vi "BIMS_Collector (2010_08).vi"() -> ()   [LabVIEW 2015]
doc: "This program is currently beta software. It is designed to address the data requirements defined primarily by the DHB Ballistic Test Report.\n\nThe general operation of this program is based on the Ballistics Version 2005 application developed internally by DuPont as a research tool for the Spruance Plant Ballistics Lab in Richmond, VA.\n\nPlease note that the original trigger control logic was modified and no longer depends on a safety interlock system to enable operation of a ballistic test.\n\nDuPont makes no warranties and assumes no liabilities in connection with any use of this program."
uses:
  <vilib>/addons/database/NI_Database_API.lvlib
  <vilib>/addons/database/Connection.llb/Conn Execute.vi
  <vilib>/addons/database/Recordset.llb/Rec Destroy - Connection.vi
  <vilib>/Utility/config.llb/NI_LVConfig.lvlib
  <vilib>/Utility/config.llb/Write Key (I32).vi
  Shot Record.ctl
  BIMS_Collector Globals.vi
  Collector State.ctl
  DataSource.ctl
  <vilib>/registry/registry.llb/Registry RtKey.ctl
  <vilib>/Utility/config.llb/Write Key (String).vi
  <vilib>/addons/database/Connection.llb/DB Tools Open Connec (Path).vi
panel:
  out "Loading":u16(ring)
  in  "runtimeMenusVisible":bool=TRUE
  in  "diagPageVisible":bool
  in  "RESET All":bool
  out "ConfigName":string
  out "TimeNow":string
  in  "EXIT":bool
  in  "mainTabCntrl":enum32{"Setup", "Measure", "History", "System"}(tab)=enum."System"
  in  "SampleEntryTabCntrl":enum32{"Environment", "Sample"}(tab)
  in  "ThreatDetails":u16(ring) caption="Detail"
  in  "ThreatGroups":u16(ring) caption="Group" items=["", "RCC"]
  in  "PowderTypes":u16(ring) caption="Type"
  in  "Ballisticians":u16(ring) caption="Ballistician"
  in  "Recorders":u16(ring) caption="Recorder"
  in  "Shooters":u16(ring) caption="Shooter"
  in  "Methods":u16(ring) caption="Method"
  in  "RoomT":sgl caption="Temperature (° F)" format="%.1f"
  in  "RoomHum":sgl caption="Humidity (%)" min=0 max=100 format="%.1f"
  in  "SampleBackings":u16(ring)=3 caption="Type"
  in  "clayCalArray":i16[](array[numeric])=[0, 0, 0, 0, 0] caption="Calibration (mm)" min=0 max=99 format="%02.0f"
  out "clayAverage":sgl caption="Clay Average (mm)" format="%#.1f"
  in  "clayTemp":sgl caption="Clay Temp (° F)" format="%.1f"
  out "threatDetails":T1 caption="Description"
  in  "SampleClamping":u16(ring) caption="Clamping"
  in  "Sample SubTabCntrl":T2(tab)
  in  "SampleID":string caption="Sample ID"
  in  "SampleDimensions":u16(ring) caption="Dimensions"
  in  "ModelMfrs":u16(ring) caption="Manufacturer" items=["DuPont Experimental"]
  in  "SampleTypes":u16(ring) caption="Sample Type"
  in  "Submitters":u16(ring) caption="Submitter"
  in  "ProjectID":string caption="Project ID"
  in  "BackLayers":i32 caption="# of Layers" min=0 max=99 step=5
  in  "FrontLayers":i32 caption="# of Layers" min=0 max=99 step=5
  in  "BackLayer":u16(ring) caption="Back Layer"
  in  "FrontLayer":u16(ring) caption="Front Layer"
  out "totalNumLayers":i32 caption="Total # of Layers" min=0 max=100 step=5
  out "totalBAW":sgl caption="Total BAW (psf)" format="%.2f"
  in  "LayerTabControl":enum32{"1", "2", "3", "4", "5", "6"}(tab) caption="Inner Layers"
  out "fab1_totalWt":sgl caption="Fab1 Wt" min=0 max=99 step=5 format="%.2f"
  out "SampleAttribs_1":T3 caption="fabricAttribs_1"
  in  "Layer_1":T4 caption="Fabric #1" {"plyNum" min=0 max=99 step=5}
  in  "SampleStyle_1":u16(ring) items=["", "S-706G"]
  in  "Mfr_1":u16(ring) caption="vendor" items=["", "DuPont"]
  in  "layerStitch_1":u16(ring) caption="Stitch" items=["", "1-inch quilt", "2-inch quilt", "Corner Bartack", "Corners", "Custom (Panel)", "Custom (Vest)", "Diamond", "Edge", "n/a", "Normal"]
  out "fab2_totalWt":sgl caption="Fab2 Wt" min=0 max=99 step=5 format="%.2f"
  out "SampleAttribs_2":T3 caption="fabricAttribs_2"
  in  "Layer_2":T4 caption="Fabric #2" {"plyNum" min=0 max=99 step=5}
  in  "SampleStyle_2":u16(ring)
  in  "Mfr_2":u16(ring) caption="vendor" items=["", "DuPont"]
  in  "layerStitch_2":u16(ring) caption="Stitch" items=["", "1-inch quilt", "2-inch quilt", "Corner Bartack", "Corners", "Custom (Panel)", "Custom (Vest)", "Diamond", "Edge", "n/a", "Normal"]
  out "fab3_totalWt":sgl caption="Fab3 Wt" min=0 max=99 step=5 format="%.2f"
  out "SampleAttribs_3":T3 caption="fabricAttribs_3"
  in  "Layer_3":T4 caption="Fabric #3" {"plyNum" min=0 max=99 step=5}
  in  "SampleStyle_3":u16(ring)
  in  "Mfr_3":u16(ring) caption="vendor" items=["", "DuPont"]
  in  "layerStitch_3":u16(ring) caption="Stitch" items=["", "1-inch quilt", "2-inch quilt", "Corner Bartack", "Corners", "Custom (Panel)", "Custom (Vest)", "Diamond", "Edge", "n/a", "Normal"]
  out "fab4_totalWt":sgl caption="Fab4 Wt" min=0 max=99 step=5 format="%.2f"
  out "SampleAttribs_4":T3 caption="fabricAttribs_4"
  in  "Layer_4":T4 caption="Fabric #4" {"plyNum" min=0 max=99 step=5}
  in  "SampleStyle_4":u16(ring)
  in  "Mfr_4":u16(ring) caption="vendor" items=["", "DuPont"]
  in  "layerStitch_4":u16(ring) caption="Stitch" items=["", "1-inch quilt", "2-inch quilt", "Corner Bartack", "Corners", "Custom (Panel)", "Custom (Vest)", "Diamond", "Edge", "n/a", "Normal"]
  out "fab5_totalWt":sgl caption="Fab5 Wt" min=0 max=99 step=5 format="%.2f"
  out "SampleAttribs_5":T3 caption="fabricAttribs_5"
  in  "Layer_5":T4 caption="Fabric #5" {"plyNum" min=0 max=99 step=5}
  in  "SampleStyle_5":u16(ring)
  in  "Mfr_5":u16(ring) caption="vendor" items=["", "DuPont"]
  in  "layerStitch_5":u16(ring) caption="Stitch" items=["", "1-inch quilt", "2-inch quilt", "Corner Bartack", "Corners", "Custom (Panel)", "Custom (Vest)", "Diamond", "Edge", "n/a", "Normal"]
  out "fab6_totalWt":sgl caption="Fab6 Wt" min=0 max=99 step=5 format="%.2f"
  out "SampleAttribs_6":T3 caption="fabricAttribs_6"
  in  "Layer_6":T4 caption="Fabric #6" {"plyNum" min=0 max=99 step=5}
  in  "SampleStyle_6":u16(ring)
  in  "Mfr_6":u16(ring) caption="vendor" items=["", "DuPont"]
  in  "layerStitch_6":u16(ring) caption="Stitch" items=["", "1-inch quilt", "2-inch quilt", "Corner Bartack", "Corners", "Custom (Panel)", "Custom (Vest)", "Diamond", "Edge", "n/a", "Normal"]
  in  "SampleCoverings":u16(ring) caption="Sample Covering" items=["None", "RipStop", "Plastic bag", "Other"]
  in  "Assemblers":u16(ring) caption="Technician"
  in  "Thickness":dbl caption="Thickness (in)" format="%.3f"
  in  "totalSampleWt":sgl caption="Total Weight (lbs)" format="%.3f"
  in  "Comments":string caption="Remarks (optional):"
  in  "TestConditions":u16(ring) caption="Sample Condition"
  in  "shotsTabCntrl":T5(tab)
  in  "Frag Rod":sgl format="%.1f"
  in  "MeasSrc":T6=enum."Screens" caption="Source"
  in  "Drag Corrected":bool=TRUE
  in  "ARM":bool
  in  "readyClock":bool caption="Clock"
  out "Impact/speed":sgl caption="Chronograph 1" min=0 max=10000 step=0.1 format="%.1f"
  out "SHOT STATUS":u16(ring) caption="Penetration" items=["Partial", "Complete"]
  out "residual/speed":sgl caption="Residual" min=0 max=10000 step=0.1 format="%.1f"
  out "SUBMIT DATE/TIME":string
  out "BACKFACE DEPTH":sgl caption="Backface\nDepth" min=0 max=200 step=5
  in  "MeasVelScrnSet1":sgl caption="Set #1" min=0 max=10000 step=0.1 format="%.1f"
  in  "Current/sthotstatus":u16(ring) caption="Penetration" items=["Partial", "Complete"]
  in  "Current/residual/speed":sgl caption="Residual Set" min=0 max=10000 step=0.1 format="%.1f"
  in  "currentDateTime":string caption="Date/Time"
  in  "MeasVelScrnSet2":sgl caption="Set #2" min=0 max=1000000 step=0.1 format="%.1f"
  out "%_Difference":sgl caption="% Vel Diff" format="%.3f"
  in  "backdepth":sgl caption="BF Depth"
  out "Redundant/speed":sgl caption="Chronograph 2" min=0 max=10000 step=0.1 format="%.1f"
  out "Current/avg/speed":sgl caption="Average" min=0 max=1000000 step=0.1 format="%.1f"
  out "Avg/speed":sgl caption="Average" min=0 max=10000 step=0.1 format="%.1f"
  out "SafetyInterlock":cluster{"ARMED":bool}
  out "DC_ factor":sgl=1.0 caption="DC Factor" format="%.4f"
  in  "Barrel Temp":sgl format="%.1f"
  in  "Shot Description":string caption="Description (optional)"
  in  "Powder Loading":sgl caption="Powder Load" min=0 max=100 step=0.1 format="%.3f"
  in  "Shot Angle":u16 max=90 step=1
  out "Projectile Mass":sgl caption="Projectile Mass (grains)" min=0 step=1
  in  "N.I.J":u16(ring) items=["n/a", "PASS", "FAIL"]
  out "Device S/N":string
  in  "addShot":bool caption="RANGE SETUP must be selected before shots can be added."
  in  "loadingUnits":enum32{"grams", "grains"}(radio)
  out "instruct_addShot":string="RANGE SETUP and THREAT must be selected before shots can be added."
  out "Set#1 Separation":sgl=4.0 caption="Outer" format="%.2f"
  out "Set#2 Separation":sgl=4.0 caption="Inner" format="%.2f"
  out "saveReq":string="Number of layers in sample ply specification and number of shots in shots table must be greater than 0 to enable saving."
  in  "VsVr Report":bool caption="Report"
  out "Table of Shots":string[][](table) caption="Shot Table"
  in  "MC Listbox of Shots":i32(listbox)
  in  "saveShots":bool
  in  "clearShots":bool
  out "highPartial":i32 caption="High Partial" min=0 max=10000 step=1
  out "lowComplete":i32 caption="Low Complete" min=0 max=10000 step=1
  out "rangeOfResults":i32 caption="Range of Results" min=0 max=10000 step=1
  out "zmr 2":sgl caption="Low C minus High P" format="%.1f"
  out "computed_V50":sgl caption="V50" format="%.1f"
  out "Pairs":i16 min=0 max=100 step=1
  in  "reportV50":bool caption="Report"
  in  "maxDev":sgl=125.0 caption="Max Deviation" min=0 max=300 step=25
  in  "undoLastShot":bool
  in  "deleteShot":bool
  in  "nextShot":bool
  in  "SHOTS":T7[](array[typedef]) {"Frag Rod" format="%.1f"; "UncorrectedAvgVel_PB" format="%.1f"; "UncorrectedRed_PB" format="%.1f"; "strikeVel_PB" format="%.1f"; "velLoss_PB" format="%.1f"; "avgVel_PB" format="%.1f"; "Redundant_Velocity" format="%.1f"; "Energy Loss (J)" format="%.3e"; "Projectile Mass" min=0 step=1 format="%.4f"; "Corrected residual" format="%.2f"; "Uncorrected Residual" format="%.1f"; "Corrected Impact" format="%.2f"; "Uncorrected Impact" format="%.1f"; "Shot Angle" max=90 step=1; "SHOT STATUS" items=["Partial", "Complete"]; "IMPACT VELOCITY" min=0 max=10000 step=0.1 format="%.1f"; "Barrel Temperature" format="%.1f"; "Powder Loading" format="%.4f"; "RESIDUAL  VELOCITY" min=0 max=10000 step=0.1 format="%.1f"}
  out "velProfile":cluster{dbl, dbl}[](graph) caption="Shot Velocity Measurement Profile"
  out "velCompProf":cluster{"vStrike":dbl, "vA":dbl} caption="Velocity in fps\n(computed)"
  out "velMeasProf":T8 caption="Velocity in fps\n(measured)"
  out "relativeTime":cluster{"ts2":dbl, "ts3":dbl, "ts1":dbl} caption="Relative time\n(microsec)"
  out "displacement":T9={"ds_v2"=6.75, "ds2"=5.0833, "ds_vB"=4.9167, "ds3"=4.75, "ds_vAvg"=6.9167, "ds_v1"=7.0833, "ds1"=8.75, "ds_vA"=8.9167, "ds0"=9.0833} caption="Distance from\ntarget (ft)" {"ds0" format="%_4g"; "ds_vA" format="%_4g"; "ds1" format="%_4g"; "ds_v1" format="%_4g"; "ds_vAvg" format="%_4g"; "ds3" format="%_4g"; "ds_vB" format="%#_4g"; "ds2" format="%#_4g"; "ds_v2" format="%_4g"}
  out "arrIDC":dbl[](array[numeric]) caption="Instantaneous Drag Coefficient"
  in  "rangeSetup":u16(ring)=1 caption="Range Dimensions" items=["Short (small frag)", "Standard (handgun)", "Long (rifle)"]
  out "mid_to_targ_dist":sgl=5.0 caption="Mid To Target (ft)"
  in  "historyTabCntrl":enum32{"Powder Loading", "Panel Search"}(tab)=enum."Panel Search"
  in  "Threat.freeTxt":string caption="Threat"
  in  "Powder.freeTxt":string caption="Powder"
  in  "QueryLoad":bool
  in  "lkupEndDate":timestamp caption="End Date" format="%<%x>T"
  in  "lkupStartDate":timestamp caption="Begin Date" format="%<%x>T"
  out "Vel.vs.Loading":cluster{dbl[], dbl[]}(graph)
  out "v50_table":string[][](table)
  in  "maxRecs":u16=1001 caption="Max # of SHOT Records" min=1 max=10000 step=100
  out "ActualNumRecs":i32=1001 caption="Actual # Returned"
  in  "ThreatSize_0":u16(ring) caption="Threat Size" items=["", "2"]
  in  "panelSearch":bool
  in  "Mfr_0":u16(ring) caption="Manufacturer" items=["", "DuPont"]
  in  "SampleStyle_0":u16(ring) caption="Sample Style"
  in  "srchParams":T10={"maxPanels"=1001, "lkupPanelStartDate"=timestamp(0 s since 1904-01-01), "lkupPanelEndDate"=timestamp(3376658114.0909824 s since 1904-01-01)} {"lkupPanelEndDate" format="%<%x>T"; "lkupPanelStartDate" format="%<%x>T"; "maxPanels" min=1 max=10000 step=100}
  out "actualNumPanels":i32 caption="Actual # Returned"
  out "pastPanels":string[][](table)
  in  "Record #":i32=1 min=0 max=0
  in  "reportV50_History":bool
  out "SampleAttribs_0":T11 caption="fabricAttribs_1"
  in  "Requestors_0":u16(ring) caption="Submitter"
  in  "aboutTabCntrl":T12(tab)
  in  "RefreshMetadata":bool
  out "LastShot":i32 caption="Shot"
  out "LastSample":i32 caption="Sample"
  in  "PublishNewRecords":bool
  in  "Folder":string="esvrs11" caption="Publish Folder"
  in  "clearErrors":bool
  in  "useBMC":bool caption="Use Message Center?"
  in  "Server":string="esvrs11"
  in  "Site":string="ICE1"
  in  "TestStandards":u16(ring)=2 caption="Standard" items=["n/a", "NIJ 0101.04", "MIL-STD-662F"]
  in  "WeaponTypes":u16(ring) caption="Weapon" items=["", "Universal Receiver", "Other"]
  in  "processShots":bool
  out "DIO":u32=21 format="%.0b"
  in  "line direction map":i32=1792 format="%.0b"
  out "Corrected Average":sgl=1527.9313 format="%.2f"
  out "CorrectedVelScrnSet2":sgl=1551.8816 caption="Corrected Redundant" format="%.2f"
  out "conversion factor":sgl=0.3048037 format="%.5f"
  out "#_completes":i32
  out "#_partials":i32
  in  "percent warning":sgl=1.0 format="%.2f"
  in  "SoftwareVersion":dbl caption="Version" format="%.2f"
  out "impact/ID":u32=83886081 format="%.0x"
  out "residual/ID":u32=83951617 format="%.0x"
  out "Red/ID":u32=84017153 format="%.0x"
  out "correction coefficient":sgl format="%.8f"
  out "Corrected Residual":sgl=751.9905 format="%.2f"
  out "CorrectedVelScrnSet1":sgl=1503.981 format="%.2f"
  out "Barrel to Screen":sgl=7.8333 format="%.2f"
  in  "Set#1_to_Target":sgl=7.083333 format="%.2f"
  out "Residual/Separation":sgl=4.0 format="%.2f"
  in  "Residual/Target Dist":sgl=7.083333 format="%.2f"
  out "Z.M.R.":sgl min=0 step=0.1 format="%.1f"
  in  "old threat":u16
  out "Complete":sgl[](array[numeric]) format="%.2f"
  out "factor array":sgl[](array[numeric]) format="%.4f"
  out "Partial":sgl[](array[numeric]) format="%.2f"
  in  "DAQ Card":i16=1
  in  "Impact Timer":i16 min=0 max=3 step=1
  in  "Redundant Timer":i16=1 min=0 max=3 step=1
  in  "Residual  Timer":i16=2 min=0 max=3 step=1
  out "Impact factor":sgl=1.0 caption="Impact" min=0 max=1 format="%.5f"
  out "Residual factor":sgl=1.0 caption="Residual" min=0 max=1 format="%.5f"
  in  "Areal Density":dbl format="%.2f"
  in  "Areal density text":string
  in  "Fabric Description":string caption="Fabric Desc"
  in  "clayCalib":string="##-##-##-##-##" caption="Calibration"
  in  "lookupRec":bool caption="lookup"
  out "STOP (Shots MC LB)":bool=TRUE
  out "configPath":path=path "P:/Private/My Projects/AFS/BIMS/2008/BIMS_Collector.ini" caption="Configuration Path (INI)"
  in  "minV50":i32=1500 caption="Minimum V50"
  in  "Type of work":string="QC"
  in  "Threat":u16(ring) caption="Threat (long description)"
  out "massUnits":string="GRAMS" caption="Weight Units"
  out "lengthUnits":string="FOOT" caption="Distance Units"
  in  "SampleDescrip":u16(ring) caption="Misc. Sample Description (legacy)"
  in  "serialNum":string caption="Serial #"
  in  "Models":u16(ring) caption="Model #" items=["n/a"]
  in  "InterlockExists":bool=TRUE caption="Safety Interlock Hardware Exist?"
  in  "ScreenSetAvgg":bool caption="Average Screen Sets?"
  in  "Sort by AVG":bool=TRUE caption="Sort shots by average velocity"
  in  "useBallisitican":bool=TRUE caption="Use Ballistician field in Setup?"
  in  "useRecorder":bool caption="Use Recorder field in Setup?"
  in  "useShooter":bool caption="Use Shooter field in Setup?"
  out "SMErr":errorcluster
  out "U/I EvErr":errorcluster
  out "booleanDump":bool
  out "GrainSize":u16 caption="Grain"
  in  "LayerStitchTypes":u16(ring) caption="Stitch" items=["", "Corners"]
  # "Effectively restarts the application from scratch, as if the user pressed the EXIT button and then restarted the application."
  # "Configured for"
  # "Threat"
  # "*"
  # "*"
  # "Test"
  # "Powder"
  # "*"
  # "Personnel"
  # "Room"
  # "*"
  # "Backing"
  # "*"
  # "*"
  # "*"
  # "Body Side"
  # "Strike Face"
  # "Layer"
  # "Mfr"
  # "Style"
  # "# of Plies"
  # "Lot"
  # "Roll"
  # "Stitch"
  # "Internal ID"
  # "Fiber"
  # "Denier"
  # "Construction"
  # "Weave"
  # "Finish"
  # "Basis weight (oz/yd²)"
  # "Yarn Merge"
  # "Total Weight"
  # "*"
  # "*"
  # "*"
  # "1"
  # "2"
  # "3"
  # "4"
  # "5"
  # "6"
  # "Required"
  # "*"
  # "Timing System"
  # "Shot Parameters"
  # "cm"
  # "deg"
  # "degF"
  # "Velocity Measurements"
  # "Observations"
  # "Screens\nSeparation"
  # "Ft"
  # "Table Functions"
  # "Summary"
  # "Reports"
  # "Test Record"
  # "Edit Shot Records"
  # "Corrected"
  # "Shot #"
  # "t0"
  # "0"
  # "S Strike"
  # "0"
  # "Internal ID#"
  # "Fiber"
  # "Denier"
  # "Pick"
  # "Weave"
  # "Finish"
  # "oz/yd²"
  # "Asset"
  # "DuPont Ballistics Information Management System\n\nBIMS\nEnterprise Edition\n\n\nSample Performance\nData Collector\n\nAugust 2010"
  # "DuET Measurement System Technologies\nDUCOM 8 695-2330 for technical support\n\nDuPont Company"
  # "Last Assigned\nRecord Numbers"
  # "Deployment Configuration"
  # "Data items support Point Blank requirements:"
  # "Correction Factors"
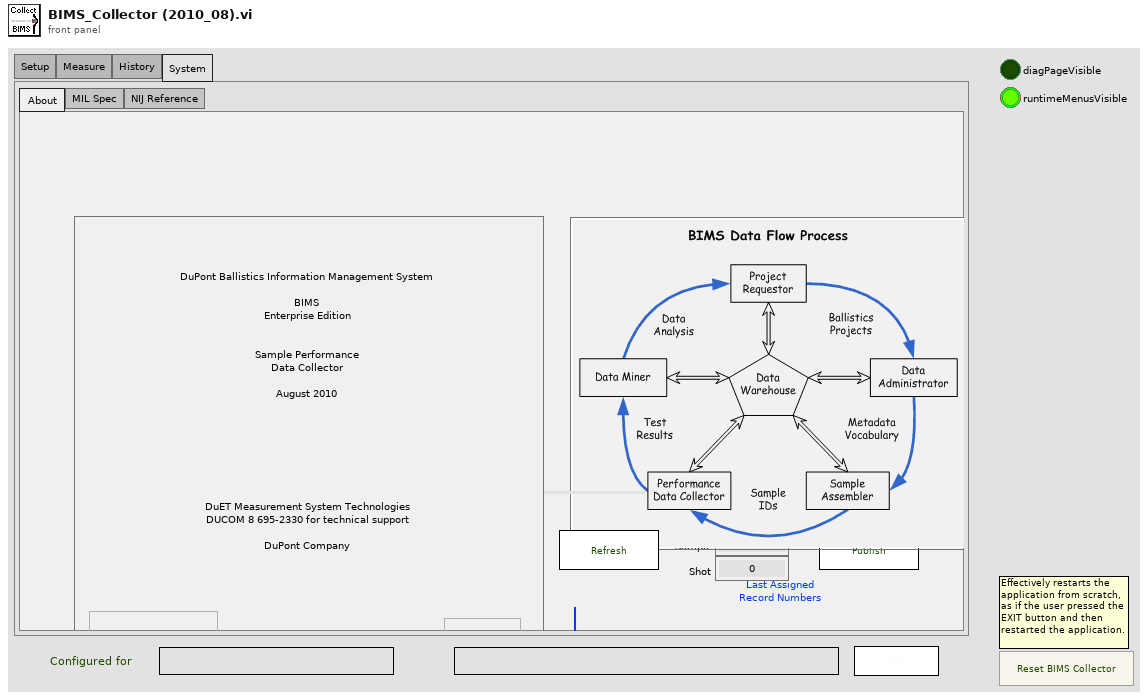
[diagram p1: front panel]
types:
  T1 = cluster{"barrelLength":string, "dragCorrection":string, "detailDescription":string, "barrelCaliber":string, "grainSize":string, "Make":string, "Model":string}
  T2 = enum32{"General Specification", "Ply Specification", "Preparation"}
  T3 = cluster{"Fabric.fiber":string, "Fabric.denier":string, "pick":string, "weave":string, "finish":string, "ozPerYd2":string, "fabricID_DHB":string, "yarnMerge":string}
  T4 = cluster{"plyNum":i32, "LotNum":string, "RollNum":string}
  T5 = enum32{"Ready-Aim-Fire", "Shots Table", "Edit", "Instantaneous DC"}
  T6 = typedef "DataSource.ctl" = enum16{"Simulated", "Radar", "Screens"}
  T7 = typedef "Shot Record.ctl" = cluster{"Uncorrected Impact":sgl, "Uncorrected Residual":sgl, "avgVel_PB":sgl, "IMPACT VELOCITY":sgl, "RESIDUAL  VELOCITY ":sgl, "Shot Description":string, "Powder Loading ":sgl, "Barrel Temperature":sgl, "TIME / DATE":string, "shot order":i32, "SHOT STATUS":u16, "Shot Angle":u16, "Corrected Impact":sgl, "Corrected residual":sgl, "Projectile Mass":sgl, "usedv50":bool, "Energy Loss (J)":sgl, "BackFace\nDepth":sgl, "BackFace\nDiameter":sgl, "Redundant_Velocity":sgl, "velLoss_PB":sgl, "strikeVel_PB":sgl, "UncorrectedRed_PB":sgl, "CorrectedRed_PB":sgl, "UncorrectedAvgVel_PB":sgl, "V50userExcl":bool, "Frag Rod":sgl}
  T8 = cluster{"v2":dbl, "vB":dbl, "vOuter":dbl, "v1":dbl, "vA":dbl, "vInner":dbl}
  T9 = cluster{"ds_v2":dbl, "ds2":dbl, "ds_vB":dbl, "ds3":dbl, "ds_vAvg":dbl, "ds_v1":dbl, "ds1":dbl, "ds_vA":dbl, "ds0":dbl}
  T10 = cluster{"maxPanels":u16, "lkupPanelStartDate":timestamp, "lkupPanelEndDate":timestamp}
  T11 = cluster{"Fabric.fiber":string, "Fabric.denier":string, "pick":string, "weave":string, "finish":string, "ozPerYd2":string, "fabricID_DHB":string, "asset":string}
  T12 = enum32{"About ", "MIL Spec", "NIJ Reference", "Internal Use"}
  T13 = typedef "Collector State.ctl" = enum16{"POLL", "INITIALIZE", "V50 Report or GET Record", "VsVr Report", "SAVE SHOTS", "ADD SHOT", "CLEAR SHOTS", "NEXT SHOT", "DELETE SHOT", "READY CLOCK", "PROC SHOTS", "CHECK DAQ"}
  T14 = typedef "Collector State.ctl" = enum16{"POLL", "INITIALIZE", "V50 Report or GET Record", "VsVr Report", "SAVE SHOTS", "ADD SHOT", "CLEAR SHOTS", "NEXT SHOT", "DELETE SHOT", "PROCESS SHOTS", "READY CLOCK", "CHECK DAQ"}
  T15 = enum8{"Enabled", "Disabled", "Disabled and Grayed Out"}
  T16 = enum32{"Page Enabled", "Page Disabled", "Page Disabled & Grayed"}
  T17 = typedef "Registry RtKey.ctl" = enum32{"HKEY_CLASSES_ROOT", "HKEY_CURRENT_USER", "HKEY_LOCAL_MACHINE", "HKEY_USERS", "HKEY_PERFORMANCE_DATA", "HKEY_CURRENT_CONFIG", "HKEY_DYN_DATA"}
  T18 = cluster{"[0]":string, "[1]":string, "[2]":string, "[3]":string, "[4]":string, "[5]":string, "[6]":string, "[7]":string, "[8]":string, "[9]":string}[]
  T19 = cluster{"[0]":string, "[1]":string, "[2]":string, "[3]":string, "[4]":string, "[5]":string, "[6]":string, "[7]":string, "[8]":string}[]
  T20 = cluster{"Fabric.fiber":string, "Fabric.denier":string, "pick":string, "weave":string, "finish":string, "ozPerYd2":string, "fabricID_DHB":string, "yarnMerge":string}[]
  T21 = cluster{"Uncorrected Impact":bool, "Uncorrected Residual":bool, "avgVel_PB":bool, "IMPACT VELOCITY":bool, "RESIDUAL  VELOCITY ":bool, "Shot Description":bool, "Powder Loading ":bool, "Barrel Temperature":bool, "TIME / DATE":bool, "shot order":bool, "SHOT STATUS":bool, "Shot Angle":bool, "Corrected Impact":bool, "Corrected residual":bool, "Projectile Mass":bool, "usedv50":bool, "Energy Loss (J)":bool, "BackFace\nDepth":bool, "BackFace\nDiameter":bool, "Redundant_Velocity":bool, "velLoss_PB":bool, "strikeVel_PB":bool, "UncorrectedRed_PB":bool, "CorrectedRed_PB":bool, "UncorrectedAvgVel_PB":bool, "V50userExcl":bool, "Frag Rod":bool}
  T22 = cluster{"SampleTypes":refnum<vi>, "SampleDescrip":refnum<vi>}
  T23 = cluster{"max dev":sgl, "residual separation":sgl, "Set#1 Separation":sgl, "Set#2 Separation ":sgl, "impact target dist":sgl, "resid target dist":sgl, "barrel screen dist":sgl, "midpt_to_target_dist":sgl}
  T24 = cluster{"fiber":string, "denier":string, "pick":string, "weave":string, "finish":string, "ozPerYd2":string, "internal_ID":string, "asset":string}[]
  T25 = cluster{"numOfPlies":i32, "LotNum":string, "RollNum":string}[]
  T26 = cluster{string, string, string, string, string, string, string, string, "clayCalib":string, string}
  T27 = cluster{string, string, string, string, string, string, string}
  T28 = cluster{"SampleID":string, "element":string, "Type of work":string, "serialNum":string, "element":string, string, string, string, "element":string, string}
  T29 = cluster{"SampleID":string, "element":string, string, string, string, "element":string}
  T30 = cluster{"[0]":string, "[1]":string, "[2]":string, "[3]":string, "[4]":string, "[5]":string, "[6]":string, "[7]":string, "[8]":string, "[9]":string}
  T31 = cluster{"[0]":string, "[1]":string, "[2]":string, "[3]":string, "[4]":string, "[5]":string, "[6]":string, "[7]":string, "[8]":string}
  T32 = cluster{"element":string, "element":string, "grainSize":string, "element":string, "barrelLength":string, string, "element":string, "element":string, "element":string}
  T33 = cluster{"element":string, "grainSize":string, "element":string, "barrelLength":string, string, "element":string}
  T34 = typedef "NI_Database_API.lvlib/Conn ObjectReference.ctl" = refnum<k1>
  T35 = typedef "NI_Database_API.lvlib/Rec ObjectReference.ctl" = refnum<k1>
  T36 = typedef "NI_LVConfig.lvlib/Config Data RefNum.ctl" = refnum<k1>
  T37 = cluster{"task ID out":u32, "task ID out":u32, "task ID out":u32}
  T38 = enum32{"invalid app kind", "Development System", "Run Time System", "Student Edition", "Embedded LabVIEW", "Evaluation", "Custom"}
  T39 = typedef "LVRowAndColumnTypeDef.ctl" = cluster{"Row":i32, "Column":i32}
  T40 = cluster{"barrelLength":string, "dragCoefficient":string, "detailDescription":string, "barrelCaliber":string, "grainSize":string, "Make":string, "Model":string}
  T41 = cluster{"fiber":string, "denier":string, "construction":string, "weave":string, "finish":string, "ozPerYd2":string, "fabricStyle_DHB":string, "yarnMerge":string}
  T42 = cluster{"plyNum":i32, "LotNum":string, "RollNum":string}[]
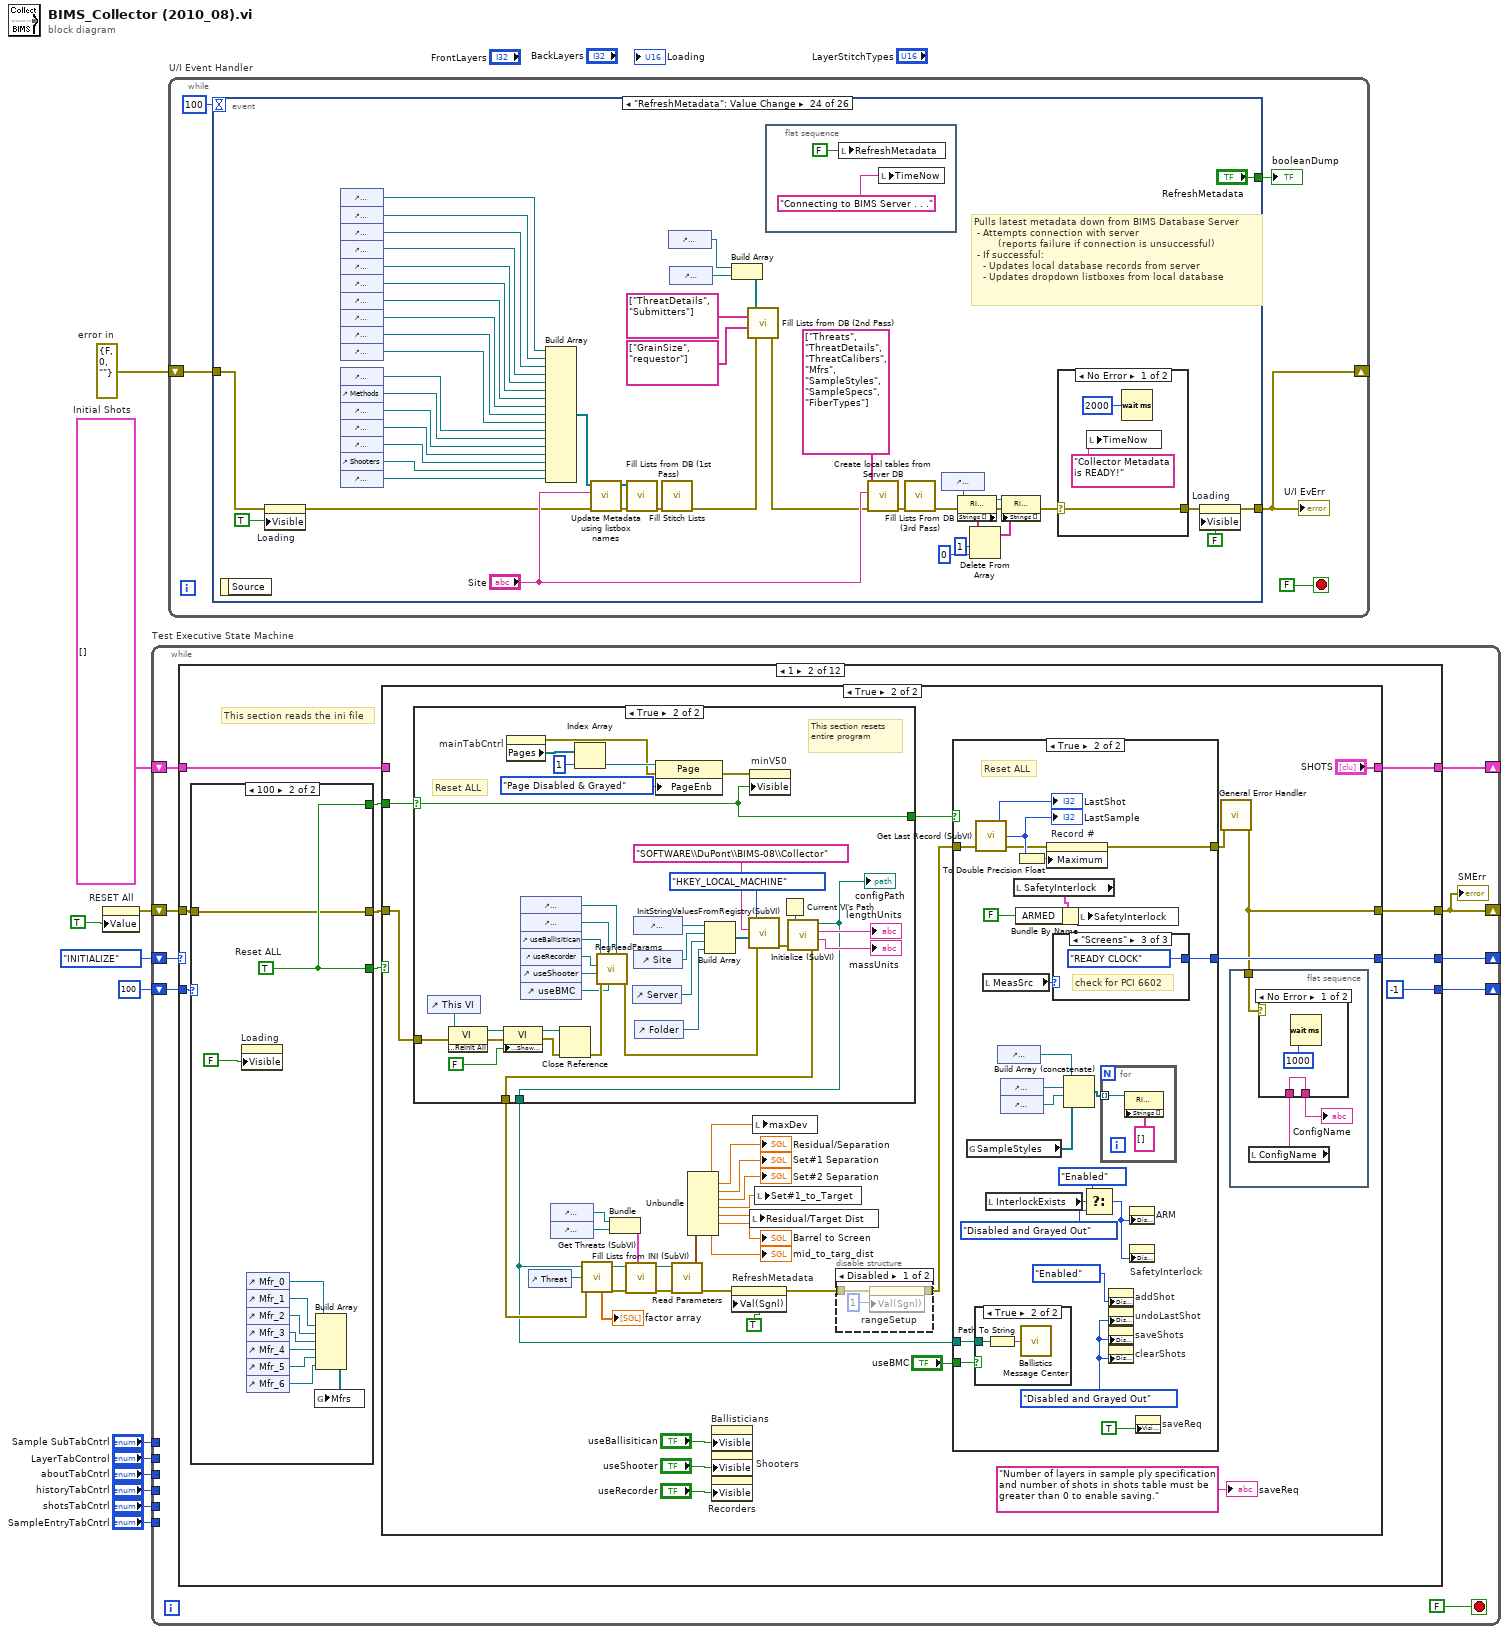
[diagram p0: block diagram]
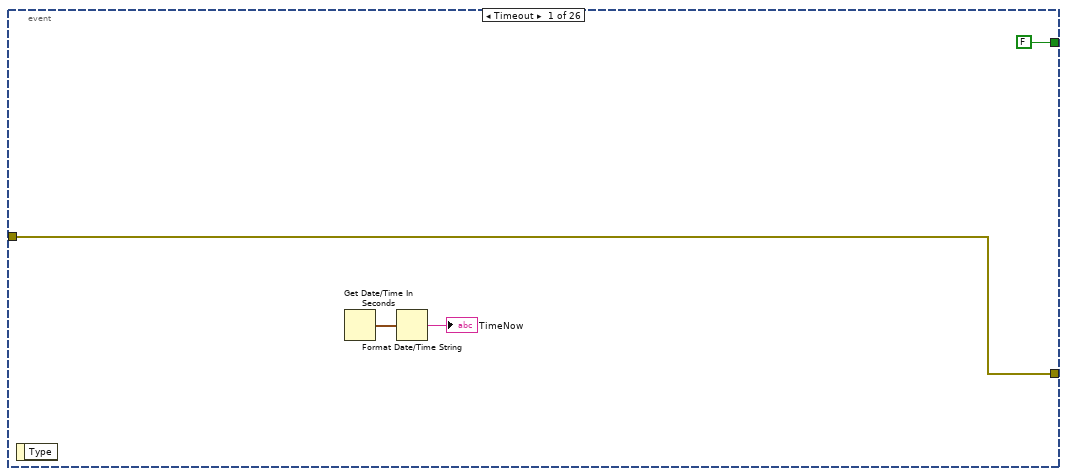
[diagram p2: hidden frame]
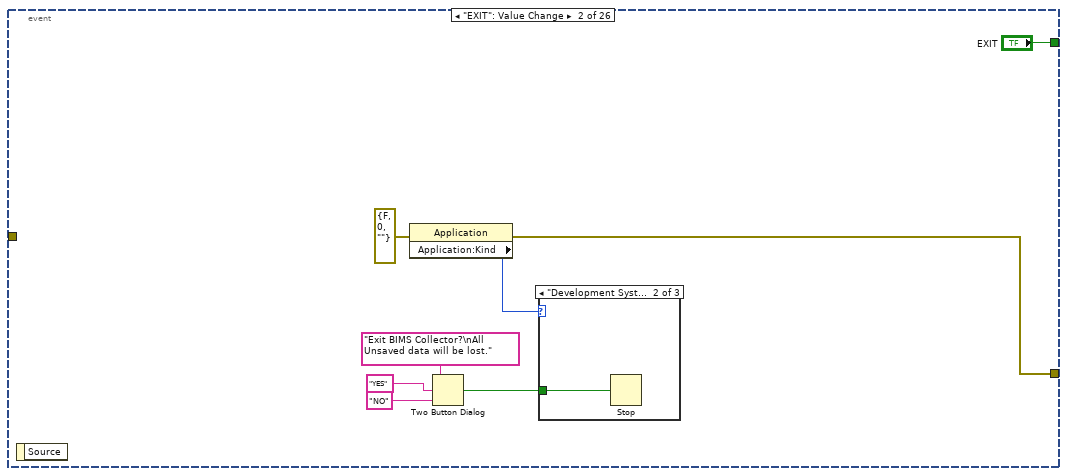
[diagram p3: hidden frame]
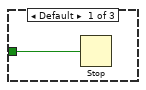
[diagram p4: hidden frame]
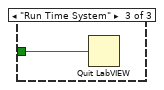
[diagram p5: hidden frame]
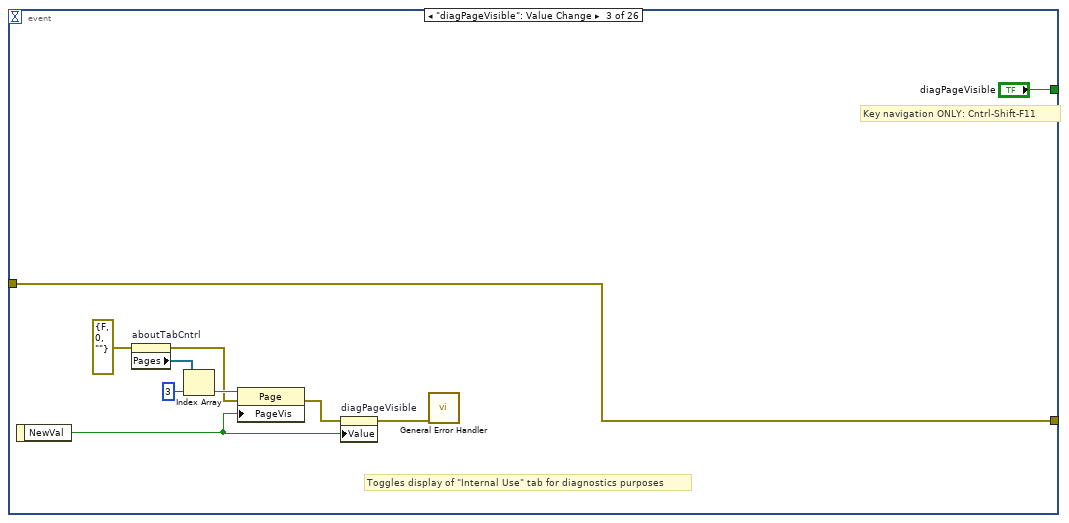
[diagram p6: hidden frame]
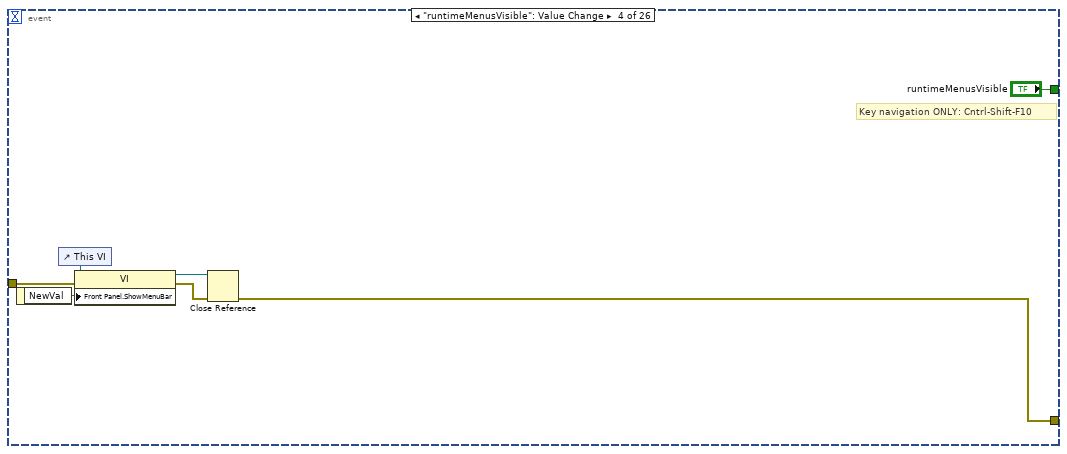
[diagram p7: hidden frame]
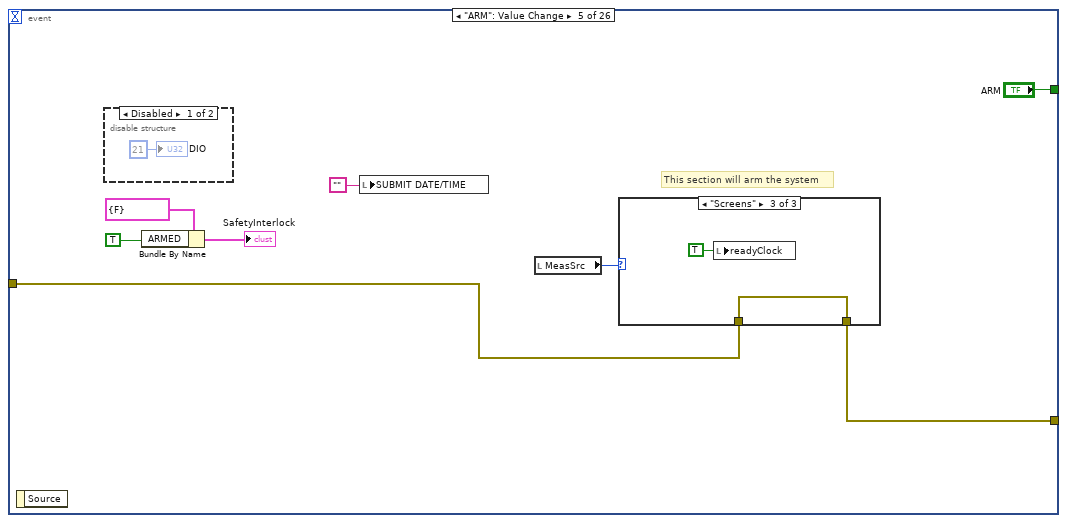
[diagram p8: hidden frame]
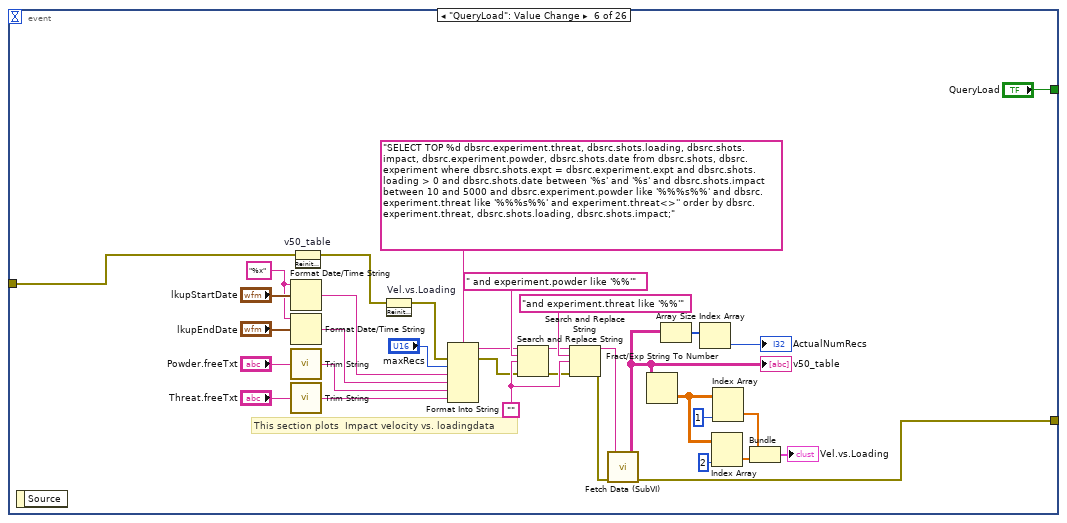
[diagram p12: hidden frame]
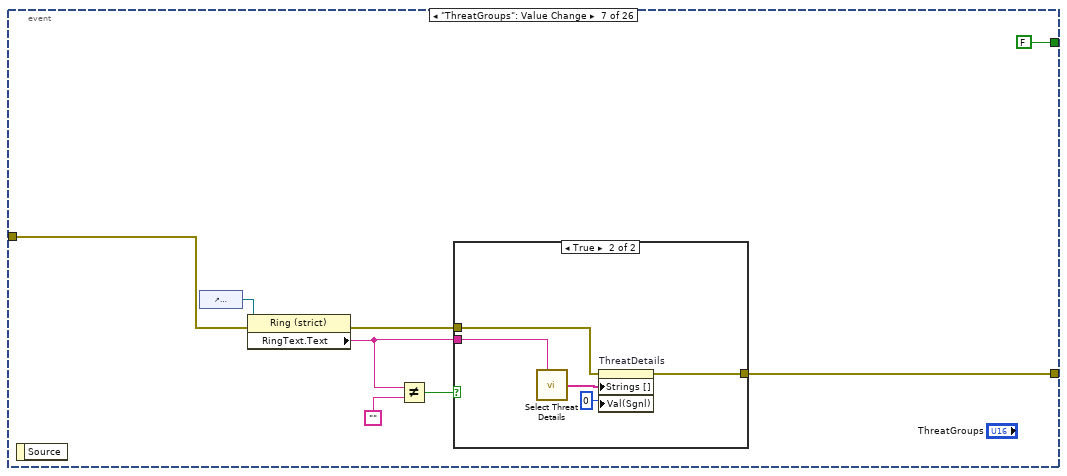
[diagram p13: hidden frame]
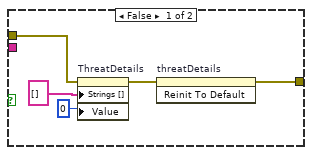
[diagram p14: hidden frame]
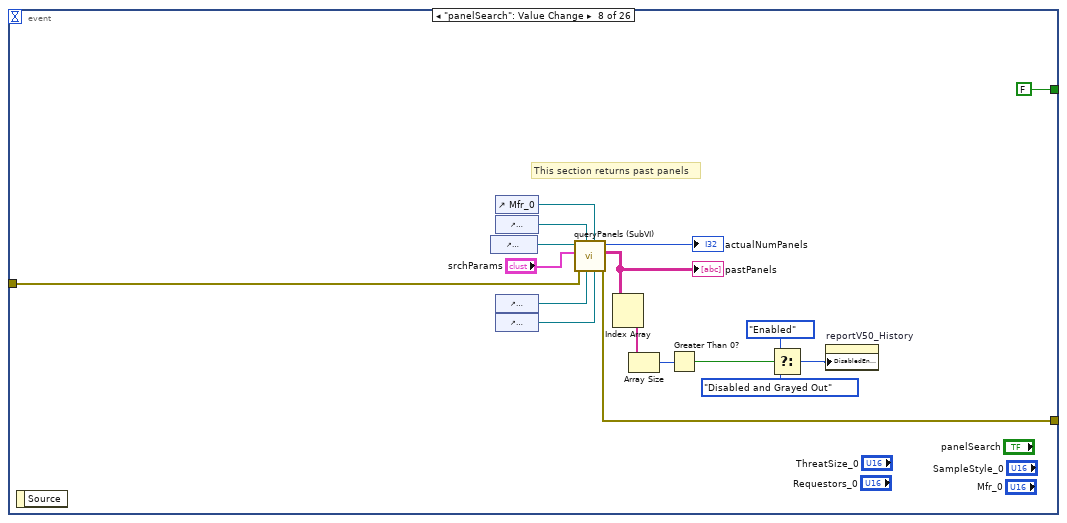
[diagram p15: hidden frame]
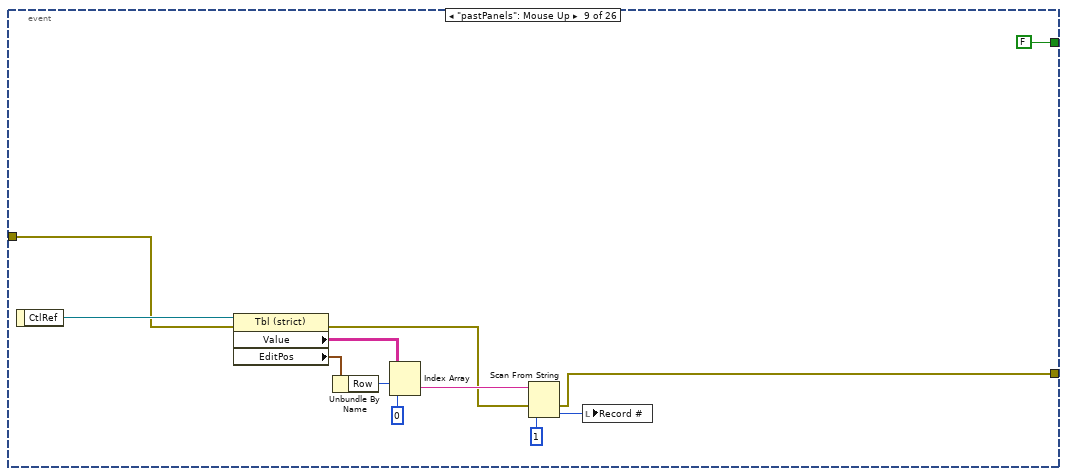
[diagram p16: hidden frame]
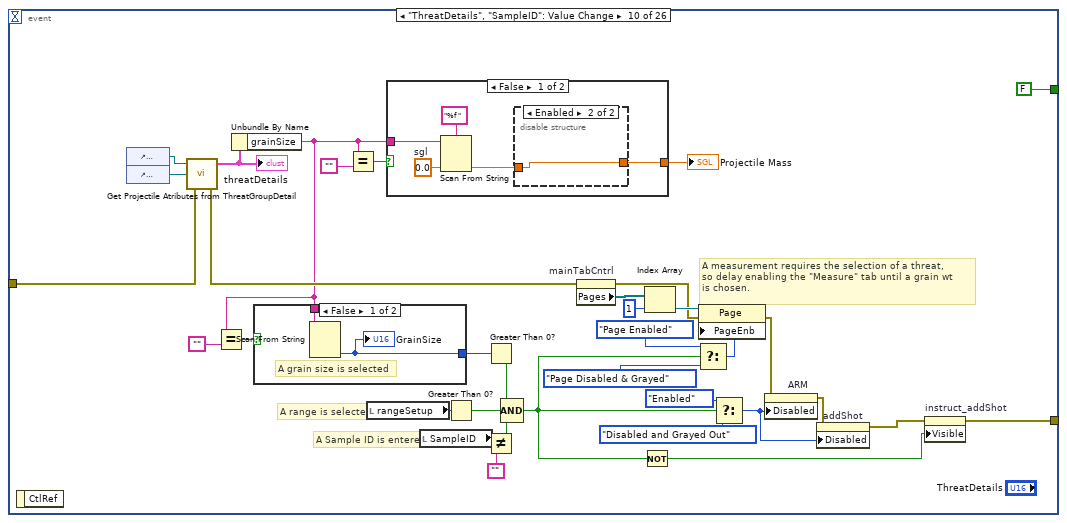
[diagram p17: hidden frame]
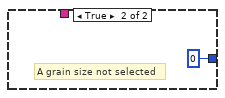
[diagram p18: hidden frame]
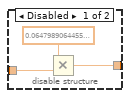
[diagram p19: hidden frame]
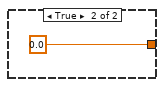
[diagram p20: hidden frame]
diagram:
  w7 = errorcluster {"status"=FALSE, "code"=0, "source"=""}  # error in
  w8 = T7[] []  # Initial Shots
  n1 = property on="RESET All" class="Bool (strict)"("Value"=TRUE ("RESET")) -> (error out=w10:errorcluster)  [unwired: 2 in, 1 out]
  n2 = while "Test Executive State Machine" {
    shift-left: 100 -> [w18]
    shift-right: [w19] -> _
    shift-left: Collector_State."INITIALIZE" ("progState") -> [w15]
    shift-right: [w20] -> _
    shift-right: [w16] -> _
    shift-left: w8 -> [w17]
    shift-right: [w13] -> _
    shift-left: w10 -> [w14]
    tunnel: "LayerTabControl" -> [_]
    tunnel: "aboutTabCntrl" -> [_]
    tunnel: "historyTabCntrl" -> [_]
    tunnel: "SampleEntryTabCntrl" -> [_]
    tunnel: "Sample SubTabCntrl" -> [_]
    tunnel: "shotsTabCntrl" -> [_]
    stop <- FALSE stop-if-true
    n3 = case shown="1" w15 {
      tunnel: [w24 w144 Collector_State."POLL" ("progState") Collector_State."POLL" ("progState") w1094 Collector_State."PROCESS SHOTS" ("progState") Collector_State."POLL" ("progState") Collector_State."PROCESS SHOTS" ("progState") Collector_State."PROCESS SHOTS" ("progState") Collector_State."POLL" ("progState") Collector_State."POLL" ("progState") w1757] -> w20
      tunnel: [-1 -1 ("index of element") -1 ("index of element") -1 ("index of element") w1093 -1 ("index of element") -1 -1 ("index of element") -1 ("index of element") -1 -1 ("index of element") w1756] -> w19
      tunnel: w18 -> [_ w145 _ _ _ _ _ _ _ _ _ _]
      tunnel: w17 -> [w28 w143 w300 w841 w1087 w1350 w1395 w1418 w1424 w1477 w1529 w1760]
      tunnel: [w27 w142 w300 w841 w1086 w1337 w1399 w1417 w1423 w1477 w1533 w1760] -> w16
      tunnel: w14 -> [_ w138 w297 w839 w1089 w1345 w1391 w1407 w1419 w1473 w1528 w1751]
      tunnel: [w36 w139 w296 w838 w1088 w1343 w1391 w1405 w1420 w1472 w1527 w1752] -> w13
      frame 0, Default {
        w29 = Collector_State."POLL"  # progStateType
        w49 = TRUE  # element
        w52 = 4  # SAVE
        # "This section checks for any buttons, maintains routine check of the paramters"
        n4 = case shown="\"Measure\"" "mainTabCntrl" {
          tunnel: w28 -> [_ w108 _ _]
          frame "Setup", Default {
            n5 = control-ref of="layerStitch_1"() -> (w76:refnum<vi>)
            n6 = control-ref of="layerStitch_2"() -> (w75:refnum<vi>)
            n7 = control-ref of="layerStitch_3"() -> (w74:refnum<vi>)
            n8 = control-ref of="layerStitch_4"() -> (w73:refnum<vi>)
            n9 = control-ref of="layerStitch_5"() -> (w72:refnum<vi>)
            n10 = control-ref of="layerStitch_6"() -> (w71:refnum<vi>)
            n11 = control-ref of="SampleStyle_0"() -> (w69:refnum<vi>)
            n12 = control-ref of="SampleStyle_1"() -> (w90:refnum<vi>)
            n13 = control-ref of="SampleStyle_2"() -> (w91:refnum<vi>)
            n14 = control-ref of="SampleStyle_3"() -> (w92:refnum<vi>)
            n15 = control-ref of="SampleStyle_4"() -> (w93:refnum<vi>)
            n16 = control-ref of="SampleStyle_5"() -> (w94:refnum<vi>)
            n17 = control-ref of="SampleStyle_6"() -> (w95:refnum<vi>)
            n18 = Build Array(w69, w90, w91, w92, w93, w94, w95) -> (w88:refnum<vi>[])
            n19 = global write "BIMS_Collector Globals.vi" "SampleStyles"(w88) -> ()
            n20 = Build Array(w76, w75, w74, w73, w72, w71) -> (w77:refnum<vi>[])
            n21 = global write "BIMS_Collector Globals.vi" "LayerStitchTypeRefs"(w77) -> ()
            n22 = local read "SampleAttribs_1"() -> (w82:T3)
            n23 = local read "SampleAttribs_2"() -> (w84:T3)
            n24 = local read "SampleAttribs_3"() -> (w85:T3)
            n25 = local read "SampleAttribs_4"() -> (w86:T3)
            n26 = local read "SampleAttribs_5"() -> (w87:T3)
            n27 = local read "SampleAttribs_6"() -> (w83:T3)
            n28 = Build Array(w82, w84, w85, w86, w87, w83) -> (w81:T20)
            n29 = global write "BIMS_Collector Globals.vi" "SampleAttribs"(w81) -> ()
            n30 = local read "Fabric Description"() -> (w80:string)
            n31 = control-ref of="Mfr_0"() -> (w70:refnum<vi>)
            n32 = control-ref of="Mfr_1"() -> (w101:refnum<vi>)
            n33 = control-ref of="Mfr_2"() -> (w100:refnum<vi>)
            n34 = control-ref of="Mfr_3"() -> (w99:refnum<vi>)
            n35 = control-ref of="Mfr_4"() -> (w98:refnum<vi>)
            n36 = control-ref of="Mfr_5"() -> (w97:refnum<vi>)
            n37 = control-ref of="Mfr_6"() -> (w96:refnum<vi>)
            n38 = String Subset(string=w80, length (rest)=75 ("length (rest)")) -> (substring=w79:string)  [unwired: 1 out]
            n39 = Build Array(w70, w101, w100, w99, w98, w97, w96) -> (w89:refnum<vi>[])
            n40 = local write "Fabric Description"(w79) -> ()
            n41 = global write "BIMS_Collector Globals.vi" "Mfrs"(w89) -> ()
          }
          frame "Measure" {
            # "Disable and gray out the \"Save\" button\nIF the shot table has no shots, \nOR if there are no plies; otherwise, enable it."
            # "Disable and gray out the \"Clear Shots\" button\nIF the shot table has no shots; otherwise, enable it."
            n42 = Array Size(array=w108) -> (size(s)=w115:i32)
            n43 = Equal To 0?(x=w115) -> (x = 0?=w102:bool)
            n44 = property on="saveReq" class="Str"("Visible"=w102) -> ()  [unwired: 2 in, 2 out]
            n45 = Select(t=T15."Disabled and Grayed Out" ("Disabled"), s=w102, f=T15."Enabled" ("Disabled")) -> (s? t:f=w114:T15)
            n46 = Select(t=T15."Disabled and Grayed Out" ("Disabled"), s=w102, f=T15."Enabled" ("Disabled")) -> (s? t:f=w103:T15)
            n47 = property on="reportV50" class="Bool"("Disabled"=w103) -> ()  [unwired: 2 in, 2 out]
            n48 = property on="saveShots" class="Bool"("Disabled"=w103) -> ()  [unwired: 2 in, 2 out]
            n49 = property on="clearShots" class="Bool"("Disabled"=w114) -> ()  [unwired: 2 in, 2 out]
            n50 = local read "Shot Description"() -> (w111:string)
            n51 = String Subset(string=w111, length (rest)=30 ("length (rest)")) -> (substring=w109:string)  [unwired: 1 out]
            n52 = local write "Shot Description"(w109) -> ()
            "SHOT STATUS" <- "Current/sthotstatus"
            "BACKFACE DEPTH" <- "backdepth"
          }
          frame "History" {
          }
          frame "System" {
          }
        }
        n53 = Get Date/Time String(want seconds? (F)=TRUE) -> (date string=w34:string, time string=w35:string)  [unwired: 2 in]
        n54 = call <vilib>:"Space Constant.vi"() -> ("String"=w32:string)
        n55 = Concatenate Strings(w34, w32, w35) -> (w33:string)
        n56 = local write "currentDateTime"(w33) -> ()
        n57 = Or(x="undoLastShot", y="deleteShot") -> (x .or. y?=w47:bool)
        n58 = Or(x="reportV50", y="reportV50_History") -> (x .or. y?=w55:bool)
        n59 = flat-sequence {
          tunnel: [w68] -> w30
          frame #0 {
            n60 = Wait (ms)(milliseconds to wait=u32 200 ("millisecond timer value")) -> ()  [unwired: 1 out]
          }
          frame #1 {
            n61 = local read "SMErr"() -> (w68:errorcluster)
          }
        }
        n62 = Build Array("RESET All", w55, "VsVr Report", "saveShots", "addShot", "clearShots", "nextShot", w47, "processShots", "readyClock") -> (w50:bool[])
        n63 = Search 1D Array(1D array=w50, element=w49) -> (index of element=w60:i32)  [unwired: 1 out]
        n64 = Increment(x=w60) -> (x+1=w61:i32)
        n65 = Equal?(x=w61, y=w52) -> (x = y?=w53:bool)
        n66 = case shown="False" w53 {
          tunnel: w61 -> [w117 w129]
          tunnel: [w118 w134] -> w59
          tunnel: w30 -> [w116 w125]
          tunnel: [w116 w123] -> w36
          frame False {
            w120 = 0  # Not Found
            n67 = Equal?(x=w117, y=w120) -> (x = y?=w119:bool)
            n68 = case shown="True" w119 {
              tunnel: w117 -> [w121 _]
              tunnel: [w121 w122] -> w118
              frame False {
              }
              frame True {
                w122 = 11  # CheckDAQ
                # "USUAL SCENARIO"
              }
            }
          }
          frame True {
            # "Before allowing data record to be saved,\nprompt user to validate."
            n69 = call "Get Last Record (SubVI).vi"("error in"=w125) -> ("error out"=w124:errorcluster, "experiment record"=w126:i32, "shot record"=w127:i32)  [unwired: 2 out]
            n70 = local write "LastShot"(w127) -> ()
            n71 = local write "LastSample"(w126) -> ()
            n72 = To Double Precision Float(number=w126) -> (double precision float=w128:dbl)
            n73 = Two Button Dialog(message="Are ALL Data Valid?", 1:"NO" ("F button name (\"Cancel\")"), 2:"YES" ("T button name (\"OK\")")) -> (T button?=w133:bool)
            n74 = property on="Record #" class="DigNum (strict)"(error in=w124, "Maximum"=w128) -> (error out=w123:errorcluster)  [unwired: 1 in, 1 out]
            n75 = case shown="False" w133 {
              tunnel: [0 ("index of element") w136] -> w134
              tunnel: w129 -> [_ w136]
              frame False {
                # "POLL"
              }
              frame True {
              }
            }
          }
        }
        n76 = local read "SHOTS"() -> (w27:T7[])
        n77 = To Variant(anything=w59) -> (Variant=w58:variant)
        n78 = for {
          tunnel: w28 -> [w65] mode=indexing
          tunnel: w27 -> [w66] mode=indexing
          tunnel: [w62] -> w26 mode=indexing
          n79 = Not Equal?(x=w66, y=w65) -> (x != y?=w64:T21)
          n80 = Cluster To Array(cluster=w64) -> (array=w63:bool[])
          n81 = Or Array Elements(Boolean array=w63) -> (logical OR=w62:bool)
        }
        n82 = Variant To Data(type=w29, Variant=w58) -> (data=w25:T13)  [unwired: 1 in, 1 out]
        n83 = Or Array Elements(Boolean array=w26) -> (logical OR=w22:bool)
        n84 = Select(t=Collector_State."PROCESS SHOTS" ("progStateType"), s=w22, f=w25) -> (s? t:f=w24:u16)
        "STOP (Shots MC LB)" <- TRUE ("STOP (Shots MC LB)")
      }
      frame 1 {
        # "This section reads the ini file"
        n85 = case shown="100" w145 {
          tunnel: [w151 w170] -> w146
          tunnel: [w149 w170] -> w141
          tunnel: w138 -> [w148 w162]
          tunnel: [w147 w162] -> w137
          frame 0, Default {
            n86 = local read "RESET All"() -> (w150:bool)
            n87 = case shown="True" w150 {
              tunnel: [TRUE w158] -> w151
              tunnel: [FALSE w158] -> w149
              tunnel: w148 -> [w152 w155]
              tunnel: [w152 w155] -> w147
              frame False {
                # "Refresh"
              }
              frame True {
                n88 = Two Button Dialog(message="Resetting will remove all unsaved data.\n\nDo you really  want to reset? ", 1:"NO" ("F button name (\"Cancel\")"), 2:"YES" ("T button name (\"OK\")")) -> (T button?=w158:bool)
              }
            }
          }
          frame 100 {
            w170 = TRUE  # Reset ALL
            n89 = property on="Loading" class="Ring (strict)"("Visible"=FALSE) -> ()  [unwired: 2 in, 2 out]
            n90 = control-ref of="Mfr_0"() -> (w160:refnum<vi>)
            n91 = control-ref of="Mfr_1"() -> (w169:refnum<vi>)
            n92 = control-ref of="Mfr_2"() -> (w168:refnum<vi>)
            n93 = control-ref of="Mfr_3"() -> (w167:refnum<vi>)
            n94 = control-ref of="Mfr_4"() -> (w166:refnum<vi>)
            n95 = control-ref of="Mfr_5"() -> (w165:refnum<vi>)
            n96 = control-ref of="Mfr_6"() -> (w164:refnum<vi>)
            n97 = Build Array(w160, w169, w168, w167, w166, w165, w164) -> (w163:refnum<vi>[])
            n98 = global write "BIMS_Collector Globals.vi" "Mfrs"(w163) -> ()
          }
        }
        n99 = case shown="True" w146 {
          tunnel: [Collector_State."POLL" ("progState") w208] -> w144
          tunnel: w143 -> [w173 _]
          tunnel: [w173 "SHOTS"] -> w142
          tunnel: w141 -> [_ w209]
          tunnel: [w171 w188] -> w139
          tunnel: w137 -> [w171 w207]
          frame False {
            n100 = local write "RESET All"(FALSE ("RESET")) -> ()
          }
          frame True {
            n101 = case shown="True" w209 {
              selector: w209 -> [_ w240]
              tunnel: [w223 w240] -> w189
              tunnel: [w222 w255] -> w190
              tunnel: w207 -> [w222 w242]
              tunnel: [w221 w239] -> w186
              frame False {
                w223 = FALSE  # Reset All
                # "Refresh"
                n102 = local read "configPath"() -> (w221:path)
              }
              frame True {
                # "This section resets\nentire program"
                # "Reset ALL"
                n103 = control-ref of="This VI"() -> (w232:refnum<vi>)
                n104 = invoke on="Invoke Node" class="VI" method="Default Vals.Reinit All"(reference=w232, error in=w242) -> (reference out=w231:refnum<vi>, error out=w230:errorcluster)  [unwired: 1 in, 1 out]
                n105 = property class="VI"(reference=w231, error in=w230, "Front Panel.ShowMenuBar"=FALSE ("Front Panel Window:Show Menu Bar")) -> (reference out=w228:refnum<vi>, error out=w226:errorcluster)
                n106 = property on="mainTabCntrl" class="TabCtl (strict)"() -> (error out=w234:errorcluster, "Pages"=w236:refnum<vi>[])  [unwired: 2 in, 1 out]
                n107 = control-ref of="ScreenSetAvgg"() -> (w250:refnum<vi>)
                n108 = control-ref of="InterlockExists"() -> (w251:refnum<vi>)
                n109 = control-ref of="useBallisitican"() -> (w252:refnum<vi>)
                n110 = control-ref of="useRecorder"() -> (w253:refnum<vi>)
                n111 = control-ref of="useShooter"() -> (w254:refnum<vi>)
                n112 = control-ref of="useBMC"() -> (w225:refnum<vi>)
                n113 = Close Reference(reference=w228, error in (no error)=w226) -> (error out=w227:errorcluster)
                n114 = Index Array(array=w236, index=1) -> (element=w238:refnum<vi>)
                n115 = call "RegReadParams.vi"("ScreenSetAveraging_Ref"=w250, "useBMC_Ref"=w225, "InterlockExist_Ref"=w251, "errorIN"=w227, "useShooter_Ref"=w254, "useRecorder_Ref"=w253, "useBallistician_Ref"=w252) -> ("error out"=w249:errorcluster)  [unwired: 4 out]
                n116 = control-ref of="Server"() -> (w241:refnum<vi>)
                n117 = control-ref of="ConfigName"() -> (w245:refnum<vi>)
                n118 = control-ref of="Site"() -> (w243:refnum<vi>)
                n119 = control-ref of="Folder"() -> (w224:refnum<vi>)
                n120 = property on="Property Node" class="Page"(reference=w238, error in=w234, "PageEnb"=T16."Page Disabled & Grayed" ("Page Enabled State")) -> (error out=w233:errorcluster)  [unwired: 1 out]
                n121 = Build Array(w245, w243, w241, w224) -> (w246:refnum<vi>[])
                n122 = call "InitStringValuesFromRegistry(SubVI).vi"("error in"=w249, "String References"=w246, "subkey"="SOFTWARE\\DuPont\\BIMS-08\\Collector", "root key (HKEY_LOCAL_MACHINE)"=Registry_RtKey."HKEY_LOCAL_MACHINE") -> ("error out"=w248:errorcluster)  [unwired: 3 out]
                n123 = property on="minV50" class="DigNum (strict)"(error in=w233, "Visible"=w240) -> ()  [unwired: 1 in, 2 out]
                n124 = Current VI's Path() -> (path=w258:path)
                n125 = call "Initialize (SubVI).vi"("path"=w258, "error IN"=w248) -> ("pathConfigOUT"=w239:path, "lengthUnits"=→"lengthUnits":string, "massUnits"=→"massUnits":string, "error out"=w255:errorcluster)  [unwired: 1 out]
                "configPath" <- w239
              }
            }
            n126 = control-ref of="Threat"() -> (w193:refnum<vi>)
            n127 = control-ref of="SampleTypes"() -> (w195:refnum<vi>)
            n128 = control-ref of="SampleDescrip"() -> (w202:refnum<vi>)
            n129 = call "Get Threats (SubVI).vi"("pathConfigIN"=w186, "refThreat"=w193, "error in"=w190) -> ("pathConfigOUT"=w197:path, "factorOut"=→"factor array":sgl[], "error out"=w200:errorcluster)  [unwired: 4 out]
            n130 = Bundle("SampleTypes"=w195, "SampleDescrip"=w202) -> (w201:T22)  [unwired: 1 out]
            n131 = call "Fill Lists from INI (SubVI).vi"("clusterListboxes"=w201, "error in"=w200, "pathConfigIN"=w197) -> ("error out"=w199:errorcluster, "pathConfigOUT"=w198:path)  [unwired: 4 out]
            n132 = call "Read Parameters.vi"("error in (no error)"=w199, "appended path"=w198) -> ("error out"=w192:errorcluster, "rangeParams"=w194:T23)  [unwired: 4 out]
            n133 = Unbundle(w194) -> ("max dev"=w175:sgl, "residual separation"=→"Residual/Separation":sgl, "Set#1 Separation"=→"Set#1 Separation":sgl, "Set#2 Separation"=→"Set#2 Separation":sgl, "impact target dist"=w179:sgl, "resid target dist"=w180:sgl, "barrel screen dist"=→"Barrel to Screen":sgl, "midpt_to_target_dist"=→"mid_to_targ_dist":sgl)
            n134 = property on="Ballisticians" class="Ring (strict)"("Visible"="useBallisitican") -> ()  [unwired: 2 in, 2 out]
            n135 = property on="Shooters" class="Ring (strict)"("Visible"="useShooter") -> ()  [unwired: 2 in, 2 out]
            n136 = property on="Recorders" class="Ring (strict)"("Visible"="useRecorder") -> ()  [unwired: 2 in, 2 out]
            n137 = property on="RefreshMetadata" class="Bool (strict)"(error in=w192, "Val(Sgnl)"=TRUE) -> (error out=w187:errorcluster)  [unwired: 1 in, 1 out]
            n138 = local write "Residual/Target Dist"(w180) -> ()
            n139 = local write "maxDev"(w175) -> ()
            n140 = local write "Set#1_to_Target"(w179) -> ()
            n141 = disable-structure shown="Disabled" {
              disable-tunnel: w187 -> [w212 w214]
              disable-tunnel: [w211 w214] -> w183
              frame Disabled {
                n142 = property on="rangeSetup" class="Ring (strict)"(error in=w212, "Val(Sgnl)"=u16 1 ("Value (Signaling)")) -> (error out=w211:errorcluster)  [unwired: 1 in, 1 out]
              }
              frame Enabled {
              }
            }
            n143 = case shown="True" w189 {
              tunnel: [Collector_State."POLL" ("progState") w284] -> w208
              tunnel: [w259 w269] -> w206
              tunnel: w183 -> [w259 w278]
              tunnel: w186 -> [_ w268]
              tunnel: "useBMC" -> [_ w267]
              frame False {
                # "Refresh"
              }
              frame True {
                w261 = T15."Disabled and Grayed Out" ("Disabled")
                # "Reset ALL"
                n144 = global read "BIMS_Collector Globals.vi" "SampleStyles"() -> (w271:refnum<vi>[])
                n145 = case shown="True" w267 {
                  tunnel: w268 -> [_ w286]
                  frame False {
                  }
                  frame True {
                    n146 = Path To String(path=w286) -> (string=w287:string)
                    n147 = call "Ballistics Message Center.vi"("INI File Name"=w287) -> ()
                  }
                }
                n148 = call "Get Last Record (SubVI).vi"("error in"=w278) -> ("error out"=w270:errorcluster, "experiment record"=w276:i32, "shot record"=→"LastShot":i32)  [unwired: 2 out]
                "LastSample" <- w276
                n149 = local read "MeasSrc"() -> (w285:T6)
                n150 = local read "InterlockExists"() -> (w283:bool)
                n151 = control-ref of="ThreatDetails"() -> (w266:refnum<vi>)
                n152 = control-ref of="SampleStyle_0"() -> (w273:refnum<vi>)
                n153 = control-ref of="ThreatGroups"() -> (w272:refnum<vi>)
                n154 = local read "SafetyInterlock"() -> (w281:cluster{"ARMED":bool})
                n155 = Bundle By Name(cluster=w281, "ARMED"=FALSE) -> (w280:cluster{"ARMED":bool})
                n156 = To Double Precision Float(number=w276) -> (double precision float=w275:dbl)
                n157 = property on="Record #" class="DigNum (strict)"(error in=w270, "Maximum"=w275) -> (error out=w269:errorcluster)  [unwired: 1 in, 1 out]
                n158 = case shown="\"Screens\"" w285 {
                  tunnel: [Collector_State."POLL" ("progState") Collector_State."POLL" ("progState") Collector_State."READY CLOCK" ("progState")] -> w284
                  frame "Simulated", Default {
                  }
                  frame "Radar" {
                  }
                  frame "Screens" {
                    # "check for PCI 6602"
                  }
                }
                n159 = Build Array (concatenate)(w266, w273, w272, w271) -> (w274:refnum<vi>[])
                n160 = local write "SafetyInterlock"(w280) -> ()
                n161 = Select(t=T15."Enabled" ("Disabled"), s=w283, f=T15."Disabled and Grayed Out" ("Disabled")) -> (s? t:f=w282:T15)
                n162 = for {
                  tunnel: w274 -> [w288] mode=indexing
                  n163 = property on="Property Node" class="Ring (strict)"(reference=w288, "Strings []"=string[] []) -> ()  [unwired: 1 in, 2 out]
                }
                n164 = property on="addShot" class="Bool"("Disabled"=T15."Enabled") -> ()  [unwired: 2 in, 2 out]
                n165 = property on="undoLastShot" class="Bool"("Disabled"=w261) -> ()  [unwired: 2 in, 2 out]
                n166 = property on="saveShots" class="Bool"("Disabled"=w261) -> ()  [unwired: 2 in, 2 out]
                n167 = property on="clearShots" class="Bool"("Disabled"=w261) -> ()  [unwired: 2 in, 2 out]
                n168 = property on="ARM" class="Bool"("Disabled"=w282) -> ()  [unwired: 2 in, 2 out]
                n169 = property on="SafetyInterlock" class="Clust (strict)"("Disabled"=w282) -> ()  [unwired: 2 in, 2 out]
                n170 = property on="saveReq" class="Str"("Visible"=TRUE) -> ()  [unwired: 2 in, 2 out]
              }
            }
            n171 = call <vilib>:"General Error Handler.vi"("error in (no error)"=w206) -> ("error out"=w188:errorcluster)  [unwired: 2 in, 12 out]
            n172 = flat-sequence {
              tunnel: w188 -> [w215]
              frame #0 {
                n173 = local read "ConfigName"() -> (w216:string)
                n174 = case shown="No Error" w215 {
                  tunnel: [w219 "NOT READY!" ("ConfigName")] -> w217
                  tunnel: w216 -> [w219 _]
                  frame No Error {
                    n175 = Wait (ms)(milliseconds to wait=u32 1000) -> ()  [unwired: 1 out]
                  }
                  frame Error {
                  }
                }
                "ConfigName" <- w217
              }
            }
            "saveReq" <- "Number of layers in sample ply specification and number of shots in shots table must be greater than 0 to enable saving." ("saveReq")
          }
        }
      }
      frame 2 {
        # "The custom Excel template file is \nexpected in the C:\\Ballistics folder."
        n176 = case shown="True" "lookupRec" {
          selector: "lookupRec" -> [_ w820]
          tunnel: [w343 w810] -> w324
          tunnel: [w342 w796] -> w323
          tunnel: [w341 w813] -> w322
          tunnel: [w340 w753] -> w321
          tunnel: [w339 w811] -> w320
          tunnel: [w338 w773] -> w319
          tunnel: [w337 w760] -> w306
          tunnel: [w336 w762] -> w305
          tunnel: [w335 w763] -> w304
          tunnel: [w334 "Record #"] -> w303
          tunnel: [w333 w812] -> w302
          tunnel: [w332 w762] -> w295
          tunnel: w300 -> [w331 _]
          tunnel: [w330 w785] -> w298
          tunnel: w297 -> [w330 w786]
          tunnel: [w329 w758] -> w293
          frame False {
            n177 = stacked-sequence {
              tunnel: [_ _ _ _ _ w673] -> w338
              tunnel: [_ w412 _ _ _ _] -> w342
              tunnel: [_ _ _ _ w517 _] -> w339
              tunnel: [_ _ _ w463 _ _] -> w340
              tunnel: [_ _ w434 _ _ _] -> w341
              tunnel: [w355 _ _ _ _ _] -> w343
              tunnel: [_ _ _ _ _ w679] -> w337
              tunnel: [_ _ _ _ _ w675] -> w336
              tunnel: [_ _ _ _ _ w674] -> w335
              tunnel: [_ _ _ _ _ w678] -> w334
              tunnel: [_ _ _ _ _ w677] -> w333
              tunnel: [_ _ _ _ _ w676] -> w332
              tunnel: w331 -> [_ _ w433 _ w516 _]
              frame #0 {
                # "Need to remove first element\nsince it's associated with the \nhistory page."
                # "FABRIC"
                n178 = local read "fab1_totalWt"() -> (w358:sgl)
                n179 = local read "fab3_totalWt"() -> (w360:sgl)
                n180 = local read "fab5_totalWt"() -> (w362:sgl)
                n181 = global read "BIMS_Collector Globals.vi" "SampleStyles"() -> (w346:refnum<vi>[])
                n182 = global read "BIMS_Collector Globals.vi" "Mfrs"() -> (w351:refnum<vi>[])
                n183 = local read "fab2_totalWt"() -> (w359:sgl)
                n184 = local read "fab4_totalWt"() -> (w361:sgl)
                n185 = local read "fab6_totalWt"() -> (w363:sgl)
                n186 = global read "BIMS_Collector Globals.vi" "LayerStitchTypeRefs"() -> (w353:refnum<vi>[])
                n187 = global read "BIMS_Collector Globals.vi" "SampleAttribs"() -> (w344:T24)
                n188 = global read "BIMS_Collector Globals.vi" "LayerSpecs"() -> (w354:T25)
                n189 = Delete From Array(array=w346, length=1, index=0) -> (array with subset deleted=w345:refnum<vi>[])  [unwired: 1 out]
                n190 = Delete From Array(array=w351, length=1, index=0) -> (array with subset deleted=w352:refnum<vi>[])  [unwired: 1 out]
                n191 = Build Array(w358, w359, w360, w361, w362, w363) -> (w357:sgl[])
                n192 = for {
                  tunnel: w357 -> [w367] mode=indexing
                  tunnel: [w375] -> w356 mode=indexing
                  tunnel: w344 -> [w374] mode=indexing
                  tunnel: w354 -> [w373] mode=indexing
                  tunnel: w352 -> [w372] mode=indexing
                  tunnel: w345 -> [w371] mode=indexing
                  tunnel: w353 -> [w370] mode=indexing
                  n193 = call "Dropdown Selection (SubVI).vi"("reference"=w372) -> ("element"=w365:string)
                  n194 = call "Dropdown Selection (SubVI).vi"("reference"=w371) -> ("element"=w369:string)
                  n195 = Equal?(x="", y=w365) -> (x = y?=w364:bool)
                  n196 = call "Dropdown Selection (SubVI).vi"("reference"=w370) -> ("element"=w368:string)
                  n197 = case shown="False" w364 {
                    tunnel: [w394 w396] -> w375
                    tunnel: w374 -> [w393 _]
                    tunnel: w373 -> [w392 _]
                    tunnel: w369 -> [w386 _]
                    tunnel: w368 -> [w381 _]
                    tunnel: w367 -> [w379 _]
                    tunnel: w365 -> [w378 _]
                    frame False {
                      n198 = Unbundle By Name(w392) -> ("numOfPlies"=w380:i32, "LotNum"=w389:string, "RollNum"=w390:string)
                      n199 = Unbundle By Name(w393) -> ("internal_ID"=w384:string, "fiber"=w385:string, "denier"=w388:string, "pick"=w387:string, "weave"=w382:string, "finish"=w383:string, "ozPerYd2"=w391:string)
                      n200 = Format Into String(w380) -> (resulting string=w377:string)  [unwired: 3 in, 1 out]
                      n201 = Format Into String(w379) -> (resulting string=w376:string)  [unwired: 3 in, 1 out]
                      n202 = Build Array(w377, w378, w386, w384, w385, w388, w387, w382, w383, w389, w390, w391, w376, w381) -> (w394:string[])
                    }
                    frame True {
                      n203 = Initialize Array("", 14 ("dimension size")) -> (w396:string[])
                    }
                  }
                }
                n204 = Transpose 2D Array(2D array=w356) -> (transposed array=w355:string[][])
              }
              frame #1 {
                w398 = "%.1f" ("format string")
                # "muzzel / midpoint"
                # "muzzle / scr#1"
                # "muzzle / target"
                # "scr#2 / target"
                # "RANGE"
                n205 = local read "Set#1 Separation"() -> (w405:sgl)
                n206 = local read "mid_to_targ_dist"() -> (w402:sgl)
                n207 = local read "Barrel to Screen"() -> (w399:sgl)
                n208 = local read "clayAverage"() -> (w420:sgl)
                n209 = Divide(x=w405, y=sgl 2.0) -> (x/y=w400:sgl)
                n210 = local read "RoomHum"() -> (w415:sgl)
                n211 = local read "clayTemp"() -> (w418:sgl)
                n212 = local read "clayCalib"() -> (w421:string)
                n213 = local read "RoomT"() -> (w416:sgl)
                n214 = Add(x=w399, y=w402) -> (x+y=w406:sgl)
                n215 = Subtract(x=w399, y=w400) -> (x-y=w401:sgl)
                n216 = Subtract(x=w402, y=w400) -> (x-y=w403:sgl)
                n217 = Format Into String(w406) -> (resulting string=w407:string)  [unwired: 3 in, 1 out]
                n218 = Format Into String(w401) -> (resulting string=w408:string)  [unwired: 3 in, 1 out]
                n219 = Format Into String(w405) -> (resulting string=w409:string)  [unwired: 3 in, 1 out]
                n220 = Format Into String(w403) -> (resulting string=w410:string)  [unwired: 3 in, 1 out]
                n221 = Format Into String(w402) -> (resulting string=w411:string)  [unwired: 3 in, 1 out]
                n222 = Format Into String(w415) -> (resulting string=w413:string)  [unwired: 3 in, 1 out]
                n223 = Format Into String(format string=w398, w416) -> (resulting string=w414:string)  [unwired: 2 in, 1 out]
                n224 = Format Into String(format string=w398, w418) -> (resulting string=w417:string)  [unwired: 2 in, 1 out]
                n225 = Format Into String(format string=w398, w420) -> (resulting string=w419:string)  [unwired: 2 in, 1 out]
                n226 = Bundle(w407, w408, w409, w410, w411, w413, w414, w417, "clayCalib"=w421, w419) -> (w422:T26)  [unwired: 1 out]
                n227 = Cluster To Array(cluster=w422) -> (array=w412:string[])
              }
              frame #2 {
                # "RESULTS"
                n228 = control-ref of="Methods"() -> (w423:refnum<vi>)
                n229 = call "Dropdown Selection (SubVI).vi"("reference"=w423) -> ("element"=w424:string)
                n230 = for {
                  tunnel: w433 -> [w461] mode=indexing
                  tunnel: [w460] -> w432 mode=indexing
                  tunnel: [w459] -> w431
                  i -> [w459]
                  n231 = Unbundle By Name(w461) -> ("BackFace\nDepth"=w460:sgl)
                }
                n232 = Increment(x=w431) -> (x+1=w429:i32)
                n233 = Add Array Elements(numeric array=w432) -> (sum=w430:sgl)
                n234 = To Single Precision Float(number=w429) -> (single precision float=w428:sgl)
                n235 = Divide(x=w430, y=w428) -> (x/y=w427:sgl)
                n236 = Format Into String(format string="%1.1f", w427) -> (resulting string=w426:string)  [unwired: 2 in, 1 out]
                n237 = case shown="\"V50\"" w424 {
                  tunnel: [w449 w458] -> w436
                  tunnel: w426 -> [w437 w457]
                  frame "V50" {
                    w443 = "%1d" ("format string")
                    n238 = local read "Z.M.R."() -> (w441:sgl)
                    n239 = Less Than 0?(x=w441) -> (x < 0?=w442:bool)
                    n240 = local read "rangeOfResults"() -> (w445:i32)
                    n241 = local read "computed_V50"() -> (w448:sgl)
                    n242 = local read "lowComplete"() -> (w446:i32)
                    n243 = local read "highPartial"() -> (w447:i32)
                    n244 = case shown="True" w442 {
                      tunnel: w441 -> [w454 _]
                      tunnel: [w454 sgl 0.0 ("Z.M.R.")] -> w440
                      frame False {
                      }
                      frame True {
                      }
                    }
                    n245 = Format Into String(format string="%1.1f", w448) -> (resulting string=w452:string)  [unwired: 2 in, 1 out]
                    n246 = Format Into String(format string=w443, w447) -> (resulting string=w451:string)  [unwired: 2 in, 1 out]
                    n247 = Format Into String(format string=w443, w446) -> (resulting string=w450:string)  [unwired: 2 in, 1 out]
                    n248 = Format Into String(format string=w443, w445) -> (resulting string=w453:string)  [unwired: 2 in, 1 out]
                    n249 = Format Into String(format string="%1.1f", w440) -> (resulting string=w439:string)  [unwired: 2 in, 1 out]
                    n250 = Bundle(w452, w451, w450, w453, w439, w437, w437) -> (w449:T27)  [unwired: 1 out]
                  }
                  frame Default {
                    w456 = "" ("Empty String Constant")
                    n251 = Bundle(w456, w456, w456, w456, w456, w457, w457) -> (w458:T27)  [unwired: 1 out]
                  }
                }
                n252 = Cluster To Array(cluster=w436) -> (array=w435:string[])
                n253 = Build Array(w435) -> (w434:string[][])
              }
              frame #3 {
                # "SAMPLE"
                n254 = local read "Site"() -> (w462:string)
                n255 = case shown="\"SPR1\"" w462 {
                  tunnel: [w465 w489 w502] -> w463
                  frame "ICE1", Default {
                    # "PB Req"
                    n256 = control-ref of="Methods"() -> (w466:refnum<vi>)
                    n257 = call "Dropdown Selection (SubVI).vi"("reference"=w466) -> ("element"=w468:string)
                    n258 = Equal?(x=w468, y="V50") -> (x = y?=w467:bool)
                    n259 = local read "totalSampleWt"() -> (w478:sgl)
                    n260 = case shown="True" w467 {
                      tunnel: ["n/a" w488] -> w472
                      frame False {
                      }
                      frame True {
                        n261 = local read "minV50"() -> (w487:i32)
                        n262 = Format Into String(w487) -> (resulting string=w488:string)  [unwired: 3 in, 1 out]
                      }
                    }
                    n263 = control-ref of="SampleDimensions"() -> (w484:refnum<vi>)
                    n264 = control-ref of="SampleCoverings"() -> (w485:refnum<vi>)
                    n265 = control-ref of="Models"() -> (w471:refnum<vi>)
                    n266 = local read "serialNum"() -> (w480:string)
                    n267 = local read "SampleID"() -> (w482:string)
                    n268 = local read "Thickness"() -> (w475:dbl)
                    n269 = local read "totalBAW"() -> (w474:sgl)
                    n270 = call "Dropdown Selection (SubVI).vi"("reference"=w484) -> ("element"=w481:string)
                    n271 = call "Dropdown Selection (SubVI).vi"("reference"=w471) -> ("element"=w470:string)
                    n272 = call "Dropdown Selection (SubVI).vi"("reference"=w485) -> ("element"=w479:string)
                    n273 = Format Into String(w478) -> (resulting string=w477:string)  [unwired: 3 in, 1 out]
                    n274 = Format Into String(w475) -> (resulting string=w476:string)  [unwired: 3 in, 1 out]
                    n275 = Format Into String(w474) -> (resulting string=w473:string)  [unwired: 3 in, 1 out]
                    n276 = Bundle("SampleID"=w482, "element"=w481, "Type of work"="Type of work", "serialNum"=w480, "element"=w470, w477, w476, w473, "element"=w479, w472) -> (w483:T28)  [unwired: 1 out]
                    n277 = Cluster To Array(cluster=w483) -> (array=w465:string[])
                  }
                  frame "SPR0" {
                    n278 = local read "totalSampleWt"() -> (w495:sgl)
                    n279 = control-ref of="SampleDimensions"() -> (w500:refnum<vi>)
                    n280 = control-ref of="SampleCoverings"() -> (w501:refnum<vi>)
                    n281 = local read "SampleID"() -> (w498:string)
                    n282 = local read "Thickness"() -> (w492:dbl)
                    n283 = local read "totalBAW"() -> (w491:sgl)
                    n284 = call "Dropdown Selection (SubVI).vi"("reference"=w500) -> ("element"=w497:string)
                    n285 = call "Dropdown Selection (SubVI).vi"("reference"=w501) -> ("element"=w496:string)
                    n286 = Format Into String(w495) -> (resulting string=w494:string)  [unwired: 3 in, 1 out]
                    n287 = Format Into String(w492) -> (resulting string=w493:string)  [unwired: 3 in, 1 out]
                    n288 = Format Into String(w491) -> (resulting string=w490:string)  [unwired: 3 in, 1 out]
                    n289 = Bundle("SampleID"=w498, "element"=w497, w494, w493, w490, "element"=w496) -> (w499:T29)  [unwired: 1 out]
                    n290 = Cluster To Array(cluster=w499) -> (array=w489:string[])
                  }
                  frame "SPR1" {
                    n291 = local read "totalSampleWt"() -> (w508:sgl)
                    n292 = control-ref of="SampleDimensions"() -> (w513:refnum<vi>)
                    n293 = control-ref of="SampleCoverings"() -> (w514:refnum<vi>)
                    n294 = local read "SampleID"() -> (w511:string)
                    n295 = local read "Thickness"() -> (w505:dbl)
                    n296 = local read "totalBAW"() -> (w504:sgl)
                    n297 = call "Dropdown Selection (SubVI).vi"("reference"=w513) -> ("element"=w510:string)
                    n298 = call "Dropdown Selection (SubVI).vi"("reference"=w514) -> ("element"=w509:string)
                    n299 = Format Into String(w508) -> (resulting string=w507:string)  [unwired: 3 in, 1 out]
                    n300 = Format Into String(w505) -> (resulting string=w506:string)  [unwired: 3 in, 1 out]
                    n301 = Format Into String(w504) -> (resulting string=w503:string)  [unwired: 3 in, 1 out]
                    n302 = Bundle("SampleID"=w511, "element"=w510, w507, w506, w503, "element"=w509) -> (w512:T29)  [unwired: 1 out]
                    n303 = Cluster To Array(cluster=w512) -> (array=w502:string[])
                  }
                }
              }
              frame #4 {
                n304 = local read "Site"() -> (w515:string)
                n305 = case shown="\"SPR1\"" w515 {
                  tunnel: [w527 w577 w629] -> w517
                  tunnel: w516 -> [w520 w570 w622]
                  frame "ICE1", Default {
                    # "SHOT TABLE"
                    n306 = control-ref of="Methods"() -> (w519:refnum<vi>)
                    n307 = call "Dropdown Selection (SubVI).vi"("reference"=w519) -> ("element"=w518:string)
                    n308 = for {
                      tunnel: w520 -> [w559] mode=indexing
                      shift-right: [w536] -> _
                      shift-left: T18 [] -> [w538]
                      tunnel: [w536] -> w523
                      tunnel: w518 -> [w532]
                      n309 = Unbundle By Name(w559) -> ("shot order"=w558:i32, "Powder Loading"=w557:sgl, "Uncorrected Impact"=w556:sgl, "UncorrectedRed_PB"=w555:sgl, "UncorrectedAvgVel_PB"=w554:sgl, "velLoss_PB"=w553:sgl, "strikeVel_PB"=w552:sgl, "SHOT STATUS"=w541:u16, "usedv50"=w551:bool, "Shot Angle"=w533:u16, "BackFace\nDepth"=w534:sgl)
                      n310 = case shown="\"V50\"" w532 {
                        tunnel: w551 -> [w561 _]
                        tunnel: [w560 w565] -> w550
                        tunnel: w533 -> [_ w564]
                        frame "V50" {
                          n311 = case shown="True" w561 {
                            tunnel: ["" ("Empty String Constant") "*"] -> w560
                            frame False {
                            }
                            frame True {
                            }
                          }
                        }
                        frame Default {
                          n312 = Format Into String(w564) -> (resulting string=w565:string)  [unwired: 3 in, 1 out]
                        }
                      }
                      n313 = case shown="1" w541 {
                        tunnel: ["P" "C"] -> w540
                        frame 0, Default {
                        }
                        frame 1 {
                        }
                      }
                      n314 = Format Into String(format string="%2d", w558) -> (resulting string=w543:string)  [unwired: 2 in, 1 out]
                      n315 = Format Into String(w557) -> (resulting string=w544:string)  [unwired: 3 in, 1 out]
                      n316 = Format Into String(w556) -> (resulting string=w545:string)  [unwired: 3 in, 1 out]
                      n317 = Format Into String(w555) -> (resulting string=w546:string)  [unwired: 3 in, 1 out]
                      n318 = Format Into String(w554) -> (resulting string=w547:string)  [unwired: 3 in, 1 out]
                      n319 = Format Into String(w553) -> (resulting string=w548:string)  [unwired: 3 in, 1 out]
                      n320 = Format Into String(w552) -> (resulting string=w549:string)  [unwired: 3 in, 1 out]
                      n321 = Format Into String(w534) -> (resulting string=w542:string)  [unwired: 3 in, 1 out]
                      n322 = Build Array(w543, w544, w545, w546, w547, w548, w549, w540, w550, w542) -> (w537:string[])
                      n323 = Array To Cluster(array=w537) -> (cluster=w539:T30)
                      n324 = Build Array (concatenate)(w538, w539) -> (w536:T18)
                    }
                    n325 = Array Size(array=w523) -> (size(s)=w525:i32)
                    n326 = Equal To 0?(x=w525) -> (x = 0?=w521:bool)
                    n327 = case shown="True" w521 {
                      tunnel: [w528 T18 [{"[0]"="", "[1]"="", "[2]"="", "[3]"="", "[4]"="", "[5]"="", "[6]"="", "[7]"="", "[8]"="", "[9]"=""}]] -> w522
                      tunnel: w523 -> [w528 _]
                      frame False {
                      }
                      frame True {
                      }
                    }
                    n328 = Sort 1D Array(array=w522) -> (sorted array=w524:T18)
                    n329 = for {
                      tunnel: w524 -> [w531] mode=indexing
                      tunnel: [w530] -> w527 mode=indexing
                      n330 = Cluster To Array(cluster=w531) -> (array=w530:string[])
                    }
                  }
                  frame "SPR0" {
                    # "SHOT TABLE"
                    n331 = control-ref of="Methods"() -> (w569:refnum<vi>)
                    n332 = call "Dropdown Selection (SubVI).vi"("reference"=w569) -> ("element"=w568:string)
                    n333 = for {
                      tunnel: w570 -> [w607] mode=indexing
                      shift-right: [w588] -> _
                      shift-left: T19 [] -> [w590]
                      tunnel: [w588] -> w573
                      tunnel: w568 -> [w584]
                      n334 = Unbundle By Name(w607) -> ("shot order"=w606:i32, "Powder Loading"=w605:sgl, "Uncorrected Impact"=w604:sgl, "UncorrectedRed_PB"=w603:sgl, "strikeVel_PB"=w602:sgl, "SHOT STATUS"=w593:u16, "usedv50"=w601:bool, "Shot Angle"=w585:u16, "BackFace\nDepth"=w586:sgl, "V50userExcl"=w583:bool, "Shot Description"=w582:string)
                      n335 = case shown="\"V50\"" w584 {
                        tunnel: w601 -> [w610 _]
                        tunnel: [w609 w617] -> w600
                        tunnel: w585 -> [_ w616]
                        tunnel: w583 -> [w608 _]
                        frame "V50" {
                          n336 = case shown="True" w608 {
                            tunnel: w610 -> [w612 _]
                            tunnel: [w611 "!"] -> w609
                            frame False {
                              n337 = case shown="False" w612 {
                                tunnel: ["" ("Empty String Constant") "*"] -> w611
                                frame False {
                                }
                                frame True {
                                }
                              }
                            }
                            frame True {
                            }
                          }
                        }
                        frame Default {
                          n338 = Format Into String(w616) -> (resulting string=w617:string)  [unwired: 3 in, 1 out]
                        }
                      }
                      n339 = case shown="1" w593 {
                        tunnel: ["P" "C"] -> w592
                        frame 0, Default {
                        }
                        frame 1 {
                        }
                      }
                      n340 = Format Into String(format string="%2d", w606) -> (resulting string=w595:string)  [unwired: 2 in, 1 out]
                      n341 = Format Into String(w605) -> (resulting string=w596:string)  [unwired: 3 in, 1 out]
                      n342 = Format Into String(w604) -> (resulting string=w597:string)  [unwired: 3 in, 1 out]
                      n343 = Format Into String(w603) -> (resulting string=w598:string)  [unwired: 3 in, 1 out]
                      n344 = Format Into String(w602) -> (resulting string=w599:string)  [unwired: 3 in, 1 out]
                      n345 = Format Into String(w586) -> (resulting string=w594:string)  [unwired: 3 in, 1 out]
                      n346 = Build Array(w595, w596, w597, w598, w599, w592, w600, w594, w582) -> (w589:string[])
                      n347 = Array To Cluster(array=w589) -> (cluster=w591:T31)
                      n348 = Build Array (concatenate)(w590, w591) -> (w588:T19)
                    }
                    n349 = Array Size(array=w573) -> (size(s)=w575:i32)
                    n350 = Equal To 0?(x=w575) -> (x = 0?=w571:bool)
                    n351 = case shown="True" w571 {
                      tunnel: [w578 T19 [{"[0]"="", "[1]"="", "[2]"="", "[3]"="", "[4]"="", "[5]"="", "[6]"="", "[7]"="", "[8]"=""}]] -> w572
                      tunnel: w573 -> [w578 _]
                      frame False {
                      }
                      frame True {
                      }
                    }
                    n352 = Sort 1D Array(array=w572) -> (sorted array=w574:T19)
                    n353 = for {
                      tunnel: w574 -> [w581] mode=indexing
                      tunnel: [w580] -> w577 mode=indexing
                      n354 = Cluster To Array(cluster=w581) -> (array=w580:string[])
                    }
                  }
                  frame "SPR1" {
                    # "SHOT TABLE"
                    n355 = control-ref of="Methods"() -> (w621:refnum<vi>)
                    n356 = call "Dropdown Selection (SubVI).vi"("reference"=w621) -> ("element"=w620:string)
                    n357 = for {
                      tunnel: w622 -> [w659] mode=indexing
                      shift-right: [w640] -> _
                      shift-left: T19 [] -> [w642]
                      tunnel: [w640] -> w625
                      tunnel: w620 -> [w636]
                      n358 = Unbundle By Name(w659) -> ("shot order"=w658:i32, "Powder Loading"=w657:sgl, "Uncorrected Impact"=w656:sgl, "UncorrectedRed_PB"=w655:sgl, "strikeVel_PB"=w654:sgl, "SHOT STATUS"=w645:u16, "usedv50"=w653:bool, "Shot Angle"=w637:u16, "BackFace\nDepth"=w638:sgl, "V50userExcl"=w635:bool, "Shot Description"=w634:string)
                      n359 = case shown="\"V50\"" w636 {
                        tunnel: w653 -> [w662 _]
                        tunnel: [w661 w669] -> w652
                        tunnel: w637 -> [_ w668]
                        tunnel: w635 -> [w660 _]
                        frame "V50" {
                          n360 = case shown="True" w660 {
                            tunnel: w662 -> [w664 _]
                            tunnel: [w663 "!"] -> w661
                            frame False {
                              n361 = case shown="False" w664 {
                                tunnel: ["" ("Empty String Constant") "*"] -> w663
                                frame False {
                                }
                                frame True {
                                }
                              }
                            }
                            frame True {
                            }
                          }
                        }
                        frame Default {
                          n362 = Format Into String(w668) -> (resulting string=w669:string)  [unwired: 3 in, 1 out]
                        }
                      }
                      n363 = case shown="1" w645 {
                        tunnel: ["P" "C"] -> w644
                        frame 0, Default {
                        }
                        frame 1 {
                        }
                      }
                      n364 = Format Into String(format string="%2d", w658) -> (resulting string=w647:string)  [unwired: 2 in, 1 out]
                      n365 = Format Into String(w657) -> (resulting string=w648:string)  [unwired: 3 in, 1 out]
                      n366 = Format Into String(w656) -> (resulting string=w649:string)  [unwired: 3 in, 1 out]
                      n367 = Format Into String(w655) -> (resulting string=w650:string)  [unwired: 3 in, 1 out]
                      n368 = Format Into String(w654) -> (resulting string=w651:string)  [unwired: 3 in, 1 out]
                      n369 = Format Into String(w638) -> (resulting string=w646:string)  [unwired: 3 in, 1 out]
                      n370 = Build Array(w647, w648, w649, w650, w651, w644, w652, w646, w634) -> (w641:string[])
                      n371 = Array To Cluster(array=w641) -> (cluster=w643:T31)
                      n372 = Build Array (concatenate)(w642, w643) -> (w640:T19)
                    }
                    n373 = Array Size(array=w625) -> (size(s)=w627:i32)
                    n374 = Equal To 0?(x=w627) -> (x = 0?=w623:bool)
                    n375 = case shown="True" w623 {
                      tunnel: [w630 T19 [{"[0]"="", "[1]"="", "[2]"="", "[3]"="", "[4]"="", "[5]"="", "[6]"="", "[7]"="", "[8]"=""}]] -> w624
                      tunnel: w625 -> [w630 _]
                      frame False {
                      }
                      frame True {
                      }
                    }
                    n376 = Sort 1D Array(array=w624) -> (sorted array=w626:T19)
                    n377 = for {
                      tunnel: w626 -> [w633] mode=indexing
                      tunnel: [w632] -> w629 mode=indexing
                      n378 = Cluster To Array(cluster=w633) -> (array=w632:string[])
                    }
                  }
                }
              }
              frame #5 {
                n379 = local read "Site"() -> (w672:string)
                n380 = case shown="\"ICE1\", Default" w672 {
                  tunnel: [w703 w724 w744] -> w679
                  tunnel: [w702 w723 w743] -> w678
                  tunnel: [w701 w722 w742] -> w677
                  tunnel: [w700 w707 w727] -> w676
                  tunnel: ["" ("projNum") w707 w727] -> w675
                  tunnel: [w698 w721 w741] -> w674
                  tunnel: [w682 w710 w730] -> w673
                  frame "ICE1", Default {
                    # "THREAT"
                    # "Range # (supports a PB reporting requirement)"
                    # "Project Name goes here.\nSupports a PB reporting requirement."
                    # "GENERAL"
                    n381 = local read "threatDetails"() -> (w681:T1)
                    n382 = Unbundle By Name(w681) -> ("barrelLength"=w685:string)
                    n383 = Unbundle By Name(w681) -> ("grainSize"=w680:string)
                    n384 = local read "Shot Angle"() -> (w686:u16)
                    n385 = control-ref of="WeaponTypes"() -> (w695:refnum<vi>)
                    n386 = control-ref of="ThreatGroups"() -> (w694:refnum<vi>)
                    n387 = control-ref of="PowderTypes"() -> (w693:refnum<vi>)
                    n388 = control-ref of="Recorders"() -> (w696:refnum<vi>)
                    n389 = control-ref of="Shooters"() -> (w697:refnum<vi>)
                    n390 = Format Into String(w686) -> (resulting string=w687:string)  [unwired: 3 in, 1 out]
                    n391 = call "Dropdown Selection (SubVI).vi"("reference"=w695) -> ("element"=w691:string)
                    n392 = call "Dropdown Selection (SubVI).vi"("reference"=w694) -> ("element"=w690:string)
                    n393 = call "Dropdown Selection (SubVI).vi"("reference"=w693) -> ("element"=w689:string)
                    n394 = call "Dropdown Selection (SubVI).vi"("reference"=w696) -> ("element"=w688:string)
                    n395 = call "Dropdown Selection (SubVI).vi"("reference"=w697) -> ("element"=w684:string)
                    n396 = local read "Comments"() -> (w701:string)
                    n397 = local read "ProjectID"() -> (w698:string)
                    n398 = local read "LastSample"() -> (w706:i32)
                    n399 = Bundle("element"=w691, "element"=w690, "grainSize"=w680, "element"=w689, "barrelLength"=w685, w687, "element"="1", "element"=w684, "element"=w688) -> (w692:T32)  [unwired: 1 out]
                    n400 = control-ref of="TestStandards"() -> (w705:refnum<vi>)
                    n401 = control-ref of="Methods"() -> (w704:refnum<vi>)
                    n402 = Cluster To Array(cluster=w692) -> (array=w682:string[])
                    n403 = call "Dropdown Selection (SubVI).vi"("reference"=w705) -> ("element"=w700:string)
                    n404 = call "Dropdown Selection (SubVI).vi"("reference"=w704) -> ("element"=w703:string)
                    n405 = Increment(x=w706) -> (x+1=w702:i32)
                  }
                  frame "SPR0" {
                    w707 = "" ("projNum")
                    # "THREAT"
                    # "Project Name goes here.\nSupports a PB reporting requirement."
                    # "GENERAL"
                    n406 = local read "threatDetails"() -> (w709:T1)
                    n407 = Unbundle By Name(w709) -> ("barrelLength"=w712:string)
                    n408 = Unbundle By Name(w709) -> ("grainSize"=w708:string)
                    n409 = local read "Shot Angle"() -> (w713:u16)
                    n410 = control-ref of="ThreatGroups"() -> (w719:refnum<vi>)
                    n411 = control-ref of="PowderTypes"() -> (w718:refnum<vi>)
                    n412 = control-ref of="Ballisticians"() -> (w720:refnum<vi>)
                    n413 = Format Into String(w713) -> (resulting string=w714:string)  [unwired: 3 in, 1 out]
                    n414 = call "Dropdown Selection (SubVI).vi"("reference"=w719) -> ("element"=w716:string)
                    n415 = call "Dropdown Selection (SubVI).vi"("reference"=w718) -> ("element"=w715:string)
                    n416 = call "Dropdown Selection (SubVI).vi"("reference"=w720) -> ("element"=w711:string)
                    n417 = local read "Comments"() -> (w722:string)
                    n418 = local read "ProjectID"() -> (w721:string)
                    n419 = local read "LastSample"() -> (w726:i32)
                    n420 = Bundle("element"=w716, "grainSize"=w708, "element"=w715, "barrelLength"=w712, w714, "element"=w711) -> (w717:T33)  [unwired: 1 out]
                    n421 = control-ref of="Methods"() -> (w725:refnum<vi>)
                    n422 = Cluster To Array(cluster=w717) -> (array=w710:string[])
                    n423 = call "Dropdown Selection (SubVI).vi"("reference"=w725) -> ("element"=w724:string)
                    n424 = Increment(x=w726) -> (x+1=w723:i32)
                  }
                  frame "SPR1" {
                    w727 = "" ("projNum")
                    # "THREAT"
                    # "Project Name goes here.\nSupports a PB reporting requirement."
                    # "GENERAL"
                    n425 = local read "threatDetails"() -> (w729:T1)
                    n426 = Unbundle By Name(w729) -> ("barrelLength"=w732:string)
                    n427 = Unbundle By Name(w729) -> ("grainSize"=w728:string)
                    n428 = local read "Shot Angle"() -> (w733:u16)
                    n429 = control-ref of="Ballisticians"() -> (w740:refnum<vi>)
                    n430 = control-ref of="ThreatGroups"() -> (w739:refnum<vi>)
                    n431 = control-ref of="PowderTypes"() -> (w738:refnum<vi>)
                    n432 = call "Dropdown Selection (SubVI).vi"("reference"=w740) -> ("element"=w731:string)
                    n433 = call "Dropdown Selection (SubVI).vi"("reference"=w739) -> ("element"=w736:string)
                    n434 = call "Dropdown Selection (SubVI).vi"("reference"=w738) -> ("element"=w735:string)
                    n435 = Format Into String(w733) -> (resulting string=w734:string)  [unwired: 3 in, 1 out]
                    n436 = control-ref of="Methods"() -> (w745:refnum<vi>)
                    n437 = local read "LastSample"() -> (w746:i32)
                    n438 = local read "Comments"() -> (w742:string)
                    n439 = local read "ProjectID"() -> (w741:string)
                    n440 = Bundle("element"=w736, "grainSize"=w728, "element"=w735, "barrelLength"=w732, w734, "element"=w731) -> (w737:T33)  [unwired: 1 out]
                    n441 = call "Dropdown Selection (SubVI).vi"("reference"=w745) -> ("element"=w744:string)
                    n442 = Cluster To Array(cluster=w737) -> (array=w730:string[])
                    n443 = Increment(x=w746) -> (x+1=w743:i32)
                  }
                }
              }
            }
            n444 = Get Date/Time String() -> (date string=w329:string)  [unwired: 3 in, 1 out]
          }
          frame True {
            w762 = ""
            w754 = 16  # dimensions
            w757 = 5  # SampleID
            # "date"
            # "method"
            # "general"
            # "remark"
            # "threat"
            # "shots"
            # "sample"
            # "results"
            # "range"
            # "fabric"
            # "query db with the entered record number and use result to populate the xlt"
            n445 = Not(x=w820) -> (.not. x?=w819:bool)
            n446 = local write "lookupRec"(w819) -> ()
            n447 = Format Into String(format string="SELECT * FROM Experiments\nWHERE expt=%d;" ("query string"), error in=w786, "Record #") -> (resulting string=w816:string, error out=w787:errorcluster)  [unwired: 1 in]
            n448 = call "Fetch Data (SubVI).vi"("error IN"=w787, "query string"=w816) -> ("error OUT"=w785:errorcluster, "recordset data"=w818:string[][])  [unwired: 4 out]
            n449 = Index Array(array=w818) -> (element=w756:string[])  [unwired: 2 in]
            n450 = Index Array(array=w756, index=111) -> (element=w789:string)
            n451 = local read "Set#1 Separation"() -> (w803:sgl)
            n452 = call "Load Shots (SubVI).vi"("Record #"="Record #", "Method"=w789) -> ("Shot Array"=w811:string[][], "AvgDef"=w794:dbl)  [unwired: 1 in]
            n453 = local read "mid_to_targ_dist"() -> (w806:sgl)
            n454 = local read "Barrel to Screen"() -> (w809:sgl)
            n455 = Format Into String(w794) -> (resulting string=w792:string)  [unwired: 3 in, 1 out]
            n456 = Match Pattern(string=w789, regular expression="N.I.J.") -> (offset past match=w791:i32)  [unwired: 4 out]
            n457 = Greater Or Equal To 0?(x=w791) -> (x >= 0?=w788:bool)
            n458 = case shown="False" w788 {
              tunnel: [w831 w832] -> w793
              tunnel: w792 -> [w828 w834]
              tunnel: w756 -> [w830 _]
              frame False {
                n459 = Index Array(array=w830, index #1=124 ("index"), index #2=149 ("index"), index #5=145 ("index")) -> (element #1=w829:string, element #2=w827:string, element #3=w826:string, element #4=w822:string, element #5=w823:string)  [unwired: 2 in]
                n460 = Build Array(w829, w827, w826, w822, w823, w828) -> (w831:string[])
              }
              frame True {
                w833 = "" ("Empty String Constant")
                n461 = Build Array(w833, w833, w833, w833, w833, w834, w834) -> (w832:string[])
              }
            }
            n462 = Divide(x=w803, y=sgl 2.0) -> (x/y=w808:sgl)
            n463 = Add(x=w809, y=w806) -> (x+y=w802:sgl)
            n464 = Subtract(x=w809, y=w808) -> (x-y=w807:sgl)
            n465 = Subtract(x=w806, y=w808) -> (x-y=w805:sgl)
            n466 = Index Array(array=w756, index #1=120 ("index"), index #2=119 ("index"), index #3=127 ("index"), index #4=12 ("index"), index #5=7 ("index")) -> (element #1=w774:string, element #2=w772:string, element #3=w771:string, element #4=w768:string, element #5=w767:string)
            n467 = Index Array(array=w756, index #1=113 ("index"), index #2=112 ("index"), index #3=103 ("index")) -> (element #1=w783:string, element #2=w782:string, element #3=w781:string, element #4=w780:string, element #5=w776:string)  [unwired: 2 in]
            n468 = Format Into String(w802) -> (resulting string=w801:string)  [unwired: 3 in, 1 out]
            n469 = Format Into String(w807) -> (resulting string=w800:string)  [unwired: 3 in, 1 out]
            n470 = Format Into String(w803) -> (resulting string=w799:string)  [unwired: 3 in, 1 out]
            n471 = Format Into String(w805) -> (resulting string=w798:string)  [unwired: 3 in, 1 out]
            n472 = Format Into String(w806) -> (resulting string=w797:string)  [unwired: 3 in, 1 out]
            n473 = Index Array(array=w756, index #1=w757, index #2=w754, index #3=147 ("index"), index #5=148 ("index")) -> (element #1=w755:string, element #2=w752:string, element #3=w751:string, element #5=w748:string)  [unwired: 1 in, 1 out]
            n474 = Build Array(w774, w772, w771, "", w768, w767) -> (w773:string[])
            n475 = Build Array(w801, w800, w799, w798, w797, w783, w782, w781, w780, w776) -> (w796:string[])
            n476 = Index Array(array=w756, index #1=4 ("index"), index #2=111 ("index")) -> (element #1=w763:string, element #2=w760:string)
            n477 = Index Array(array=w756, index=107) -> (element=w812:string)
            n478 = Build Array(w755, w752, w751, "", w748) -> (w753:string[])
            n479 = Index Array(array=w756, index=2) -> (element=w758:string)
            n480 = call "Get Model Construction.vi"("panel record"=w756) -> ("Fabric Array"=w810:string[][])
            n481 = Build Array(w793) -> (w813:string[][])
          }
        }
        n482 = To Variant(anything=w324) -> (Variant=w318:variant)
        n483 = To Variant(anything=w323) -> (Variant=w317:variant)
        n484 = To Variant(anything=w322) -> (Variant=w316:variant)
        n485 = To Variant(anything=w321) -> (Variant=w315:variant)
        n486 = To Variant(anything=w320) -> (Variant=w314:variant)
        n487 = To Variant(anything=w319) -> (Variant=w313:variant)
        n488 = To Variant(anything=w306) -> (Variant=w312:variant)
        n489 = To Variant(anything=w305) -> (Variant=w311:variant)
        n490 = To Variant(anything=w304) -> (Variant=w310:variant)
        n491 = To Variant(anything=w303) -> (Variant=w307:variant)
        n492 = To Variant(anything=w302) -> (Variant=w308:variant)
        n493 = To Variant(anything=w295) -> (Variant=w309:variant)
        n494 = To Variant(anything=w293) -> (Variant=w294:variant)
        n495 = call "TestReport_XL.vi"("Enable"=TRUE, "blockFabric"=w318, "blockRange"=w317, "blockResults"=w316, "blockSample"=w315, "blockShotTbl"=w314, "error in (no error)"=w298, "blockThreat"=w313, "testDate"=w294, "method"=w312, "projName"=w311, "projNum"=w310, "recNum"=w307, "remark"=w308, "standard"=w309) -> ("error out"=w325:errorcluster)  [unwired: 4 in, 8 out]
        n496 = call <vilib>:"Simple Error Handler.vi"("error in (no error)"=w325) -> ("error out"=w327:errorcluster)  [unwired: 1 in, 7 out]
        n497 = case shown="No Error" w327 {
          selector: w327 -> [w835 w837]
          tunnel: [w835 w837] -> w296
          frame No Error {
            n498 = One Button Dialog(message=" V50 Ballistic Test Report is ready") -> ()  [unwired: 2 out]
          }
          frame Error {
          }
        }
      }
      frame 3 {
        w867 = TRUE  # Enable
        # "The custom Excel template file is \nexpected in the C:\\Ballistics folder."
        n499 = stacked-sequence {
          tunnel: [_ _ _ _ _ w1058] -> w860
          tunnel: [_ w931 _ _ _ _] -> w864
          tunnel: [_ _ _ _ w1015 _] -> w861
          tunnel: [_ _ _ w982 _ _] -> w862
          tunnel: [_ _ w953 _ _ _] -> w863
          tunnel: [w875 _ _ _ _ _] -> w865
          tunnel: [_ _ _ _ _ w1079] -> w847
          tunnel: [_ _ _ _ _ "" ("projNum")] -> w846
          tunnel: [_ _ _ _ _ w1074] -> w845
          tunnel: [_ _ _ _ _ w1078] -> w844
          tunnel: [_ _ _ _ _ w1077] -> w843
          tunnel: [_ _ _ _ _ w1076] -> w842
          tunnel: w841 -> [_ _ w952 _ w1008 _]
          frame #0 {
            # "FABRIC"
            n500 = local read "fab1_totalWt"() -> (w878:sgl)
            n501 = local read "fab3_totalWt"() -> (w880:sgl)
            n502 = local read "fab5_totalWt"() -> (w882:sgl)
            n503 = global read "BIMS_Collector Globals.vi" "LayerStitchTypeRefs"() -> (w870:refnum<vi>[])
            n504 = global read "BIMS_Collector Globals.vi" "SampleAttribs"() -> (w871:T24)
            n505 = global read "BIMS_Collector Globals.vi" "SampleStyles"() -> (w873:refnum<vi>[])
            n506 = local read "fab2_totalWt"() -> (w879:sgl)
            n507 = local read "fab4_totalWt"() -> (w881:sgl)
            n508 = local read "fab6_totalWt"() -> (w883:sgl)
            n509 = global read "BIMS_Collector Globals.vi" "LayerSpecs"() -> (w872:T25)
            n510 = global read "BIMS_Collector Globals.vi" "Mfrs"() -> (w874:refnum<vi>[])
            n511 = Build Array(w878, w879, w880, w881, w882, w883) -> (w877:sgl[])
            n512 = for {
              tunnel: w877 -> [w885] mode=indexing
              tunnel: [w891] -> w876 mode=indexing
              tunnel: w871 -> [w889] mode=indexing
              tunnel: w872 -> [w888] mode=indexing
              tunnel: w874 -> [w887] mode=indexing
              tunnel: w873 -> [w886] mode=indexing
              tunnel: w870 -> [w884] mode=indexing
              n513 = Less Or Equal To 0?(x=w885) -> (x <= 0?=w890:bool)
              n514 = case shown="False" w890 {
                tunnel: [w913 w915] -> w891
                tunnel: w889 -> [w912 _]
                tunnel: w888 -> [w897 _]
                tunnel: w887 -> [w906 _]
                tunnel: w886 -> [w903 _]
                tunnel: w885 -> [w896 _]
                tunnel: w884 -> [w892 _]
                frame False {
                  n515 = Unbundle By Name(w897) -> ("numOfPlies"=w895:i32, "LotNum"=w909:string, "RollNum"=w910:string)
                  n516 = Unbundle By Name(w912) -> ("internal_ID"=w900:string, "fiber"=w901:string, "denier"=w908:string, "pick"=w907:string, "weave"=w898:string, "finish"=w899:string, "ozPerYd2"=w911:string)
                  n517 = Format Into String(w895) -> (resulting string=w905:string)  [unwired: 3 in, 1 out]
                  n518 = call "Dropdown Selection (SubVI).vi"("reference"=w906) -> ("element"=w904:string)
                  n519 = call "Dropdown Selection (SubVI).vi"("reference"=w903) -> ("element"=w902:string)
                  n520 = call "Dropdown Selection (SubVI).vi"("reference"=w892) -> ("element"=w893:string)
                  n521 = Format Into String(w896) -> (resulting string=w894:string)  [unwired: 3 in, 1 out]
                  n522 = Build Array(w905, w904, w902, w900, w901, w908, w907, w898, w899, w909, w910, w911, w894, w893) -> (w913:string[])
                }
                frame True {
                  n523 = call <vilib>:"Space Constant.vi"() -> ("String"=w916:string)
                  n524 = Initialize Array(w916, 12 ("dimension size")) -> (w915:string[])
                }
              }
            }
            n525 = Transpose 2D Array(2D array=w876) -> (transposed array=w875:string[][])
          }
          frame #1 {
            w917 = "%.1f" ("format string")
            # "muzzel / midpoint"
            # "muzzle / scr#1"
            # "muzzle / target"
            # "scr#2 / target"
            # "RANGE"
            n526 = local read "Set#1 Separation"() -> (w924:sgl)
            n527 = local read "mid_to_targ_dist"() -> (w921:sgl)
            n528 = local read "Barrel to Screen"() -> (w918:sgl)
            n529 = local read "clayAverage"() -> (w939:sgl)
            n530 = Divide(x=w924, y=sgl 2.0) -> (x/y=w919:sgl)
            n531 = local read "RoomHum"() -> (w934:sgl)
            n532 = local read "clayTemp"() -> (w937:sgl)
            n533 = local read "clayCalib"() -> (w940:string)
            n534 = local read "RoomT"() -> (w935:sgl)
            n535 = Add(x=w918, y=w921) -> (x+y=w925:sgl)
            n536 = Subtract(x=w918, y=w919) -> (x-y=w920:sgl)
            n537 = Subtract(x=w921, y=w919) -> (x-y=w922:sgl)
            n538 = Format Into String(w925) -> (resulting string=w926:string)  [unwired: 3 in, 1 out]
            n539 = Format Into String(w920) -> (resulting string=w927:string)  [unwired: 3 in, 1 out]
            n540 = Format Into String(w924) -> (resulting string=w928:string)  [unwired: 3 in, 1 out]
            n541 = Format Into String(w922) -> (resulting string=w929:string)  [unwired: 3 in, 1 out]
            n542 = Format Into String(w921) -> (resulting string=w930:string)  [unwired: 3 in, 1 out]
            n543 = Format Into String(w934) -> (resulting string=w932:string)  [unwired: 3 in, 1 out]
            n544 = Format Into String(format string=w917, w935) -> (resulting string=w933:string)  [unwired: 2 in, 1 out]
            n545 = Format Into String(format string=w917, w937) -> (resulting string=w936:string)  [unwired: 2 in, 1 out]
            n546 = Format Into String(format string=w917, w939) -> (resulting string=w938:string)  [unwired: 2 in, 1 out]
            n547 = Bundle(w926, w927, w928, w929, w930, w932, w933, w936, "clayCalib"=w940, w938) -> (w941:T26)  [unwired: 1 out]
            n548 = Cluster To Array(cluster=w941) -> (array=w931:string[])
          }
          frame #2 {
            # "RESULTS"
            n549 = control-ref of="Methods"() -> (w942:refnum<vi>)
            n550 = call "Dropdown Selection (SubVI).vi"("reference"=w942) -> ("element"=w943:string)
            n551 = for {
              tunnel: w952 -> [w980] mode=indexing
              tunnel: [w979] -> w951 mode=indexing
              tunnel: [w978] -> w950
              i -> [w978]
              n552 = Unbundle By Name(w980) -> ("BackFace\nDepth"=w979:sgl)
            }
            n553 = Increment(x=w950) -> (x+1=w948:i32)
            n554 = Add Array Elements(numeric array=w951) -> (sum=w949:sgl)
            n555 = To Single Precision Float(number=w948) -> (single precision float=w947:sgl)
            n556 = Divide(x=w949, y=w947) -> (x/y=w946:sgl)
            n557 = Format Into String(format string="%1.1f", w946) -> (resulting string=w945:string)  [unwired: 2 in, 1 out]
            n558 = case shown="\"V50\"" w943 {
              tunnel: [w968 w977] -> w955
              tunnel: w945 -> [w956 w976]
              frame "V50" {
                w962 = "%1d" ("format string")
                n559 = local read "Z.M.R."() -> (w960:sgl)
                n560 = Less Than 0?(x=w960) -> (x < 0?=w961:bool)
                n561 = local read "rangeOfResults"() -> (w964:i32)
                n562 = local read "computed_V50"() -> (w967:sgl)
                n563 = local read "lowComplete"() -> (w965:i32)
                n564 = local read "highPartial"() -> (w966:i32)
                n565 = case shown="True" w961 {
                  tunnel: w960 -> [w973 _]
                  tunnel: [w973 sgl 0.0 ("Z.M.R.")] -> w959
                  frame False {
                  }
                  frame True {
                  }
                }
                n566 = Format Into String(format string="%1.1f", w967) -> (resulting string=w971:string)  [unwired: 2 in, 1 out]
                n567 = Format Into String(format string=w962, w966) -> (resulting string=w970:string)  [unwired: 2 in, 1 out]
                n568 = Format Into String(format string=w962, w965) -> (resulting string=w969:string)  [unwired: 2 in, 1 out]
                n569 = Format Into String(format string=w962, w964) -> (resulting string=w972:string)  [unwired: 2 in, 1 out]
                n570 = Format Into String(format string="%1.1f", w959) -> (resulting string=w958:string)  [unwired: 2 in, 1 out]
                n571 = Bundle(w971, w970, w969, w972, w958, w956, w956) -> (w968:T27)  [unwired: 1 out]
              }
              frame Default {
                w975 = "" ("Empty String Constant")
                n572 = Bundle(w975, w975, w975, w975, w975, w976, w976) -> (w977:T27)  [unwired: 1 out]
              }
            }
            n573 = Cluster To Array(cluster=w955) -> (array=w954:string[])
            n574 = Build Array(w954) -> (w953:string[][])
          }
          frame #3 {
            # "PB Req"
            # "SAMPLE"
            n575 = control-ref of="Methods"() -> (w983:refnum<vi>)
            n576 = call "Dropdown Selection (SubVI).vi"("reference"=w983) -> ("element"=w985:string)
            n577 = Equal?(x=w985, y="V50") -> (x = y?=w984:bool)
            n578 = local read "totalSampleWt"() -> (w995:sgl)
            n579 = case shown="True" w984 {
              tunnel: ["n/a" w1005] -> w989
              frame False {
              }
              frame True {
                n580 = local read "minV50"() -> (w1004:i32)
                n581 = Format Into String(w1004) -> (resulting string=w1005:string)  [unwired: 3 in, 1 out]
              }
            }
            n582 = local read "Type of work"() -> (w981:string)
            n583 = control-ref of="SampleDimensions"() -> (w1001:refnum<vi>)
            n584 = control-ref of="SampleCoverings"() -> (w1002:refnum<vi>)
            n585 = control-ref of="Models"() -> (w988:refnum<vi>)
            n586 = local read "serialNum"() -> (w997:string)
            n587 = local read "SampleID"() -> (w999:string)
            n588 = local read "Thickness"() -> (w992:dbl)
            n589 = local read "totalBAW"() -> (w991:sgl)
            n590 = call "Dropdown Selection (SubVI).vi"("reference"=w1001) -> ("element"=w998:string)
            n591 = call "Dropdown Selection (SubVI).vi"("reference"=w988) -> ("element"=w987:string)
            n592 = call "Dropdown Selection (SubVI).vi"("reference"=w1002) -> ("element"=w996:string)
            n593 = Format Into String(w995) -> (resulting string=w994:string)  [unwired: 3 in, 1 out]
            n594 = Format Into String(w992) -> (resulting string=w993:string)  [unwired: 3 in, 1 out]
            n595 = Format Into String(w991) -> (resulting string=w990:string)  [unwired: 3 in, 1 out]
            n596 = Bundle("SampleID"=w999, "element"=w998, "Type of work"=w981, "serialNum"=w997, "element"=w987, w994, w993, w990, "element"=w996, w989) -> (w1000:T28)  [unwired: 1 out]
            n597 = Cluster To Array(cluster=w1000) -> (array=w982:string[])
          }
          frame #4 {
            # "SHOT TABLE"
            n598 = control-ref of="Methods"() -> (w1007:refnum<vi>)
            n599 = call "Dropdown Selection (SubVI).vi"("reference"=w1007) -> ("element"=w1006:string)
            n600 = for {
              tunnel: w1008 -> [w1047] mode=indexing
              shift-right: [w1024] -> _
              shift-left: T18 [] -> [w1026]
              tunnel: [w1024] -> w1011
              tunnel: w1006 -> [w1020]
              n601 = Unbundle By Name(w1047) -> ("shot order"=w1046:i32, "Powder Loading"=w1045:sgl, "Uncorrected Impact"=w1044:sgl, "UncorrectedRed_PB"=w1043:sgl, "UncorrectedAvgVel_PB"=w1042:sgl, "velLoss_PB"=w1041:sgl, "strikeVel_PB"=w1040:sgl, "SHOT STATUS"=w1029:u16, "usedv50"=w1039:bool, "Shot Angle"=w1021:u16, "BackFace\nDepth"=w1022:sgl)
              n602 = case shown="\"V50\"" w1020 {
                tunnel: w1039 -> [w1049 _]
                tunnel: [w1048 w1053] -> w1038
                tunnel: w1021 -> [_ w1052]
                frame "V50" {
                  n603 = case shown="True" w1049 {
                    tunnel: ["" ("Empty String Constant") "*"] -> w1048
                    frame False {
                    }
                    frame True {
                    }
                  }
                }
                frame Default {
                  n604 = Format Into String(w1052) -> (resulting string=w1053:string)  [unwired: 3 in, 1 out]
                }
              }
              n605 = case shown="1" w1029 {
                tunnel: ["P" "C"] -> w1028
                frame 0, Default {
                }
                frame 1 {
                }
              }
              n606 = Format Into String(format string="%2d", w1046) -> (resulting string=w1031:string)  [unwired: 2 in, 1 out]
              n607 = Format Into String(w1045) -> (resulting string=w1032:string)  [unwired: 3 in, 1 out]
              n608 = Format Into String(w1044) -> (resulting string=w1033:string)  [unwired: 3 in, 1 out]
              n609 = Format Into String(w1043) -> (resulting string=w1034:string)  [unwired: 3 in, 1 out]
              n610 = Format Into String(w1042) -> (resulting string=w1035:string)  [unwired: 3 in, 1 out]
              n611 = Format Into String(w1041) -> (resulting string=w1036:string)  [unwired: 3 in, 1 out]
              n612 = Format Into String(w1040) -> (resulting string=w1037:string)  [unwired: 3 in, 1 out]
              n613 = Format Into String(w1022) -> (resulting string=w1030:string)  [unwired: 3 in, 1 out]
              n614 = Build Array(w1031, w1032, w1033, w1034, w1035, w1036, w1037, w1028, w1038, w1030) -> (w1025:string[])
              n615 = Array To Cluster(array=w1025) -> (cluster=w1027:T30)
              n616 = Build Array (concatenate)(w1026, w1027) -> (w1024:T18)
            }
            n617 = Array Size(array=w1011) -> (size(s)=w1013:i32)
            n618 = Equal To 0?(x=w1013) -> (x = 0?=w1009:bool)
            n619 = case shown="True" w1009 {
              tunnel: [w1016 T18 [{"[0]"="", "[1]"="", "[2]"="", "[3]"="", "[4]"="", "[5]"="", "[6]"="", "[7]"="", "[8]"="", "[9]"=""}]] -> w1010
              tunnel: w1011 -> [w1016 _]
              frame False {
              }
              frame True {
              }
            }
            n620 = Sort 1D Array(array=w1010) -> (sorted array=w1012:T18)
            n621 = for {
              tunnel: w1012 -> [w1019] mode=indexing
              tunnel: [w1018] -> w1015 mode=indexing
              n622 = Cluster To Array(cluster=w1019) -> (array=w1018:string[])
            }
          }
          frame #5 {
            # "THREAT"
            # "Range # (supports a PB reporting requirement)"
            # "Project Name goes here.\nSupports a PB reporting requirement."
            # "GENERAL"
            n623 = local read "threatDetails"() -> (w1057:T1)
            n624 = Unbundle By Name(w1057) -> ("barrelLength"=w1061:string)
            n625 = Unbundle By Name(w1057) -> ("grainSize"=w1056:string)
            n626 = local read "Shot Angle"() -> (w1062:u16)
            n627 = control-ref of="WeaponTypes"() -> (w1071:refnum<vi>)
            n628 = control-ref of="ThreatGroups"() -> (w1070:refnum<vi>)
            n629 = control-ref of="PowderTypes"() -> (w1069:refnum<vi>)
            n630 = control-ref of="Recorders"() -> (w1072:refnum<vi>)
            n631 = control-ref of="Shooters"() -> (w1073:refnum<vi>)
            n632 = Format Into String(w1062) -> (resulting string=w1063:string)  [unwired: 3 in, 1 out]
            n633 = call "Dropdown Selection (SubVI).vi"("reference"=w1071) -> ("element"=w1067:string)
            n634 = call "Dropdown Selection (SubVI).vi"("reference"=w1070) -> ("element"=w1066:string)
            n635 = call "Dropdown Selection (SubVI).vi"("reference"=w1069) -> ("element"=w1065:string)
            n636 = call "Dropdown Selection (SubVI).vi"("reference"=w1072) -> ("element"=w1064:string)
            n637 = call "Dropdown Selection (SubVI).vi"("reference"=w1073) -> ("element"=w1060:string)
            n638 = Bundle("element"=w1067, "element"=w1066, "grainSize"=w1056, "element"=w1065, "barrelLength"=w1061, w1063, "element"="1", "element"=w1060, "element"=w1064) -> (w1068:T32)  [unwired: 1 out]
            n639 = Cluster To Array(cluster=w1068) -> (array=w1058:string[])
            n640 = local read "Comments"() -> (w1077:string)
            n641 = local read "ProjectID"() -> (w1074:string)
            n642 = local read "LastSample"() -> (w1082:i32)
            n643 = control-ref of="TestStandards"() -> (w1081:refnum<vi>)
            n644 = control-ref of="Methods"() -> (w1080:refnum<vi>)
            n645 = call "Dropdown Selection (SubVI).vi"("reference"=w1081) -> ("element"=w1076:string)
            n646 = call "Dropdown Selection (SubVI).vi"("reference"=w1080) -> ("element"=w1079:string)
            n647 = Increment(x=w1082) -> (x+1=w1078:i32)
          }
        }
        n648 = To Variant(anything=w865) -> (Variant=w859:variant)
        n649 = To Variant(anything=w864) -> (Variant=w858:variant)
        n650 = To Variant(anything=w863) -> (Variant=w857:variant)
        n651 = To Variant(anything=w862) -> (Variant=w856:variant)
        n652 = To Variant(anything=w861) -> (Variant=w855:variant)
        n653 = To Variant(anything=w860) -> (Variant=w854:variant)
        n654 = To Variant(anything=w847) -> (Variant=w853:variant)
        n655 = To Variant(anything=w846) -> (Variant=w852:variant)
        n656 = To Variant(anything=w845) -> (Variant=w851:variant)
        n657 = To Variant(anything=w844) -> (Variant=w848:variant)
        n658 = To Variant(anything=w843) -> (Variant=w849:variant)
        n659 = To Variant(anything=w842) -> (Variant=w850:variant)
        n660 = call "TestReport_XL.vi"("Enable"=w867, "blockFabric"=w859, "blockRange"=w858, "blockResults"=w857, "blockSample"=w856, "blockShotTbl"=w855, "error in (no error)"=w839, "blockThreat"=w854, "method"=w853, "projName"=w852, "projNum"=w851, "recNum"=w848, "remark"=w849, "standard"=w850) -> ("error out"=w866:errorcluster)  [unwired: 5 in, 8 out]
        n661 = call <vilib>:"Simple Error Handler.vi"("error in (no error)"=w866) -> ("error out"=w868:errorcluster)  [unwired: 1 in, 7 out]
        n662 = case shown="No Error" w868 {
          selector: w868 -> [w1083 w1085]
          tunnel: [w1083 w1085] -> w838
          frame No Error {
            n663 = One Button Dialog(message=" VsVr Ballistic Test Report is ready") -> ()  [unwired: 2 out]
          }
          frame Error {
          }
        }
      }
      frame 4 {
        # "This section saves the shots to the data base"
        n664 = stacked-sequence {
          seq-local: [w1151 _ _] -> [_ w1237 _]
          seq-local: [w1153 _ _] -> [_ w1234 _]
          seq-local: [_ w1222 _] -> [_ _ w1251]
          seq-local: [_ w1224 _] -> [_ _ w1250]
          seq-local: [w1149 _ _] -> [_ _ w1243]
          seq-local: [w1123 _ _] -> [_ w1180 _]
          tunnel: [_ _ w1245] -> w1091
          tunnel: [_ _ w1248] -> w1092
          tunnel: w1087 -> [_ w1189 w1242]
          tunnel: w1089 -> [w1125 _ _]
          tunnel: ["SampleDescrip" _ _] -> _
          tunnel: ["Areal Density" _ _] -> _
          tunnel: ["Areal density text" _ _] -> _
          tunnel: ["SoftwareVersion" _ _] -> _
          tunnel: ["Fabric Description" _ _] -> _
          tunnel: ["Threat" _ _] -> _
          tunnel: ["old threat" _ _] -> _
          tunnel: ["line direction map" _ _] -> _
          tunnel: ["Methods" _ _] -> _
          tunnel: ["SampleCoverings" _ _] -> _
          tunnel: ["Ballisticians" _ _] -> _
          tunnel: ["Submitters" _ _] -> _
          tunnel: ["SampleDimensions" _ _] -> _
          tunnel: ["PowderTypes" _ _] -> _
          tunnel: ["SampleTypes" _ _] -> _
          tunnel: ["TestConditions" _ _] -> _
          tunnel: ["ModelMfrs" _ _] -> _
          tunnel: ["Assemblers" _ _] -> _
          tunnel: ["N.I.J" _ _] -> _
          tunnel: ["SampleClamping" _ _] -> _
          tunnel: ["FrontLayer" _ _] -> _
          tunnel: ["BackLayer" _ _] -> _
          frame #0 {
            # "Legacy requirements:"
            # "Shared requirements:"
            n665 = local read "fab1_totalWt"() -> (w1161:sgl)
            n666 = local read "fab2_totalWt"() -> (w1160:sgl)
            n667 = local read "fab3_totalWt"() -> (w1159:sgl)
            n668 = local read "fab4_totalWt"() -> (w1158:sgl)
            n669 = local read "fab5_totalWt"() -> (w1157:sgl)
            n670 = local read "fab6_totalWt"() -> (w1156:sgl)
            n671 = flat-sequence {
              tunnel: ["TestStandards"] -> _
              tunnel: ["Shooters"] -> _
              tunnel: ["Recorders"] -> _
              tunnel: ["WeaponTypes"] -> _
              tunnel: ["Models"] -> _
              tunnel: ["serialNum"] -> _
              tunnel: ["layerStitch_1"] -> _
              tunnel: ["layerStitch_2"] -> _
              tunnel: ["layerStitch_3"] -> _
              tunnel: ["layerStitch_4"] -> _
              tunnel: ["layerStitch_5"] -> _
              tunnel: ["layerStitch_6"] -> _
              tunnel: ["minV50"] -> _
              frame #0 {
                # "PB-only requirements:"
              }
            }
            n672 = Build Array(w1161, w1160, w1159, w1158, w1157, w1156) -> (w1155:sgl[])
            n673 = call "SQL Statement for Sample Descritpion.vi"("error IN"=w1125, "Layer Weight Array"=w1155, "VALUES clause IN"=" VALUES (%d " ("SQL statement IN"), "INSERT clause IN"="INSERT INTO Experiments " ("SQL statement IN")) -> ("error OUT"=w1124:errorcluster, "VALUES clause OUT"=w1154:string, "INSERT clause OUT"=w1152:string)  [unwired: 1 out]
            n674 = local read "LastSample"() -> (w1150:i32)
            n675 = Increment(x=w1150) -> (x+1=w1149:i32)
            n676 = local read "rangeOfResults"() -> (w1127:i32)
            n677 = local read "lowComplete"() -> (w1128:i32)
            n678 = local read "clayAverage"() -> (w1130:sgl)
            n679 = local read "highPartial"() -> (w1129:i32)
            n680 = control-ref of="SampleClamping"() -> (w1122:refnum<vi>)
            n681 = control-ref of="BackLayer"() -> (w1098:refnum<vi>)
            n682 = control-ref of="FrontLayer"() -> (w1097:refnum<vi>)
            n683 = control-ref of="Ballisticians"() -> (w1144:refnum<vi>)
            n684 = control-ref of="Shooters"() -> (w1140:refnum<vi>)
            n685 = control-ref of="Recorders"() -> (w1139:refnum<vi>)
            n686 = control-ref of="Submitters"() -> (w1143:refnum<vi>)
            n687 = control-ref of="SampleCoverings"() -> (w1136:refnum<vi>)
            n688 = control-ref of="ThreatGroups"() -> (w1135:refnum<vi>)
            n689 = call "Dropdown Selection (SubVI).vi"("reference"=w1144) -> ("element"=w1142:string)
            n690 = call "Dropdown Selection (SubVI).vi"("reference"=w1140) -> ("element"=w1138:string)
            n691 = call "Dropdown Selection (SubVI).vi"("reference"=w1139) -> ("element"=w1137:string)
            n692 = call "Dropdown Selection (SubVI).vi"("reference"=w1143) -> ("element"=w1141:string)
            n693 = call "Dropdown Selection (SubVI).vi"("reference"=w1136) -> ("element"=w1134:string)
            n694 = call "Dropdown Selection (SubVI).vi"("reference"=w1135) -> ("element"=w1133:string)
            n695 = call "Dropdown Selection (SubVI).vi"("reference"=w1122) -> ("element"=w1121:string)
            n696 = call "Dropdown Selection (SubVI).vi"("reference"=w1098) -> ("element"=w1096:string)
            n697 = call "Dropdown Selection (SubVI).vi"("reference"=w1097) -> ("element"=w1095:string)
            n698 = Concatenate Strings(w1152, ", expt, [date], Ballistician1, Ballistician2, Ballistician3, Submitter1, SampleCovering, ProjectileType, ClayTemp, ClayCalibration, ClayAvgThickness, highPartial, lowComplete, rangeOfResults, clamping, FrontPly, BackPly," ("Substring")) -> (w1151:string)
            n699 = Format Into String(format string=", %d, #%s#, '%s', '%s', '%s', '%s', '%s', '%s', %.1f, '%s', %.1f, %d, %d, %d, '%s', '%s', '%s'" ("Format String"), initial string=w1154, error in=w1124, w1149, "currentDateTime", w1142, w1138, w1137, w1141, w1134, w1133, "clayTemp", "clayCalib", w1130, w1129, w1128, w1127, w1121, w1096, w1095) -> (resulting string=w1153:string, error out=w1123:errorcluster)
          }
          frame #1 {
            w1236 = " Angle, Conditions, SampleType, ThreatGrain, ThreatDetail, V50dc, V50, maker, thickness, powder, numshots, backing, totalnumberplys, testcomments, NIJ1, method, temperature, humidity, Dimensions, zmr, ProjectID, SampleID, panelmaker, panelWeight, totalBAW)"  # INSERT clause continued
            # "Although shot angle is defined for the overall\nexperiment, it is also recorded for each shot."
            n700 = local read "computed_V50"() -> (w1232:sgl)
            n701 = local read "Drag Corrected"() -> (w1227:bool)
            n702 = local read "Impact factor"() -> (w1229:sgl)
            n703 = Array Size(array=w1189) -> (size(s)=w1220:i32)
            n704 = Select(t=w1229, s=w1227, f=sgl 1.0) -> (s? t:f=w1228:sgl)
            n705 = Divide(x=w1232, y=w1228) -> (x/y=w1231:sgl)
            n706 = control-ref of="ModelMfrs"() -> (w1215:refnum<vi>)
            n707 = control-ref of="PowderTypes"() -> (w1213:refnum<vi>)
            n708 = call "Dropdown Selection (SubVI).vi"("reference"=w1215) -> ("element"=w1214:string)
            n709 = call "Dropdown Selection (SubVI).vi"("reference"=w1213) -> ("element"=w1197:string)
            n710 = local read "GrainSize"() -> (w1178:u16)
            n711 = local read "Z.M.R."() -> (w1203:sgl)
            n712 = local read "Shot Angle"() -> (w1191:u16)
            n713 = Less Than 0?(x=w1203) -> (x < 0?=w1202:bool)
            n714 = local read "totalNumLayers"() -> (w1219:i32)
            n715 = control-ref of="ThreatDetails"() -> (w1175:refnum<vi>)
            n716 = control-ref of="SampleTypes"() -> (w1185:refnum<vi>)
            n717 = control-ref of="TestConditions"() -> (w1204:refnum<vi>)
            n718 = control-ref of="SampleBackings"() -> (w1212:refnum<vi>)
            n719 = Format Into String(w1178) -> (resulting string=w1177:string)  [unwired: 3 in, 1 out]
            n720 = local read "totalBAW"() -> (w1205:sgl)
            n721 = case shown="True" w1202 {
              tunnel: w1203 -> [w1240 _]
              tunnel: [w1240 sgl 0.0 ("Z.M.R.")] -> w1201
              frame False {
              }
              frame True {
              }
            }
            n722 = control-ref of="SampleDimensions"() -> (w1208:refnum<vi>)
            n723 = control-ref of="N.I.J"() -> (w1210:refnum<vi>)
            n724 = control-ref of="Methods"() -> (w1195:refnum<vi>)
            n725 = control-ref of="Assemblers"() -> (w1206:refnum<vi>)
            n726 = call "Dropdown Selection (SubVI).vi"("reference"=w1175) -> ("element"=w1176:string)
            n727 = call "Dropdown Selection (SubVI).vi"("reference"=w1185) -> ("element"=w1184:string)
            n728 = call "Dropdown Selection (SubVI).vi"("reference"=w1204) -> ("element"=w1190:string)
            n729 = call "Dropdown Selection (SubVI).vi"("reference"=w1212) -> ("element"=w1211:string)
            n730 = Equal?(x=w1177, y="") -> (x = y?=w1199:bool)
            n731 = call "Dropdown Selection (SubVI).vi"("reference"=w1210) -> ("element"=w1209:string)
            n732 = call "Dropdown Selection (SubVI).vi"("reference"=w1195) -> ("element"=w1194:string)
            n733 = call "Dropdown Selection (SubVI).vi"("reference"=w1208) -> ("element"=w1207:string)
            n734 = call "Dropdown Selection (SubVI).vi"("reference"=w1206) -> ("element"=w1196:string)
            n735 = case shown="False" w1199 {
              tunnel: [w1238 "0" ("element")] -> w1198
              tunnel: w1177 -> [w1238 _]
              frame False {
              }
              frame True {
              }
            }
            n736 = call "Prepare DB Connect Path (SubVI).vi"("connectString"=path "BIMS_Collector.udl", "error in"=w1180) -> ("appended path"=w1179:path, "error out"=w1181:errorcluster)  [unwired: 1 out]
            n737 = Format Into String(format string=", %d, '%s', '%s', '%s', '%s', %.4f, %.1f, '%s', %.4f, '%s', %d, '%s', %d, '%s', '%s', '%s', %.1f, %.1f, '%s', %.1f, '%s', '%s', '%s', %.1f, %.1f);" ("Format String"), initial string=w1234, error in=w1181, w1191, w1190, w1184, w1198, w1176, w1232, w1231, w1214, "Thickness", w1197, w1220, w1211, w1219, "Comments", w1209, w1194, "RoomT", "RoomHum", w1207, w1201, "ProjectID", "SampleID", w1196, "totalSampleWt", w1205) -> (resulting string=w1233:string, error out=w1183:errorcluster)
            n738 = call-poly <vilib>:"DB Tools Open Connection.vi"("error in (no error)"=w1183, "connection information"=w1179) -> ("error out"=w1192:errorcluster, "connection reference"=w1193:T34)  [unwired: 3 in, 3 out]
            n739 = Concatenate Strings(w1237, w1236, w1233) -> (w1226:string)
            n740 = call-poly <vilib>:"DB Tools Execute Query.vi"("error in (no error)"=w1192, "SQL query"=w1226, "connection reference"=w1193) -> ("error out"=w1225:errorcluster, "recordset reference"=w1223:T35)  [unwired: 1 in, 4 out]
            n741 = call-poly <vilib>:"DB Tools Free Object.vi"("error in (no error)"=w1225, "recordset reference"=w1223) -> ("error out"=w1224:errorcluster, "connection reference"=w1222:T34)  [unwired: 8 out]
          }
          frame #2 {
            # "Experiment.expt"
            n742 = local read "LastShot"() -> (w1249:i32)
            n743 = Increment(x=w1249) -> (x+1=w1247:i32)
            n744 = for {
              tunnel: w1242 -> [w1295] mode=indexing
              tunnel: w1251 -> [w1270]
              tunnel: w1250 -> [w1254]
              tunnel: [w1268] -> w1244
              tunnel: [w1269] -> w1246
              tunnel: w1247 -> [w1275]
              tunnel: [w1267] -> w1248
              tunnel: w1243 -> [w1263]
              i -> [w1267]
              w1255 = sgl 1.0 ("f")
              # "Shot.id"
              n745 = Add(x=w1275, y=w1267) -> (x+y=w1274:i32)
              n746 = Unbundle By Name(w1295) -> ("IMPACT VELOCITY"=w1281:sgl, "Redundant_Velocity"=w1260:sgl, "RESIDUAL  VELOCITY"=w1259:sgl, "Shot Description"=w1261:string, "Powder Loading"=w1285:sgl, "Barrel Temperature"=w1286:sgl, "TIME / DATE"=w1287:string, "shot order"=w1288:i32, "Shot Angle"=w1289:u16, "BackFace\nDepth"=w1290:sgl, "BackFace\nDiameter"=w1291:sgl, "SHOT STATUS"=w1293:u16, "Projectile Mass"=w1284:sgl, "usedv50"=w1283:bool, "Energy Loss (J)"=w1282:sgl, "avgVel_PB"=w1266:sgl, "velLoss_PB"=w1265:sgl, "strikeVel_PB"=w1264:sgl, "Frag Rod"=w1252:sgl)
              n747 = local read "Drag Corrected"() -> (w1257:bool)
              n748 = local read "Residual factor"() -> (w1279:sgl)
              n749 = local read "Impact factor"() -> (w1256:sgl)
              n750 = Greater Than 0?(x=w1293) -> (x > 0?=w1292:bool)
              n751 = Select(t=w1256, s=w1257, f=w1255) -> (s? t:f=w1277:sgl)
              n752 = Select(t=w1256, s=w1257, f=w1255) -> (s? t:f=w1262:sgl)
              n753 = Select(t=w1279, s=w1257, f=w1255) -> (s? t:f=w1278:sgl)
              n754 = Divide(x=w1281, y=w1277) -> (x/y=w1276:sgl)
              n755 = Divide(x=w1260, y=w1262) -> (x/y=w1258:sgl)
              n756 = Divide(x=w1259, y=w1278) -> (x/y=w1280:sgl)
              n757 = Format Into String(format string="INSERT INTO shots (impactdc, redundantdc, residualdc,  comment, loading, barreltemp, [date], [order], shotangle, bfdepth, bfdiameter, [complete], expt, id, weight,usedv50, loss, residual, impact, redundant, avgVel_PB, velLoss_PB, strikeVel_PB, fragRod)  VALUES (%.1f, %.1f, %.1f, '%s', %.4f, %.1f, #%s#, %d, %d, %.3f, %.3f, %d, %d, %d, %.4f, %d, %.4f, %.1f, %.1f, %.1f, %.1f, %.1f, %.1f, %.1f)" ("Substring"), error in=w1254, w1281, w1260, w1259, w1261, w1285, w1286, w1287, w1288, w1289, w1290, w1291, w1292, w1263, w1274, w1284, w1283, w1282, w1280, w1276, w1258, w1266, w1265, w1264, w1252) -> (resulting string=w1271:string, error out=w1253:errorcluster)  [unwired: 1 in]
              n758 = call-poly <vilib>:"DB Tools Execute Query.vi"("error in (no error)"=w1253, "SQL query"=w1271, "connection reference"=w1270) -> ("error out"=w1273:errorcluster, "recordset reference"=w1272:T35)  [unwired: 1 in, 4 out]
              n759 = call-poly <vilib>:"DB Tools Free Object.vi"("error in (no error)"=w1273, "recordset reference"=w1272) -> ("error out"=w1268:errorcluster, "connection reference"=w1269:T34)  [unwired: 8 out]
            }
            n760 = call <vilib>:"DB Tools Close Connection.vi"("error in (no error)"=w1244, "connection reference"=w1246) -> ("error out"=w1245:errorcluster)  [unwired: 5 out]
          }
        }
        n761 = local read "configPath"() -> (w1090:path)
        n762 = case shown="No Error" w1091 {
          selector: w1091 -> [w1307 w1334]
          tunnel: [-1 -1] -> w1093
          tunnel: [Collector_State."POLL" ("progState") Collector_State."POLL" ("progState")] -> w1094
          tunnel: w1092 -> [w1318 _]
          tunnel: w1090 -> [w1302 _]
          tunnel: [w1301 w1332] -> w1088
          tunnel: w1087 -> [w1299 w1331]
          tunnel: [w1297 w1331] -> w1086
          frame No Error {
            w1308 = "Data Base Parameters" ("section")
            n763 = local read "LastShot"() -> (w1319:i32)
            n764 = Array Size(array=w1299) -> (size(s)=w1298:i32)
            n765 = flat-sequence {
              tunnel: w1301 -> [_]
              tunnel: w1296 -> [w1329]
              tunnel: [w1329] -> w1297
              frame #0 {
                w1322 = T15."Disabled and Grayed Out" ("Disabled")
                n766 = property on="saveReq" class="Str"("Visible"=TRUE) -> ()  [unwired: 2 in, 2 out]
                n767 = local write "SampleID"("") -> ()
                n768 = property on="clearShots" class="Bool"("Disabled"=T15."Enabled") -> ()  [unwired: 2 in, 2 out]
                n769 = property on="addShot" class="Bool"("Disabled"=w1322) -> ()  [unwired: 2 in, 2 out]
                n770 = property on="undoLastShot" class="Bool"("Disabled"=w1322) -> ()  [unwired: 2 in, 2 out]
                n771 = property on="saveShots" class="Bool"("Disabled"=w1322) -> ()  [unwired: 2 in, 2 out]
                n772 = One Button Dialog(message="Data Saved. Enter new Sample ID.") -> ()  [unwired: 1 in, 1 out]
                n773 = property on="mainTabCntrl" class="TabCtl (strict)"("Value"=enum32{"Setup", "Measure", "History", "System"}."Setup" ("mainTabCntrl")) -> ()  [unwired: 2 in, 2 out]
                n774 = property on="SampleEntryTabCntrl" class="TabCtl (strict)"("Value"=enum32{"Environment", "Sample"}."Sample" ("SampleEntryTabCntrl")) -> ()  [unwired: 2 in, 2 out]
                n775 = property on="Sample SubTabCntrl" class="TabCtl (strict)"("Value"=T2."General Specification" ("Sample SubTabCntrl")) -> ()  [unwired: 2 in, 2 out]
              }
            }
            n776 = Increment(x=w1319) -> (x+1=w1313:i32)
            n777 = call <vilib>:"Open Config Data (compatibility).vi"("error in (no error)"=w1307, "configuration file path"=w1302) -> ("error out"=w1312:errorcluster, "refnum"=w1311:T36)  [unwired: 7 in, 1 out]
            n778 = Add(x=w1313, y=w1318) -> (x+y=w1314:i32)
            n779 = local read "LastSample"() -> (w1315:i32)
            n780 = for {
              N: w1298 -> [_]
              shift-right: [w1320] -> w1296
              shift-left: w1299 -> [w1321]
              n781 = Delete From Array(array=w1321) -> (array with subset deleted=w1320:T7[])  [unwired: 2 in, 1 out]
            }
            n782 = local write "LastShot"(w1314) -> ()
            n783 = call-poly <vilib>:"Write Key.vi"("section"=w1308, "error in (no error)"=w1312, "value"=w1314, "key"="Last Shot Saved ", "refnum"=w1311) -> ("error out"=w1310:errorcluster, "refnum out"=w1309:T36)  [unwired: 5 out]
            n784 = Increment(x=w1315) -> (x+1=w1303:i32)
            n785 = local write "LastSample"(w1303) -> ()
            n786 = call-poly <vilib>:"Write Key.vi"("section"=w1308, "error in (no error)"=w1310, "value"=w1303, "key"="Last Panel Saved ", "refnum"=w1309) -> ("error out"=w1300:errorcluster)  [unwired: 6 out]
            n787 = To Double Precision Float(number=w1303) -> (double precision float=w1306:dbl)
            n788 = call <vilib>:"Close Config Data.vi"("error in (no error)"=w1300, "refnum"=w1309) -> ("error out"=w1301:errorcluster)  [unwired: 1 in, 8 out]
            n789 = property on="Record #" class="DigNum (strict)"("Maximum"=w1306) -> ()  [unwired: 2 in, 2 out]
            n790 = property on="SHOTS" class="Arr (strict)"("Val(Sgnl)"=w1296) -> ()  [unwired: 2 in, 2 out]
          }
          frame Error {
            n791 = One Button Dialog(message="Error saving Data. ") -> ()  [unwired: 2 out]
            n792 = call <vilib>:"General Error Handler.vi"("error in (no error)"=w1334) -> ("error out"=w1332:errorcluster)  [unwired: 2 in, 12 out]
          }
        }
      }
      frame 5 {
        # "Shot Order"
        # "This section accepts new data to the shot table."
        n793 = property on="undoLastShot" class="Bool"(error in=w1345, "Disabled"=u8 0) -> (error out=w1344:errorcluster)  [unwired: 1 in, 1 out]
        n794 = local read "residual/speed"() -> (w1370:sgl)
        n795 = local read "Impact/speed"() -> (w1374:sgl)
        n796 = Array Size(array=w1350) -> (size(s)=w1355:i32)
        n797 = Increment(x=w1355) -> (x+1=w1375:i32)
        n798 = case shown="\"grains\"" "loadingUnits" {
          tunnel: [w1382 w1383] -> w1340
          tunnel: "Powder Loading" -> [w1382 w1384]
          frame "grams", Default {
            # "Always save in grams."
          }
          frame "grains" {
            # "Always save in grams."
            n799 = Multiply(x=w1384, y=sgl 0.06479891) -> (x*y=w1383:sgl)
          }
        }
        n800 = local read "Current/residual/speed"() -> (w1358:sgl)
        n801 = local read "CorrectedVelScrnSet2"() -> (w1379:sgl)
        n802 = local read "MeasVelScrnSet2"() -> (w1376:sgl)
        n803 = local read "CorrectedVelScrnSet1"() -> (w1359:sgl)
        n804 = local read "MeasVelScrnSet1"() -> (w1377:sgl)
        n805 = local read "Current/avg/speed"() -> (w1381:sgl)
        n806 = local read "Corrected Residual"() -> (w1357:sgl)
        n807 = local read "BACKFACE DEPTH"() -> (w1361:sgl)
        n808 = local read "Redundant/speed"() -> (w1378:sgl)
        n809 = local read "conversion factor"() -> (w1368:sgl)
        n810 = local read "Projectile Mass"() -> (w1347:sgl)
        n811 = local read "SHOT STATUS"() -> (w1354:u16)
        n812 = local read "Avg/speed"() -> (w1380:sgl)
        n813 = Multiply(x=w1374, y=w1368) -> (x*y=w1366:sgl)
        n814 = Multiply(x=w1368, y=w1370) -> (x*y=w1367:sgl)
        n815 = Multiply(x=w1366, y=w1366) -> (x*y=w1362:sgl)
        n816 = Multiply(x=w1367, y=w1367) -> (x*y=w1363:sgl)
        n817 = Subtract(x=w1362, y=w1363) -> (x-y=w1364:sgl)
        n818 = Format Date/Time String(time format string (%c)="%x   %H:%M:%S") -> (date/time string=w1371:string)  [unwired: 2 out]
        "SUBMIT DATE/TIME" <- w1371
        n819 = Compound Arithmetic op=MULTIPLY(w1347, w1364, sgl 0.0005 ("Input")) -> (w1369:sgl)
        n820 = Index Array(array=w1350) -> (element=w1353:T7)  [unwired: 1 in]
        n821 = Bundle By Name(cluster=w1353, "TIME / DATE"=w1371, "shot order"=w1375, "IMPACT VELOCITY"=w1374, "RESIDUAL  VELOCITY"=w1370, "Shot Description"="Shot Description", "Powder Loading"=w1340, "Barrel Temperature"="Barrel Temp", "SHOT STATUS"=w1354, "BackFace\nDepth"=w1361, "Shot Angle"="Shot Angle", "Uncorrected Impact"=w1377, "Corrected Impact"=w1359, "Uncorrected Residual"=w1358, "Corrected residual"=w1357, "Projectile Mass"=w1347, "Energy Loss (J)"=w1369, "UncorrectedRed_PB"=w1376, "Redundant_Velocity"=w1378, "CorrectedRed_PB"=w1379, "UncorrectedAvgVel_PB"=w1381, "avgVel_PB"=w1380, "Frag Rod"="Frag Rod", "V50userExcl"=FALSE) -> (w1356:T7)
        n822 = Build Array (concatenate)(w1350, w1356) -> (w1346:T7[])
        n823 = stacked-sequence {
          tunnel: w1346 -> [w1389]
          tunnel: [w1389] -> w1337
          tunnel: w1344 -> [w1388]
          tunnel: [w1387] -> w1343
          frame #0 {
            n824 = property on="shotsTabCntrl" class="TabCtl (strict)"(error in=w1388, "Value"=T5."Shots Table" ("shotsTabCntrl")) -> (error out=w1387:errorcluster)  [unwired: 1 in, 1 out]
            n825 = local write "backdepth"(sgl 0.0 ("BACKFACE DEPTH")) -> ()
          }
        }
      }
      frame 6 {
        # "This section will clear the shot table and re-enable the \"ADD SHOT\" button to get ready for a new test panel."
        n826 = Two Button Dialog(message="Shot table cleared even if not saved. Are you sure?", 1:"NO" ("F button name (\"Cancel\")"), 2:"YES" ("T button name (\"OK\")")) -> (T button?=w1394:bool)
        n827 = case shown="True" w1394 {
          tunnel: [w1400 T7[] [] ("SHOTS")] -> w1399
          tunnel: w1395 -> [w1400 _]
          frame False {
          }
          frame True {
            w1401 = T15."Disabled and Grayed Out" ("Disabled")
            n828 = invoke on="Table of Shots" class="Tbl (strict)" method="Reinit To Default"() -> ()  [unwired: 3 in, 3 out]
            n829 = property on="addShot" class="Bool"("Disabled"=T15."Enabled") -> ()  [unwired: 2 in, 2 out]
            n830 = invoke on="SHOTS" class="Arr (strict)" method="Reinit To Default"() -> ()  [unwired: 3 in, 3 out]
            n831 = property on="saveReq" class="Str"("Visible"=TRUE) -> ()  [unwired: 2 in, 2 out]
            n832 = property on="clearShots" class="Bool"("Disabled"=w1401) -> ()  [unwired: 2 in, 2 out]
            n833 = property on="undoLastShot" class="Bool"("Disabled"=w1401) -> ()  [unwired: 2 in, 2 out]
            n834 = property on="saveShots" class="Bool"("Disabled"=w1401) -> ()  [unwired: 2 in, 2 out]
          }
        }
      }
      frame 7 {
        n835 = property on="SHOTS" class="Arr (strict)"(error in=w1407) -> (error out=w1406:errorcluster, "Index Values"=w1411:u32[])  [unwired: 1 in, 1 out]
        n836 = Array Size(array=w1418) -> (size(s)=w1414:i32)
        n837 = Index Array "Index Array"(array=w1411) -> (element=w1416:u32)  [unwired: 1 in]
        n838 = To Unsigned Long Integer(number=w1414) -> (unsigned 32bit integer=w1410:u32)
        n839 = Increment(x=w1416) -> (x+1=w1415:u32)
        n840 = Quotient & Remainder(x=w1415, y=w1410) -> (x-y*floor(x/y)=w1413:u32)  [unwired: 1 out]
        n841 = Replace Array Subset "Replace Array Subset"(array=w1411, new element=w1413) -> (w1412:u32[])  [unwired: 1 in]
        n842 = property on="SHOTS" class="Arr (strict)"(error in=w1406, "Index Values"=w1412) -> (error out=w1405:errorcluster, "Value"=w1417:T7[])  [unwired: 1 in, 1 out]
      }
      frame 8 {
        # "This section undoes new shot data OR deletes the currently accessed previous shot"
        n843 = local read "deleteShot"() -> (w1425:bool)
        n844 = case shown="True" w1425 {
          tunnel: w1424 -> [w1428 w1441]
          tunnel: [w1429 w1442] -> w1423
          frame False {
            n845 = Array Size(array=w1428) -> (size(s)=w1426:i32)
            n846 = while {
              tunnel: [w1432] -> w1427
              tunnel: w1426 -> [w1434]
              tunnel: w1428 -> [w1436] mode=indexing
              i -> [w1432]
              stop <- w1435 stop-if-true
              n847 = Unbundle By Name(w1436) -> ("shot order"=w1433:i32)
              n848 = Equal?(x=w1433, y=w1434) -> (x = y?=w1435:bool)
            }
            n849 = Delete From Array "Delete From Array"(array=w1428, index=w1427) -> (array with subset deleted=w1429:T7[])  [unwired: 1 in, 1 out]
            n850 = local write "SUBMIT DATE/TIME"("" ("Empty String Constant")) -> ()
            n851 = property on="undoLastShot" class="Bool"("Disabled"=u8 2) -> ()  [unwired: 2 in, 2 out]
          }
          frame True {
            n852 = property on="SHOTS" class="Arr (strict)"() -> ("Index Values"=w1450:u32[])  [unwired: 2 in, 2 out]
            n853 = local write "deleteShot"(FALSE) -> ()
            n854 = Index Array(array=w1450, index=0 ("Index")) -> (element=w1440:u32)
            n855 = To Long Integer(number=w1440) -> (32bit integer=w1437:i32)
            n856 = Index Array(array=w1441, index=w1437) -> (element=w1439:T7)
            n857 = Unbundle By Name(w1439) -> ("shot order"=w1438:i32)
            n858 = Format Into String(format string="The currently displayed Shot, #%d", w1438) -> (resulting string=w1447:string)  [unwired: 2 in, 1 out]
            n859 = Concatenate Strings(w1447, ", will be deleted.  IT CANNOT RECOVERED!  Do you want to DELETE the shot?" ("message")) -> (w1446:string)
            n860 = Two Button Dialog(message=w1446, 1:"NO I do NOT want to delete.  Cancel Request" ("F button name (\"Cancel\")"), 2:"YES I want to delete the shot" ("T button name (\"OK\")")) -> (T button?=w1453:bool)
            n861 = case shown="True" w1453 {
              tunnel: w1441 -> [w1466 w1469]
              tunnel: [w1466 w1471] -> w1444
              tunnel: w1437 -> [_ w1468]
              tunnel: [10000 ("shot order") w1470] -> w1443
              frame False {
              }
              frame True {
                n862 = Index Array(array=w1469, index=w1468) -> (element=w1467:T7)
                n863 = Unbundle By Name(w1467) -> ("shot order"=w1470:i32)
                n864 = Delete From Array(array=w1469, index=w1468) -> (array with subset deleted=w1471:T7[])  [unwired: 1 in, 1 out]
              }
            }
            n865 = for {
              tunnel: [w1460] -> w1442 mode=indexing
              tunnel: w1444 -> [w1455] mode=indexing
              tunnel: w1443 -> [w1459]
              n866 = Unbundle By Name(w1455) -> ("shot order"=w1457:i32)
              n867 = Decrement(x=w1457) -> (x-1=w1456:i32)
              n868 = Greater?(x=w1457, y=w1459) -> (0:w1458:bool)
              n869 = case shown="True" w1458 {
                tunnel: w1456 -> [_ w1463]
                tunnel: w1455 -> [w1461 w1464]
                tunnel: [w1461 w1462] -> w1460
                frame False {
                }
                frame True {
                  n870 = Bundle By Name(cluster=w1464, "shot order"=w1463) -> (w1462:T7)
                }
              }
            }
          }
        }
        n871 = property on="SHOTS" class="Arr (strict)"(error in=w1419, "Val(Sgnl)"=w1423) -> (error out=w1420:errorcluster)  [unwired: 1 in, 1 out]
      }
      frame 9 {
        n872 = local write "SUBMIT DATE/TIME"("" ("Empty String Constant")) -> ()
        n873 = Concatenate Strings("L|", "6|") -> (w1478:string)
        n874 = case shown="\"Simulated\", Default" "MeasSrc" {
          tunnel: w1478 -> [_ _ w1494]
          tunnel: w1473 -> [w1484 w1489 w1493]
          tunnel: [w1482 w1489 w1490] -> w1472
          frame "Simulated", Default {
            n875 = flat-sequence {
              tunnel: w1484 -> [w1485]
              tunnel: [w1485] -> w1483
              tunnel: [w1487] -> w1482
              tunnel: w1483 -> [w1487]
              frame #0 {
                n876 = local write "readyClock"(FALSE ("RANGE RESET")) -> ()
              }
              frame #1 {
                n877 = Wait (ms)(milliseconds to wait=u32 100) -> ()  [unwired: 1 out]
              }
            }
          }
          frame "Radar" {
          }
          frame "Screens" {
            w1500 = u32 22 items=["NI-DAQ version", "device name", "base address", "data transfer mode for analog input", "data transfer mode for analog output group 1", "data transfer mode for analog output group 2", "data transfer mode for GPCTR 0", "data transfer mode for GPCTR 1", "data transfer mode for digital I/O group 1", "data transfer mode for digital I/O group 2", "device type code", "DMA A level", "DMA B level", "DMA C level", "interrupt A level", "interrupt B level", "reserved", "lpt device mode", "DAQCard-700 counter 1 source", "interrupt generation mode", "device state during suspend mode", "computer name", "serial number", "counter type", "Scarab A Memory Size", "Scarab B Memory Size"] ("information type")
            w1499 = u32 1  # device
            n878 = Concatenate Strings(w1494, "2|") -> (w1495:string)
            n879 = call <vilib>:"Get DAQ Device Information.vi"("error in (no error)"=w1493, "information type"=w1500, "task ID or device"=w1499) -> ("error out"=w1492:errorcluster, "information string"=w1498:string)  [unwired: 7 out]
            n880 = disable-structure "Diagram Disable Structure" shown="Enabled" {
              disable-tunnel: w1495 -> [w1505 _]
              disable-tunnel: w1492 -> [w1502 w1507]
              disable-tunnel: [w1501 w1507] -> w1491
              frame Disabled {
                n881 = Current VI's Path() -> (path=w1506:path)
                n882 = call "Where Am I (SubVI).vi"("TL Calling Location"=w1505, "Call VI path"=w1506) -> ("I'm here"=w1504:string)
                n883 = call "Error Check (SubVI).vi"("calling VI"=w1504, "tag #"=0, "error IN"=w1502) -> ("error OUT"=w1501:errorcluster)  [unwired: 2 in]
              }
              frame Enabled {
                # "Debug code is disabled"
              }
            }
            n884 = case shown="Error" w1491 {
              selector: w1491 -> [w1508 _]
              tunnel: w1498 -> [w1518 _]
              tunnel: [w1518 "DEVICE NOT READY!" ("information string")] -> w1497
              tunnel: [w1509 errorcluster {"status"=FALSE, "code"=0, "source"=""} ("error out")] -> w1490
              frame No Error {
                # "assign task IDs to counters"
                n885 = call "Config Counter to Measure Two Edge Separation.vi"("error IN"=w1508, "Counter"="Impact Timer", "device"="DAQ Card") -> ("error out"=w1520:errorcluster, "task ID out"=w1514:u32)  [unwired: 1 in]
                "impact/ID" <- w1514
                n886 = local write "readyClock"(FALSE ("RANGE RESET")) -> ()
                n887 = call "Config Counter to Measure Two Edge Separation.vi"("error IN"=w1520, "Counter"="Residual  Timer", "device"="DAQ Card") -> ("error out"=w1522:errorcluster, "task ID out"=w1512:u32)  [unwired: 1 in]
                "residual/ID" <- w1512
                n888 = call "Config Counter to Measure Two Edge Separation.vi"("error IN"=w1522, "Counter"="Redundant Timer", "device"="DAQ Card") -> ("error out"=w1521:errorcluster, "task ID out"=w1513:u32)  [unwired: 1 in]
                "Red/ID" <- w1513
                n889 = Bundle("task ID out"=w1514, "task ID out"=w1513, "task ID out"=w1512) -> (w1510:T37)  [unwired: 1 out]
                n890 = call <vilib>:"Simple Error Handler.vi"("error in (no error)"=w1521) -> ("error out"=w1509:errorcluster)  [unwired: 1 in, 7 out]
                n891 = global write "BIMS_Collector Globals.vi" "Screens"(w1510) -> ()
              }
              frame Error {
                n892 = One Button Dialog(message="Error initializing Timer board.  Switching to simulation") -> ()  [unwired: 2 out]
                n893 = local write "MeasSrc"(DataSource."Simulated" ("MeasSrc")) -> ()
              }
            }
            "Device S/N" <- w1497
          }
        }
      }
      frame 9 {
        n894 = local write "processShots"(FALSE ("ProcessShots")) -> ()
        n895 = local read "Drag Corrected"() -> (w1532:bool)
        n896 = stacked-sequence {
          seq-local: [_ w1590 _ _] -> [_ _ w1619 w1669]
          seq-local: [w1554 _ _ _] -> [_ w1586 _ _]
          seq-local: [w1552 _ _ _] -> [_ w1587 _ _]
          seq-local: [w1553 _ _ _] -> [_ w1588 _ _]
          tunnel: [_ _ _ w1662] -> w1533
          tunnel: w1532 -> [w1556 w1589 _ _]
          tunnel: w1529 -> [_ w1585 _ _]
          tunnel: w1528 -> [w1551 _ _ _]
          tunnel: [w1551 _ _ _] -> w1527
          frame #0 {
            n897 = disable-structure "Diagram Disable Structure" shown="Enabled" {
              disable-tunnel: [w1573 w1580] -> w1561
              frame Disabled {
                n898 = local read "factor array"() -> (w1575:sgl[])
                n899 = local read "Threat"() -> (w1572:u16)
                n900 = To Long Integer(number=w1572) -> (32bit integer=w1574:i32)
                n901 = Index Array(array=w1575, index=w1574) -> (element=w1573:sgl)
              }
              frame Enabled {
                n902 = local read "threatDetails"() -> (w1579:T1)
                n903 = Unbundle By Name(w1579) -> ("dragCorrection"=w1577:string)
                n904 = Not Equal?(x=w1577, y="") -> (x != y?=w1578:bool)
                n905 = case shown="True" w1578 {
                  tunnel: [sgl 1.0 ("default value 1") w1583] -> w1580
                  tunnel: w1577 -> [_ w1582]
                  frame False {
                  }
                  frame True {
                    n906 = Scan From String(input string=w1582, default 1=sgl 0.0 ("default value 1")) -> (output 1=w1583:sgl)  [unwired: 3 in, 3 out]
                  }
                }
              }
            }
            "correction coefficient" <- w1561
            n907 = local read "Current/avg/speed"() -> (w1557:sgl)
            n908 = local read "mid_to_targ_dist"() -> (w1558:sgl)
            n909 = local read "lengthUnits"() -> (w1555:string)
            n910 = call "Compute Strike Velocity.vi"("drag coefficient"=w1561, "decay distance"=w1558, "raw velocity"=w1557, "distance units"=w1555) -> ("correction factor"=w1554:sgl, "strike velocity"=w1559:sgl)  [unwired: 1 out]
            "DC_ factor" <- w1554
            "Corrected Average" <- w1559
            n911 = call "Velocity Correction.vi"("raw impact"="MeasVelScrnSet1", "distance units"=w1555, "raw redundant"="MeasVelScrnSet2", "raw residual"="Current/residual/speed", "screen set midpt to target"="Set#1_to_Target", "residual screen to target"="Residual/Target Dist", "correction coefficient"=w1561) -> ("corrected impact"=w1566:sgl, "corrected redundant"=w1562:sgl, "corrected residual"=w1564:sgl, "impact factor"=w1552:sgl, "conversion factor"=→"conversion factor":sgl, "residual factor"=w1553:sgl)  [unwired: 3 out]
            "Residual factor" <- w1553
            "Impact factor" <- w1552
            "CorrectedVelScrnSet1" <- w1566
            "Corrected Residual" <- w1564
            "CorrectedVelScrnSet2" <- w1562
            n912 = Select(t=w1562, s=w1556, f="MeasVelScrnSet2") -> (s? t:f=→"Redundant/speed":sgl)
            n913 = Select(t=w1559, s=w1556, f=w1557) -> (s? t:f=→"Avg/speed":sgl)
            n914 = Select(t=w1566, s=w1556, f="MeasVelScrnSet1") -> (s? t:f=→"Impact/speed":sgl)
            n915 = Select(t=w1564, s=w1556, f="Current/residual/speed") -> (s? t:f=→"residual/speed":sgl)
            n916 = Add(x="MeasVelScrnSet2", y="MeasVelScrnSet1") -> (x+y=w1538:sgl)
            n917 = Subtract(x="MeasVelScrnSet2", y="MeasVelScrnSet1") -> (x-y=w1537:sgl)
            n918 = Divide(x=w1538, y=sgl 200.0) -> (x/y=w1539:sgl)
            n919 = Divide(x=w1537, y=w1539) -> (x/y=w1543:sgl)
            "%_Difference" <- w1543
            n920 = Absolute Value(x=w1543) -> (abs(x)=w1545:sgl)
            n921 = Less?(x=w1545, y="percent warning") -> (x < y?=w1550:bool)
            n922 = Select(t=u32 65343, s=w1550, f=u32 15668992) -> (s? t:f=w1546:u32)
            n923 = Select(t=u32 0, s=w1550, f=u32 16777226) -> (s? t:f=w1549:u32)
            n924 = property on="%_Difference" class="DigNum (strict)"("Numeric Text.Text Colors:BG Color"=w1546, "NumText.TextColor"=w1549) -> ()  [unwired: 2 in, 2 out]
          }
          frame #1 {
            # "<-- DC_factor (for Average of impact and redundant)"
            # "IF drag corrected THEN apply factors"
            # "Residual factor"
            # "Impact factor\n(also applies to\nredundant velocity)"
            n925 = for {
              tunnel: w1585 -> [w1598] mode=indexing
              tunnel: w1588 -> [w1607]
              tunnel: w1587 -> [w1602]
              tunnel: w1589 -> [w1596]
              tunnel: [w1609] -> w1590 mode=indexing
              tunnel: w1586 -> [w1591]
              n926 = Unbundle By Name(w1598) -> ("UncorrectedAvgVel_PB"=w1597:sgl)
              n927 = Unbundle By Name(w1598) -> ("Uncorrected Impact"=w1601:sgl)
              n928 = Unbundle By Name(w1598) -> ("Uncorrected Residual"=w1606:sgl)
              n929 = Unbundle By Name(w1598) -> ("UncorrectedRed_PB"=w1604:sgl)
              n930 = Multiply(x=w1591, y=w1597) -> (x*y=w1594:sgl)
              n931 = Multiply(x=w1602, y=w1604) -> (x*y=w1603:sgl)
              n932 = Multiply(x=w1602, y=w1601) -> (x*y=w1592:sgl)
              n933 = Multiply(x=w1607, y=w1606) -> (x*y=w1599:sgl)
              n934 = Select(t=w1594, s=w1596, f=w1597) -> (s? t:f=w1595:sgl)
              n935 = Select(t=w1603, s=w1596, f=w1604) -> (s? t:f=w1605:sgl)
              n936 = Select(t=w1599, s=w1596, f=w1606) -> (s? t:f=w1608:sgl)
              n937 = Select(t=w1592, s=w1596, f=w1601) -> (s? t:f=w1600:sgl)
              n938 = Subtract(x=w1595, y=w1594) -> (x-y=w1593:sgl)
              n939 = Bundle By Name(cluster=w1598, "velLoss_PB"=w1593, "strikeVel_PB"=w1594, "avgVel_PB"=w1595, "CorrectedRed_PB"=w1603, "Redundant_Velocity"=w1605, "Corrected Impact"=w1592, "IMPACT VELOCITY"=w1600, "Corrected residual"=w1599, "RESIDUAL  VELOCITY"=w1608) -> (w1609:T7)
            }
          }
          frame #2 {
            w1620 = sgl[] [] ("Partial")
            # "This section calculates the V50"
            n940 = for {
              shift-right: [w1644] -> w1622
              shift-left: w1620 -> [w1645]
              shift-right: [w1642] -> w1621
              shift-left: w1620 -> [w1643]
              tunnel: w1619 -> [w1636] mode=indexing
              n941 = Unbundle By Name(w1636) -> ("SHOT STATUS"=w1641:u16)
              n942 = Unbundle By Name(w1636) -> ("V50userExcl"=w1635:bool)
              n943 = Unbundle By Name(w1636) -> ("IMPACT VELOCITY"=w1640:sgl)
              n944 = Unbundle By Name(w1636) -> ("strikeVel_PB"=w1639:sgl)
              n945 = Select(t=w1639, s="ScreenSetAvgg", f=w1640) -> (s? t:f=w1638:sgl)
              n946 = case shown="False" w1635 {
                tunnel: w1645 -> [w1651 w1661]
                tunnel: [w1650 w1661] -> w1644
                tunnel: w1643 -> [w1649 w1660]
                tunnel: [w1648 w1660] -> w1642
                tunnel: w1641 -> [w1647 _]
                tunnel: w1638 -> [w1646 _]
                frame False {
                  n947 = case shown="1" w1647 {
                    tunnel: w1646 -> [w1652 w1656]
                    tunnel: [w1655 w1657] -> w1650
                    tunnel: w1651 -> [w1654 w1657]
                    tunnel: w1649 -> [w1653 w1659]
                    tunnel: [w1653 w1658] -> w1648
                    frame 0, Default {
                      n948 = Build Array (concatenate)(w1654, w1652) -> (w1655:sgl[])
                    }
                    frame 1 {
                      n949 = Build Array (concatenate)(w1659, w1656) -> (w1658:sgl[])
                    }
                  }
                }
                frame True {
                }
              }
            }
            n950 = Sort 1D Array(array=w1622) -> (sorted array=w1634:sgl[])
            n951 = Sort 1D Array(array=w1621) -> (sorted array=w1627:sgl[])
            "Complete" <- w1627
            n952 = Reverse 1D Array(array=w1634) -> (reversed array=w1625:sgl[])
            "Partial" <- w1625
            n953 = Array Size(array=w1627) -> (size(s)=→"#_completes":i32)
            n954 = Array Size(array=w1625) -> (size(s)=→"#_partials":i32)
            n955 = Array Max & Min(array=w1625) -> (max value=w1631:sgl)  [unwired: 3 out]
            n956 = Array Max & Min(array=w1627) -> (min value=w1629:sgl)  [unwired: 3 out]
            n957 = call "Compute V50.vi"("Partial"=w1625, "Maximum Deviation"="maxDev", "Complete"=w1627) -> ("Pairs"=→"Pairs":i16, "zmr"=w1610:sgl, "V50"=→"computed_V50":sgl)  [unwired: 2 out]
            "Z.M.R." <- w1610
            n958 = To Long Integer(number=w1631) -> (32bit integer=→"highPartial":i32)
            n959 = To Long Integer(number=w1629) -> (32bit integer=→"lowComplete":i32)
            n960 = Absolute Value(x=w1610) -> (abs(x)=→"zmr 2":sgl)
            n961 = Less Than 0?(x=w1610) -> (x < 0?=w1613:bool)
            n962 = Select(t="Low C minus High P", s=w1613, f="ZMR") -> (s? t:f=w1616:string)
            n963 = Select(t=u32 65336, s=w1613, f=u32 16755266) -> (s? t:f=w1617:u32)
            n964 = property on="zmr 2" class="DigNum (strict)"("Caption.Text"=w1616, "Numeric Text.Text Colors:BG Color"=w1617) -> ()  [unwired: 2 in, 2 out]
          }
          frame #3 {
            n965 = local read "Pairs"() -> (w1674:i16)
            n966 = Sort 1D Array(array=w1669) -> (sorted array=w1672:T7[])
            n967 = for {
              tunnel: w1672 -> [w1718] mode=indexing
              tunnel: w1674 -> [w1728]
              shift-right: [w1727] -> _
              shift-left: i16 0 -> [w1726]
              tunnel: [w1720] -> w1670 mode=indexing
              # "this section marks the lowest completes that are used in V50"
              n968 = Unbundle By Name(w1718) -> ("SHOT STATUS"=w1724:u16, "Projectile Mass"=w1722:sgl, "avgVel_PB"=w1721:sgl, "RESIDUAL  VELOCITY"=w1723:sgl)
              n969 = Unbundle By Name(w1718) -> ("V50userExcl"=w1719:bool)
              n970 = local read "conversion factor"() -> (w1730:sgl)
              n971 = case shown="True" w1719 {
                tunnel: w1728 -> [w1741 _]
                tunnel: [w1740 w1750] -> w1727
                tunnel: w1726 -> [w1739 w1750]
                tunnel: [w1738 FALSE] -> w1725
                tunnel: w1724 -> [w1737 _]
                frame False {
                  n972 = case shown="1" w1737 {
                    tunnel: w1741 -> [_ w1748]
                    tunnel: [FALSE w1747] -> w1738
                    tunnel: [w1743 w1746] -> w1740
                    tunnel: w1739 -> [w1743 w1744]
                    frame 0, Default {
                    }
                    frame 1 {
                      n973 = Less?(x=w1744, y=w1748) -> (x < y?=w1747:bool)
                      n974 = Add(x=w1744, y=i16 1 ("t")) -> (x+y=w1746:i16)
                    }
                  }
                }
                frame True {
                }
              }
              n975 = Multiply(x=w1730, y=w1723) -> (x*y=w1731:sgl)
              n976 = Multiply(x=w1721, y=w1730) -> (x*y=w1732:sgl)
              n977 = Multiply(x=w1732, y=w1732) -> (x*y=w1736:sgl)
              n978 = Multiply(x=w1731, y=w1731) -> (x*y=w1735:sgl)
              n979 = Subtract(x=w1736, y=w1735) -> (x-y=w1734:sgl)
              n980 = Compound Arithmetic op=MULTIPLY(w1722, w1734, sgl 0.0005 ("Input")) -> (w1729:sgl)
              n981 = Bundle By Name(cluster=w1718, "usedv50"=w1725, "Energy Loss (J)"=w1729) -> (w1720:T7)
            }
            n982 = Reverse 1D Array(array=w1670) -> (reversed array=w1671:T7[])
            n983 = for {
              tunnel: w1671 -> [w1694] mode=indexing
              tunnel: w1674 -> [w1701]
              shift-right: [w1699] -> _
              shift-left: i16 0 -> [w1700]
              tunnel: [w1697] -> w1662 mode=indexing
              # "chooses highest partials used in v50"
              n984 = Unbundle By Name(w1694) -> ("SHOT STATUS"=w1702:u16, "usedv50"=w1696:bool)
              n985 = Unbundle By Name(w1694) -> ("V50userExcl"=w1695:bool)
              n986 = case shown="True" w1695 {
                tunnel: w1702 -> [w1708 _]
                tunnel: w1701 -> [w1707 _]
                tunnel: w1700 -> [w1706 w1717]
                tunnel: [w1705 w1717] -> w1699
                tunnel: [w1704 FALSE ("usedv50")] -> w1698
                tunnel: w1696 -> [w1703 _]
                frame False {
                  n987 = case shown="1" w1708 {
                    tunnel: w1707 -> [w1712 _]
                    tunnel: [w1711 w1715] -> w1704
                    tunnel: w1706 -> [w1709 w1714]
                    tunnel: [w1710 w1714] -> w1705
                    tunnel: w1703 -> [_ w1715]
                    frame 0, Default {
                      n988 = Less?(x=w1709, y=w1712) -> (x < y?=w1711:bool)
                      n989 = Add(x=w1709, y=i16 1) -> (x+y=w1710:i16)
                    }
                    frame 1 {
                    }
                  }
                }
                frame True {
                }
              }
              n990 = Bundle By Name(cluster=w1694, "usedv50"=w1698) -> (w1697:T7)
            }
            n991 = for {
              shift-right: [w1680] -> w1663
              shift-left: sgl[] [] ("Partial") -> [w1677]
              tunnel: w1662 -> [w1679] mode=indexing
              n992 = local read "ScreenSetAvgg"() -> (w1684:bool)
              n993 = Unbundle By Name(w1679) -> ("V50userExcl"=w1678:bool, "usedv50"=w1676:bool)
              n994 = Unbundle By Name(w1679) -> ("IMPACT VELOCITY"=w1682:sgl)
              n995 = Unbundle By Name(w1679) -> ("strikeVel_PB"=w1683:sgl)
              n996 = Select(t=w1683, s=w1684, f=w1682) -> (s? t:f=w1681:sgl)
              n997 = case shown="False" w1678 {
                tunnel: w1681 -> [w1685 _]
                tunnel: [w1686 w1693] -> w1680
                tunnel: w1677 -> [w1687 w1693]
                tunnel: w1676 -> [w1688 _]
                frame False {
                  n998 = case shown="True" w1688 {
                    tunnel: w1687 -> [w1689 w1692]
                    tunnel: [w1689 w1691] -> w1686
                    tunnel: w1685 -> [_ w1690]
                    frame False {
                    }
                    frame True {
                      n999 = Build Array (concatenate)(w1692, w1690) -> (w1691:sgl[])
                    }
                  }
                }
                frame True {
                }
              }
            }
            n1000 = Array Max & Min(array=w1663) -> (max value=w1668:sgl, min value=w1667:sgl)  [unwired: 2 out]
            n1001 = Subtract(x=w1668, y=w1667) -> (x-y=w1666:sgl)
            n1002 = property on="SHOTS" class="Arr (strict)"("Val(Sgnl)"=w1662) -> ()  [unwired: 2 in, 2 out]
            n1003 = To Long Integer(number=w1666) -> (32bit integer=→"rangeOfResults":i32)
          }
        }
      }
      frame 11 {
        n1004 = local read "SafetyInterlock"() -> (w1759:cluster{"ARMED":bool})
        n1005 = Unbundle By Name(w1759) -> ("ARMED"=w1758:bool)
        n1006 = Not(x="InterlockExists") -> (.not. x?=w1754:bool)
        n1007 = Or(x=w1758, y=w1754) -> (x .or. y?=w1755:bool)
        n1008 = case shown="True" w1755 {
          tunnel: [Collector_State."POLL" ("progState") w1768] -> w1757
          tunnel: [-1 ("index of element") w1767] -> w1756
          tunnel: "InterlockExists" -> [_ w1766]
          tunnel: [w1761 w1765] -> w1752
          tunnel: w1751 -> [w1761 w1764]
          frame False {
          }
          frame True {
            n1009 = stacked-sequence {
              tunnel: [_ Collector_State."PROCESS SHOTS" ("progState")] -> w1768
              tunnel: [_ -1] -> w1767
              tunnel: w1766 -> [w1771 _]
              tunnel: [w1769 _] -> w1765
              tunnel: w1764 -> [w1770 _]
              frame #0 {
                n1010 = local read "MeasSrc"() -> (w1773:T6)
                n1011 = case shown="\"Simulated\", Default" w1773 {
                  tunnel: [w1776 w1800 w1811] -> w1772
                  tunnel: w1771 -> [_ _ w1809]
                  tunnel: w1770 -> [w1774 w1799 w1807]
                  tunnel: [w1774 w1799 w1808] -> w1769
                  frame "Simulated", Default {
                    # "Simulated"
                    n1012 = local read "minV50"() -> (w1782:i32)
                    n1013 = local read "Powder Loading"() -> (w1798:sgl)
                    n1014 = To Single Precision Float(number=w1782) -> (single precision float=w1781:sgl)
                    n1015 = call "Get Shell Speed.vi"("loading"=w1798, "v50"=w1781) -> ("impact"=w1786:sgl, "residual"=w1793:sgl)  [unwired: 1 in, 2 out]
                    n1016 = Random Number (0-1)() -> (number: 0 to 1=w1791:dbl)
                    n1017 = To Single Precision Float(number=w1791) -> (single precision float=w1787:sgl)
                    n1018 = Multiply(x=w1787, y=sgl 0.002) -> (x*y=w1790:sgl)
                    n1019 = local read "SafetyInterlock"() -> (w1777:cluster{"ARMED":bool})
                    n1020 = Add(x=w1790, y=sgl 0.999) -> (x+y=w1788:sgl)
                    n1021 = Greater Than 0?(x=w1793) -> (x > 0?=w1795:bool)
                    n1022 = Multiply(x=w1786, y=w1788) -> (x*y=w1785:sgl)
                    n1023 = Bundle By Name(cluster=w1777, "ARMED"=FALSE) -> (w1778:cluster{"ARMED":bool})
                    n1024 = Add(x=w1786, y=w1785) -> (x+y=w1783:sgl)
                    n1025 = Select(t=u16 1, s=w1795, f=u16 0) -> (s? t:f=w1794:u16)
                    n1026 = local write "readyClock"(TRUE ("RANGE RESET")) -> ()
                    n1027 = local write "SafetyInterlock"(w1778) -> ()
                    n1028 = Divide(x=w1783, y=sgl 2.0 ("v50")) -> (x/y=w1776:sgl)
                    n1029 = local write "Current/residual/speed"(w1793) -> ()
                    n1030 = local write "SHOT STATUS"(w1794) -> ()
                    n1031 = local write "Current/sthotstatus"(w1794) -> ()
                    n1032 = local write "MeasVelScrnSet1"(w1786) -> ()
                    n1033 = local write "MeasVelScrnSet2"(w1785) -> ()
                    n1034 = Wait (ms)(milliseconds to wait=u32 500 ("number")) -> ()  [unwired: 1 out]
                  }
                  frame "Radar" {
                    # "Radar -- (future)"
                    n1035 = local read "MeasVelScrnSet1"() -> (w1802:sgl)
                    n1036 = local read "MeasVelScrnSet2"() -> (w1801:sgl)
                    n1037 = Add(x=w1802, y=w1801) -> (x+y=w1803:sgl)
                    n1038 = Divide(x=w1803, y=sgl 2.0) -> (x/y=w1800:sgl)
                  }
                  frame "Screens" {
                    # "This section checks to see if the counters have been fired.  If they have then the counter times are read"
                    n1039 = Concatenate Strings("-1|", "F0|") -> (w1812:string)
                    n1040 = case shown="True" w1809 {
                      tunnel: w1807 -> [w1819 w1820]
                      tunnel: [w1819 w1820] -> w1806
                      frame False {
                      }
                      frame True {
                      }
                    }
                    n1041 = global read "BIMS_Collector Globals.vi" "Screens"() -> (w1810)
                    n1042 = Unbundle By Name(w1810) -> ("ScrnSet1CntrID"=w1815)
                    n1043 = Concatenate Strings(w1812, "2|") -> (w1816:string)
                    n1044 = call "Check DAQ Status.vi"("errIN"=w1806, "TL Calling Location"=w1816, "Task ID"=w1815) -> ("error out"=w1818:errorcluster, "Armed?"=w1805:bool)  [unwired: 1 out]
                    n1045 = case shown="False" w1805 {
                      tunnel: w1818 -> [w1848 w1886]
                      tunnel: w1815 -> [w1831 _]
                      tunnel: w1816 -> [w1844 _]
                      tunnel: w1810 -> [w1834 _]
                      tunnel: [w1822 w1887] -> w1811
                      tunnel: [w1821 w1886] -> w1808
                      frame False {
                        n1046 = local read "Set#1 Separation"() -> (w1851:sgl)
                        n1047 = Concatenate Strings(w1844, "F|") -> (w1839:string)
                        n1048 = call "Read TIO Count.vi"("TL Calling Location"=w1839, "error In"=w1848, "task IN"=w1831) -> ("error out"=w1833:errorcluster, "time (secs)"=w1853:sgl)  [unwired: 1 in, 4 out]
                        n1049 = Divide(x=w1851, y=w1853) -> (x/y=w1827:sgl)
                        n1050 = call "Arm TIO Channel.vi"("error IN"=w1833, "task ID IN"=w1831) -> ("error out"=w1832:errorcluster)  [unwired: 1 in, 2 out]
                        n1051 = Unbundle By Name(w1834) -> ("ScrnSet2CntrID"=w1836)
                        n1052 = Concatenate Strings(w1839, "a|") -> (w1842:string)
                        n1053 = call "Check DAQ Status.vi"("errIN"=w1832, "TL Calling Location"=w1842, "Task ID"=w1836) -> ("error out"=w1847:errorcluster, "Armed?"=w1838:bool)  [unwired: 1 out]
                        n1054 = case shown="False" w1838 {
                          tunnel: [w1864 sgl 0.0] -> w1828
                          tunnel: w1847 -> [w1863 w1868]
                          tunnel: [w1858 w1868] -> w1849
                          tunnel: w1836 -> [w1857 _]
                          tunnel: w1839 -> [w1861 _]
                          frame False {
                            n1055 = local read "Set#2 Separation"() -> (w1865:sgl)
                            n1056 = Concatenate Strings(w1861, "Fa|") -> (w1860:string)
                            n1057 = call "Read TIO Count.vi"("TL Calling Location"=w1860, "error In"=w1863, "task IN"=w1857) -> ("error out"=w1859:errorcluster, "time (secs)"=w1866:sgl)  [unwired: 1 in, 4 out]
                            n1058 = Divide(x=w1865, y=w1866) -> (x/y=w1864:sgl)
                            n1059 = call "Arm TIO Channel.vi"("error IN"=w1859, "task ID IN"=w1857) -> ("error out"=w1858:errorcluster)  [unwired: 1 in, 2 out]
                          }
                          frame True {
                          }
                        }
                        n1060 = Unbundle By Name(w1834) -> ("residualCntrID"=w1835)
                        n1061 = Add(x=w1827, y=w1828) -> (x+y=w1829:sgl)
                        n1062 = Concatenate Strings(w1839, "b|") -> (w1840:string)
                        n1063 = call "Check DAQ Status.vi"("errIN"=w1849, "TL Calling Location"=w1840, "Task ID"=w1835) -> ("error out"=w1846:errorcluster, "Armed?"=w1837:bool)  [unwired: 1 out]
                        n1064 = Divide(x=w1829, y=sgl 2.0) -> (x/y=w1822:sgl)
                        n1065 = case shown="True" w1837 {
                          tunnel: w1846 -> [w1875 w1884]
                          tunnel: [w1880 w1885] -> w1852
                          tunnel: w1835 -> [w1870 _]
                          tunnel: [w1869 w1884] -> w1823
                          tunnel: [w1877 sgl 0.0] -> w1850
                          tunnel: w1839 -> [w1872 _]
                          frame False {
                            w1881 = u16 1 items=["Partial", "Complete"] ("SHOT STATUS")
                            w1882 = u16 0 items=["Partial", "Complete"] ("SHOT STATUS")
                            n1066 = local read "Residual/Separation"() -> (w1876:sgl)
                            n1067 = Concatenate Strings(w1872, "Fb|") -> (w1873:string)
                            n1068 = call "Read TIO Count.vi"("TL Calling Location"=w1873, "error In"=w1875, "task IN"=w1870) -> ("error out"=w1871:errorcluster, "timeout"=w1878:bool, "time (secs)"=w1879:sgl)  [unwired: 1 in, 3 out]
                            n1069 = Divide(x=w1876, y=w1879) -> (x/y=w1877:sgl)
                            n1070 = call "Arm TIO Channel.vi"("error IN"=w1871, "task ID IN"=w1870) -> ("error out"=w1869:errorcluster)  [unwired: 1 in, 2 out]
                            n1071 = Select(t=w1882, s=w1878, f=w1881) -> (s? t:f=w1880:u16)
                          }
                          frame True {
                            w1885 = u16 1 items=["Partial", "Complete"] ("SHOT STATUS")
                          }
                        }
                        n1072 = local write "Current/residual/speed"(w1850) -> ()
                        n1073 = local write "MeasVelScrnSet1"(w1827) -> ()
                        n1074 = local write "MeasVelScrnSet2"(w1828) -> ()
                        n1075 = local write "SHOT STATUS"(w1852) -> ()
                        n1076 = local write "Current/sthotstatus"(w1852) -> ()
                        n1077 = case shown="No Error" w1823 {
                          selector: w1823 -> [w1856 _]
                          frame No Error {
                            # "=false"
                            n1078 = Unbundle By Name(w1856) -> ("status"=w1855:bool)
                            n1079 = Not(x=w1855) -> (.not. x?=w1854:bool)
                            n1080 = local write "readyClock"(w1854) -> ()
                          }
                          frame Error {
                          }
                        }
                        n1081 = local read "SafetyInterlock"() -> (w1824:cluster{"ARMED":bool})
                        n1082 = Bundle By Name(cluster=w1824, "ARMED"=FALSE) -> (w1825:cluster{"ARMED":bool})
                        n1083 = local write "SafetyInterlock"(w1825) -> ()
                        n1084 = call <vilib>:"Simple Error Handler.vi"("error in (no error)"=w1823) -> ("error out"=w1821:errorcluster)  [unwired: 1 in, 7 out]
                      }
                      frame True {
                        # "Error -10600 occurrs in \"Read Count.vi\"\n\n  Possible reason(s): NI-DAQ LV: No setup operation has been performed for the specified resources. Or, some resources require a specific ordering of calls for proper setup.  \n\n  Solution: To avoid this error, you must call the Dig_Line_Config function to setup the direction for each digital line prior to calling the Dig_Grp_Config function."
                        n1085 = local read "MeasVelScrnSet1"() -> (w1889:sgl)
                        n1086 = local read "MeasVelScrnSet2"() -> (w1888:sgl)
                        n1087 = Add(x=w1889, y=w1888) -> (x+y=w1890:sgl)
                        n1088 = Divide(x=w1890, y=sgl 2.0) -> (x/y=w1887:sgl)
                      }
                    }
                  }
                }
                "Current/avg/speed" <- w1772
              }
              frame #1 {
              }
            }
          }
        }
      }
    }
    "SMErr" <- w13
  }
  n1089 = while "U/I Event Handler" {
    shift-right: [w1895] -> _
    shift-left: w7 -> [w1896]
    stop <- FALSE stop-if-true
    n1090 = event shown="[23] \"RefreshMetadata\": Value Change" {
      selector: _ -> [_ _ _ _ _ _ _ _ _ _ _ _ _ _ _ _ _ _ _ _ _ _ _ _ _ _]
      dyn-events: _ -> [_ _ _ _ _ _ _ _ _ _ _ _ _ _ _ _ _ _ _ _ _ _ _ _ _ _]
      timeout: 100 -> [_ _ _ _ _ _ _ _ _ _ _ _ _ _ _ _ _ _ _ _ _ _ _ _ _ _]
      tunnel: w1896 -> [w1900 _ w1917 w1927 w1936 w1946 w1983 w2009 w2016 w2042 w2081 w2124 w2163 w2166 w2203 w2240 w2244 w2254 w2282 w2289 w2315 w2334 w2337 w2365 w2397 _]
      tunnel: [w1900 w1904 w1917 w1924 w1935 w1945 w1982 w2008 w2014 w2051 w2080 w2121 w2163 w2166 w2203 w2240 w2243 w2250 w2282 w2286 w2312 w2334 w2337 w2367 w2397 w2405] -> w1895
      tunnel: [FALSE ("UpdateMetadata") "EXIT" "diagPageVisible" "runtimeMenusVisible" "ARM" "QueryLoad" FALSE ("UpdateMetadata") FALSE ("UpdateMetadata") FALSE ("UpdateMetadata") FALSE ("UpdateMetadata") FALSE ("UpdateMetadata") FALSE ("UpdateMetadata") FALSE ("UpdateMetadata") FALSE ("UpdateMetadata") FALSE ("UpdateMetadata") FALSE ("UpdateMetadata") FALSE ("UpdateMetadata") FALSE ("UpdateMetadata") "Drag Corrected" FALSE ("UpdateMetadata") "PublishNewRecords" FALSE ("UpdateMetadata") FALSE ("UpdateMetadata") "RefreshMetadata" FALSE ("UpdateMetadata") FALSE ("UpdateMetadata")] -> w1894
      event Timeout {
        n1091 = event-data() -> ()  [unwired: 2 out]
        n1092 = Get Date/Time In Seconds() -> (seconds since 1Jan1904=w1902:timestamp)
        n1093 = Format Date/Time String(seconds (now)=w1902) -> (date/time string=→"TimeNow":string)  [unwired: 2 out]
      }
      event "EXIT": Value Change {
        n1094 = event-data() -> ()  [unwired: 2 out]
        n1095 = property on="Property Node" class="Application"(error in=errorcluster {"status"=FALSE, "code"=0, "source"=""} ("error in (no error)")) -> (error out=w1904:errorcluster, "Application:Kind"=w1909:T38)  [unwired: 1 in, 1 out]
        n1096 = Two Button Dialog(message="Exit BIMS Collector?\nAll Unsaved data will be lost.", 1:"NO" ("F button name (\"Cancel\")"), 2:"YES" ("T button name (\"OK\")")) -> (T button?=w1910:bool)
        n1097 = case shown="\"Development System\"" w1909 {
          tunnel: w1910 -> [w1911 w1912 w1913]
          frame Default {
            n1098 = Stop(stop? (T)=w1911) -> ()
          }
          frame "Development System" {
            n1099 = Stop(stop? (T)=w1912) -> ()
          }
          frame "Run Time System" {
            n1100 = Quit LabVIEW(quit? (T)=w1913) -> ()
          }
        }
      }
      event "diagPageVisible": Value Change {
        # "Toggles display of \"Internal Use\" tab for diagnostics purposes"
        # "Key navigation ONLY: Cntrl-Shift-F11"
        n1101 = event-data() -> ("NewVal"=w1920:bool)  [unwired: 1 out]
        n1102 = property on="aboutTabCntrl" class="TabCtl (strict)"(error in=errorcluster {"status"=FALSE, "code"=0, "source"=""} ("error in (no error)")) -> (error out=w1919:errorcluster, "Pages"=w1923:refnum<vi>[])  [unwired: 1 in, 1 out]
        n1103 = Index Array(array=w1923, index=3) -> (element=w1921:refnum<vi>)
        n1104 = property on="Property Node" class="Page"(reference=w1921, error in=w1919, "PageVis"=w1920) -> (error out=w1918:errorcluster)  [unwired: 1 out]
        n1105 = property on="diagPageVisible" class="Bool (strict)"(error in=w1918, "Value"=w1920) -> (error out=w1915:errorcluster)  [unwired: 1 in, 1 out]
        n1106 = call <vilib>:"General Error Handler.vi"("error in (no error)"=w1915) -> ()  [unwired: 2 in, 13 out]
      }
      event "runtimeMenusVisible": Value Change {
        # "Key navigation ONLY: Cntrl-Shift-F10"
        n1107 = event-data() -> ("NewVal"=w1929:bool)  [unwired: 1 out]
        n1108 = control-ref of="This VI"() -> (w1928:refnum<vi>)
        n1109 = property class="VI"(reference=w1928, error in=w1927, "Front Panel.ShowMenuBar"=w1929) -> (reference out=w1926:refnum<vi>, error out=w1925:errorcluster)
        n1110 = Close Reference(reference=w1926, error in (no error)=w1925) -> (error out=w1924:errorcluster)
      }
      event "ARM": Value Change {
        # "This section will arm the system"
        n1111 = event-data() -> ()  [unwired: 2 out]
        n1112 = disable-structure shown="Disabled" {
          frame Disabled {
            "DIO" <- u32 21 ("DIO")
          }
          frame Enabled {
          }
        }
        n1113 = Bundle By Name(cluster=cluster{"ARMED":bool} {"ARMED"=FALSE} ("Safety_Interlock"), "ARMED"=TRUE) -> (→"SafetyInterlock":cluster{"ARMED":bool})
        n1114 = local write "SUBMIT DATE/TIME"("" ("Empty String Constant")) -> ()
        n1115 = local read "MeasSrc"() -> (w1937:T6)
        n1116 = case shown="\"Screens\"" w1937 {
          tunnel: w1936 -> [w1940 w1941 w1943]
          tunnel: [w1940 w1941 w1943] -> w1935
          frame "Simulated", Default {
          }
          frame "Radar" {
          }
          frame "Screens" {
            n1117 = local write "readyClock"(TRUE ("readyClock")) -> ()
          }
        }
      }
      event "QueryLoad": Value Change {
        w1951 = "%x" ("time format string (%c)")
        w1967 = "" ("replace string (\"\")")
        # "This section plots  Impact velocity vs. loadingdata"
        n1118 = event-data() -> ()  [unwired: 2 out]
        n1119 = Format Date/Time String(time format string (%c)=w1951, seconds (now)="lkupStartDate") -> (date/time string=w1950:string)  [unwired: 1 out]
        n1120 = Format Date/Time String(time format string (%c)=w1951, seconds (now)="lkupEndDate") -> (date/time string=w1949:string)  [unwired: 1 out]
        n1121 = call "Trim String.vi"("inStr"="Powder.freeTxt") -> ("outStr"=w1965:string)
        n1122 = call "Trim String.vi"("inStr"="Threat.freeTxt") -> ("outStr"=w1966:string)
        n1123 = invoke on="v50_table" class="Tbl" method="Reinit To Default"(error in=w1946) -> (error out=w1958:errorcluster)  [unwired: 2 in, 2 out]
        n1124 = invoke on="Vel.vs.Loading" class="WFGraph (strict)" method="Reinit To Default"(error in=w1958) -> (error out=w1953:errorcluster)  [unwired: 2 in, 2 out]
        n1125 = Format Into String(format string="SELECT TOP %d dbsrc.experiment.threat, dbsrc.shots.loading, dbsrc.shots.impact, dbsrc.experiment.powder, dbsrc.shots.date from dbsrc.shots, dbsrc.experiment where dbsrc.shots.expt = dbsrc.experiment.expt and dbsrc.shots.loading > 0 and dbsrc.shots.date between '%s' and '%s' and dbsrc.shots.impact between 10 and 5000 and dbsrc.experiment.powder like '%%%s%%' and dbsrc.experiment.threat like '%%%s%%' and experiment.threat<>'' order by dbsrc.experiment.threat, dbsrc.shots.loading, dbsrc.shots.impact;" ("Format String"), error in=w1953, "maxRecs", w1950, w1949, w1965, w1966) -> (resulting string=w1971:string, error out=w1956:errorcluster)  [unwired: 1 in]
        n1126 = Search and Replace String(input string=w1971, search string=" and experiment.powder like '%%'", replace string=w1967, error in=w1956) -> (result string=w1969:string, error out=w1957:errorcluster)  [unwired: 6 out]
        n1127 = Search and Replace String(input string=w1969, search string="and experiment.threat like '%%'", replace string=w1967, error in=w1957) -> (result string=w1960:string, error out=w1955:errorcluster)  [unwired: 6 out]
        n1128 = call "Fetch Data (SubVI).vi"("error IN"=w1955, "query string"=w1960) -> ("error OUT"=w1945:errorcluster, "recordset data"=w1961:string[][])  [unwired: 4 out]
        "v50_table" <- w1961
        n1129 = Fract/Exp String To Number(string=w1961) -> (number=w1975:dbl[][])  [unwired: 4 out]
        n1130 = Array Size(array=w1961) -> (size(s)=w1963:i32[])
        n1131 = Index Array(array=w1963) -> (element=→"ActualNumRecs":i32)  [unwired: 1 in]
        n1132 = Index Array(array=w1975, index (col)=2 ("Disabled Index (col)")) -> (element=w1974:dbl[])  [unwired: 1 in]
        n1133 = Index Array(array=w1975, index (col)=1 ("Disabled Index (col)")) -> (element=w1973:dbl[])  [unwired: 1 in]
        n1134 = Bundle(w1973, w1974) -> (→"Vel.vs.Loading":cluster{dbl[], dbl[]})  [unwired: 1 out]
      }
      event "ThreatGroups": Value Change {
        n1135 = event-data() -> ()  [unwired: 2 out]
        n1136 = control-ref of="ThreatGroups"() -> (w1984:refnum<vi>)
        n1137 = property on="Property Node" class="Ring (strict)"(reference=w1984, error in=w1983) -> (error out=w1981:errorcluster, "RingText.Text"=w1979:string)  [unwired: 1 out]
        n1138 = Not Equal?(x=w1979, y="") -> (x != y?=w1978:bool)
        n1139 = case shown="True" w1978 {
          tunnel: w1979 -> [_ w1994]
          tunnel: [w1986 w1992] -> w1982
          tunnel: w1981 -> [w1989 w1991]
          frame False {
            n1140 = property on="ThreatDetails" class="Ring (strict)"(error in=w1989, "Strings []"=string[] [], "Value"=u16 0 ("Value (Signaling)")) -> (error out=w1987:errorcluster)  [unwired: 1 in, 1 out]
            n1141 = invoke on="threatDetails" class="Clust (strict)" method="Reinit To Default"(error in=w1987) -> (error out=w1986:errorcluster)  [unwired: 2 in, 2 out]
          }
          frame True {
            n1142 = call "Select Threat Details.vi"("threatGroup"=w1994) -> ("threatDetails"=w1993:string[])  [unwired: 1 out]
            n1143 = property on="ThreatDetails" class="Ring (strict)"(error in=w1991, "Strings []"=w1993, "Val(Sgnl)"=u16 0 ("Value (Signaling)")) -> (error out=w1992:errorcluster)  [unwired: 1 in, 1 out]
          }
        }
      }
      event "panelSearch": Value Change {
        # "This section returns past panels"
        n1144 = event-data() -> ()  [unwired: 2 out]
        n1145 = control-ref of="pastPanels"() -> (w2011:refnum<vi>)
        n1146 = control-ref of="Mfr_0"() -> (w2005:refnum<vi>)
        n1147 = control-ref of="SampleStyle_0"() -> (w2006:refnum<vi>)
        n1148 = control-ref of="Requestors_0"() -> (w2004:refnum<vi>)
        n1149 = control-ref of="ThreatSize_0"() -> (w2003:refnum<vi>)
        n1150 = call "queryPanels (SubVI).vi"("ThreatSize_0"=w2003, "Mfr_0"=w2005, "Requestors_0"=w2004, "Style_0"=w2006, "error in"=w2009, "srchParams"="srchParams", "pastPanels"=w2011) -> ("error out"=w2008:errorcluster, "recordset data"=w2002:string[][], "actualNumPanels"=→"actualNumPanels":i32)  [unwired: 2 in]
        "pastPanels" <- w2002
        n1151 = Index Array(array=w2002) -> (element=w1996:string[])  [unwired: 2 in]
        n1152 = Array Size(array=w1996) -> (size(s)=w2001:i32)
        n1153 = Greater Than 0?(x=w2001) -> (x > 0?=w2000:bool)
        n1154 = Select(t=T15."Enabled" ("Disabled"), s=w2000, f=T15."Disabled and Grayed Out" ("Disabled")) -> (s? t:f=w1999:T15)
        n1155 = property on="reportV50_History" class="Bool"("DisabledEnum"=w1999) -> ()  [unwired: 2 in, 2 out]
      }
      event "pastPanels": Mouse Up {
        n1156 = event-data() -> ("CtlRef"=w2024:refnum<vi>)  [unwired: 1 out]
        n1157 = property on="Property Node" class="Tbl (strict)"(reference=w2024, error in=w2016) -> (error out=w2015:errorcluster, "Value"=w2023:string[][], "EditPos"=w2022:T39)  [unwired: 1 out]
        n1158 = Unbundle By Name(w2022) -> ("Row"=w2021:i32)
        n1159 = Index Array(array=w2023, index (row)=w2021, index (col)=0 ("disabled index (col)")) -> (element=w2020:string)
        n1160 = Scan From String(input string=w2020, error in=w2015, default 1=1 ("Record #")) -> (error out=w2014:errorcluster, output 1=w2018:i32)  [unwired: 2 in, 2 out]
        n1161 = local write "Record #"(w2018) -> ()
      }
      event "ThreatDetails", "SampleID": Value Change {
        # "A Sample ID is entered"
        # "A range is selected"
        # "A measurement requires the selection of a threat,\nso delay enabling the \"Measure\" tab until a grain wt\nis chosen."
        n1162 = event-data() -> ()  [unwired: 2 out]
        n1163 = control-ref of="ThreatGroups"() -> (w2043:refnum<vi>)
        n1164 = control-ref of="ThreatDetails"() -> (w2040:refnum<vi>)
        n1165 = call "Get Projectile Atributes from ThreatGroupDetail.vi"("error IN"=w2042, "ThreatDetail"=w2040, "ThreatGroup"=w2043) -> ("error out"=w2041:errorcluster, "projectileAttribs"=w2039:T40)  [unwired: 1 out]
        "threatDetails" <- w2039
        n1166 = Unbundle By Name(w2039) -> ("grainSize"=w2032:string)
        n1167 = Equal?(x=w2032, y="") -> (x = y?=w2033:bool)
        n1168 = case shown="False" w2033 {
          tunnel: w2032 -> [w2061 _]
          tunnel: [w2060 u16 0 ("GrainSize")] -> w2038
          frame False {
            # "A grain size is selected"
            n1169 = Scan From String(input string=w2061) -> (output 1=w2060:u16)  [unwired: 3 in, 4 out]
            "GrainSize" <- w2060
          }
          frame True {
            # "A grain size not selected"
          }
        }
        n1170 = Equal?(x=w2032, y="") -> (x = y?=w2058:bool)
        n1171 = local read "rangeSetup"() -> (w2055:u16)
        n1172 = case shown="False" w2058 {
          tunnel: [w2065 sgl 0.0] -> w2054
          tunnel: w2032 -> [w2063 _]
          frame False {
            w2067 = sgl 0.0  # sgl
            n1173 = Scan From String(format string="%f " ("Format String"), input string=w2063, default 1=w2067) -> (output 1=w2066:sgl)  [unwired: 2 in, 3 out]
            n1174 = disable-structure shown="Enabled" {
              disable-tunnel: w2066 -> [w2070 w2071]
              disable-tunnel: [w2069 w2071] -> w2065
              frame Disabled {
                n1175 = Multiply(x=sgl 0.06479891, y=w2070) -> (x*y=w2069:sgl)
              }
              frame Enabled {
              }
            }
          }
          frame True {
          }
        }
        "Projectile Mass" <- w2054
        n1176 = local read "SampleID"() -> (w2037:string)
        n1177 = Greater Than 0?(x=w2055) -> (x > 0?=w2056:bool)
        n1178 = Greater Than 0?(x=w2038) -> (x > 0?=w2057:bool)
        n1179 = Not Equal?(x=w2037, y="") -> (x != y?=w2035:bool)
        n1180 = Compound Arithmetic op=AND(w2057, w2056, w2035) -> (w2030:bool)
        n1181 = property on="mainTabCntrl" class="TabCtl (strict)"(error in=w2041) -> (error out=w2047:errorcluster, "Pages"=w2050:refnum<vi>[])  [unwired: 1 in, 1 out]
        n1182 = Not(x=w2030) -> (.not. x?=w2046:bool)
        n1183 = Index Array(array=w2050, index=1) -> (element=w2048:refnum<vi>)
        n1184 = Select(t=T16."Page Enabled" ("Page Enabled State"), s=w2030, f=T16."Page Disabled & Grayed" ("Page Enabled State")) -> (s? t:f=w2029:T16)
        n1185 = property on="Property Node" class="Page"(reference=w2048, error in=w2047, "PageEnb"=w2029) -> (error out=w2045:errorcluster)  [unwired: 1 out]
        n1186 = Select(t=T15."Enabled" ("Disabled"), s=w2030, f=T15."Disabled and Grayed Out" ("Disabled")) -> (s? t:f=w2027:T15)
        n1187 = property on="ARM" class="Bool"(error in=w2045, "Disabled"=w2027) -> (error out=w2053:errorcluster)  [unwired: 1 in, 1 out]
        n1188 = property on="addShot" class="Bool"(error in=w2053, "Disabled"=w2027) -> (error out=w2052:errorcluster)  [unwired: 1 in, 1 out]
        n1189 = property on="instruct_addShot" class="Str"(error in=w2052, "Visible"=w2046) -> (error out=w2051:errorcluster)  [unwired: 1 in, 1 out]
      }
      event "Mfr_1", "Mfr_2", "Mfr_3", "Mfr_4", "Mfr_5", "Mfr_6", "Mfr_0": Value Change {
        n1190 = event-data() -> ("CtlRef"=w2089:refnum<vi>)  [unwired: 1 out]
        n1191 = property on="Property Node" class="Ring (strict)"(reference=w2089, error in=w2081) -> (error out=w2079:errorcluster, "Label.Text"=w2085:string, "RingText.Text"=w2086:string)  [unwired: 1 out]
        n1192 = flat-sequence {
          tunnel: ["Mfr_1"] -> _
          tunnel: ["Mfr_2"] -> _
          tunnel: ["Mfr_3"] -> _
          tunnel: ["Mfr_4"] -> _
          tunnel: ["Mfr_5"] -> _
          tunnel: ["Mfr_6"] -> _
          frame #0 {
          }
        }
        n1193 = call "Select Sample Style.vi"("error IN"=w2079, "Mfr"=w2086) -> ("error Out"=w2078:errorcluster, "SampleStyles"=w2074:string[])  [unwired: 4 out]
        n1194 = Scan From String(format string="Mfr_%d", input string=w2085, error in=w2078, default 1=0 ("Mfr#")) -> (error out=w2075:errorcluster, output 1=w2084:i32)  [unwired: 1 in, 2 out]
        n1195 = case shown="1" w2084 {
          tunnel: [w2101 w2104 w2107 w2110 w2113 w2116 w2119] -> w2083
          tunnel: [w2100 w2103 w2106 w2109 w2112 w2115 w2118] -> w2076
          tunnel: w2075 -> [w2100 w2103 w2106 w2109 w2112 w2115 w2118]
          tunnel: w2074 -> [w2099 w2102 w2105 w2108 w2111 w2114 w2117]
          tunnel: [w2098 w2102 w2105 w2108 w2111 w2114 w2117] -> w2073
          frame 0, Default {
            n1196 = Delete From Array(array=w2099, length=1, index=0) -> (array with subset deleted=w2098:string[])  [unwired: 1 out]
            n1197 = control-ref of="SampleStyle_0"() -> (w2101:refnum<vi>)
          }
          frame 1 {
            n1198 = control-ref of="SampleStyle_1"() -> (w2104:refnum<vi>)
          }
          frame 2 {
            n1199 = control-ref of="SampleStyle_2"() -> (w2107:refnum<vi>)
          }
          frame 3 {
            n1200 = control-ref of="SampleStyle_3"() -> (w2110:refnum<vi>)
          }
          frame 4 {
            n1201 = control-ref of="SampleStyle_4"() -> (w2113:refnum<vi>)
          }
          frame 5 {
            n1202 = control-ref of="SampleStyle_5"() -> (w2116:refnum<vi>)
          }
          frame 6 {
            n1203 = control-ref of="SampleStyle_6"() -> (w2119:refnum<vi>)
          }
        }
        n1204 = property on="Property Node" class="Ring (strict)"(reference=w2083, error in=w2076, "Strings []"=w2073, "Val(Sgnl)"=u16 0 ("Value (Signaling)")) -> (error out=w2080:errorcluster)  [unwired: 1 out]
      }
      event "SampleStyle_1", "SampleStyle_2", "SampleStyle_3", "SampleStyle_4", "SampleStyle_5", "SampleStyle_6", "SampleStyle_0": Value Change {
        n1205 = event-data() -> ("CtlRef"=w2130:refnum<vi>)  [unwired: 1 out]
        n1206 = call "Get Sample Style Atributes.vi"("StyleNumRef"=w2130) -> ("SampleSpecs"=w2125:T41)  [unwired: 1 in]
        n1207 = flat-sequence {
          tunnel: ["SampleStyle_1"] -> _
          tunnel: ["SampleStyle_2"] -> _
          tunnel: ["SampleStyle_3"] -> _
          tunnel: ["SampleStyle_4"] -> _
          tunnel: ["SampleStyle_5"] -> _
          tunnel: ["SampleStyle_6"] -> _
          frame #0 {
          }
        }
        n1208 = property on="Property Node" class="Ring (strict)"(reference=w2130, error in=w2124) -> (error out=w2123:errorcluster, "Label.Text"=w2129:string)  [unwired: 1 out]
        n1209 = Scan From String(format string="SampleStyle_%d", input string=w2129, error in=w2123, default 1=0 ("default value 1")) -> (error out=w2122:errorcluster, output 1=w2127:i32)  [unwired: 1 in, 2 out]
        n1210 = case shown="0, Default" w2127 {
          tunnel: w2125 -> [w2139 w2142 w2145 w2148 w2151 w2154 w2157]
          tunnel: w2122 -> [w2138 w2141 w2144 w2147 w2150 w2153 w2156]
          tunnel: [w2137 w2140 w2143 w2146 w2149 w2152 w2155] -> w2121
          frame 0, Default {
            n1211 = property on="SampleAttribs_0" class="Clust (strict)"(error in=w2138, "Val(Sgnl)"=w2139) -> (error out=w2137:errorcluster)  [unwired: 1 in, 1 out]
            "SampleAttribs_0" <- w2139
          }
          frame 1 {
            n1212 = property on="SampleAttribs_1" class="Clust (strict)"(error in=w2141, "Val(Sgnl)"=w2142) -> (error out=w2140:errorcluster)  [unwired: 1 in, 1 out]
            "SampleAttribs_1" <- w2142
          }
          frame 2 {
            n1213 = property on="SampleAttribs_2" class="Clust (strict)"(error in=w2144, "Val(Sgnl)"=w2145) -> (error out=w2143:errorcluster)  [unwired: 1 in, 1 out]
            "SampleAttribs_2" <- w2145
          }
          frame 3 {
            n1214 = property on="SampleAttribs_3" class="Clust (strict)"(error in=w2147, "Val(Sgnl)"=w2148) -> (error out=w2146:errorcluster)  [unwired: 1 in, 1 out]
            "SampleAttribs_3" <- w2148
          }
          frame 4 {
            n1215 = property on="SampleAttribs_4" class="Clust (strict)"(error in=w2150, "Val(Sgnl)"=w2151) -> (error out=w2149:errorcluster)  [unwired: 1 in, 1 out]
            "SampleAttribs_4" <- w2151
          }
          frame 5 {
            n1216 = property on="SampleAttribs_5" class="Clust (strict)"(error in=w2153, "Val(Sgnl)"=w2154) -> (error out=w2152:errorcluster)  [unwired: 1 in, 1 out]
            "SampleAttribs_5" <- w2154
          }
          frame 6 {
            n1217 = property on="SampleAttribs_6" class="Clust (strict)"(error in=w2156, "Val(Sgnl)"=w2157) -> (error out=w2155:errorcluster)  [unwired: 1 in, 1 out]
            "SampleAttribs_6" <- w2157
          }
        }
      }
      event "SHOTS", "Sort by AVG": Value Change {
        n1218 = event-data() -> ()  [unwired: 2 out]
        n1219 = local read "Site"() -> (w2158:string)
        n1220 = local read "SHOTS"() -> (w2160:T7[])
        n1221 = call "Update Shot Table.vi"("Sort by AVG"="Sort by AVG", "Site"=w2158, "shotsArr"=w2160) -> ("shotTable OUT"=→"Table of Shots":string[][])
      }
      event "Layer_1.plyNum", "Layer_2.plyNum", "Layer_3.plyNum", "Layer_4.plyNum", "Layer_5.plyNum", "Layer_6.plyNum", "SampleAttribs_1.ozPerYd2", "SampleAttribs_2.ozPerYd2", "SampleAttribs_3.ozPerYd2", "SampleAttribs_4.ozPerYd2", "SampleAttribs_5.ozPerYd2", "SampleAttribs_6.ozPerYd2": Value Change {
        n1222 = event-data() -> ()  [unwired: 2 out]
        n1223 = global read "BIMS_Collector Globals.vi" "SampleAttribs"() -> (w2164:T24)
        n1224 = Build Array("Layer_1", "Layer_2", "Layer_3", "Layer_4", "Layer_5", "Layer_6") -> (w2167:T42)
        n1225 = global write "BIMS_Collector Globals.vi" "LayerSpecs"(w2167) -> ()
        n1226 = for {
          tunnel: w2167 -> [w2194] mode=indexing
          shift-right: [w2196] -> w2175
          shift-left: 0 -> [w2195]
          tunnel: [w2193] -> w2185 mode=indexing
          tunnel: w2164 -> [w2191] mode=indexing
          n1227 = Unbundle By Name(w2191) -> ("ozPerYd2"=w2187:string)
          n1228 = Equal?(x=w2187, y="" ("Empty String Constant")) -> (x = y?=w2186:bool)
          n1229 = case shown="False" w2186 {
            tunnel: [w2200 sgl 0.0 ("default value 1")] -> w2190
            tunnel: w2187 -> [w2197 _]
            frame False {
              n1230 = Scan From String(format string="%f", input string=w2197, default 1=sgl 0.0 ("default value 1")) -> (output 1=w2200:sgl)  [unwired: 2 in, 3 out]
            }
            frame True {
            }
          }
          n1231 = Unbundle By Name(w2194) -> ("plyNum"=w2192:i32)
          n1232 = Add(x=w2195, y=w2192) -> (x+y=w2196:i32)
          n1233 = To Single Precision Float(number=w2192) -> (single precision float=w2189:sgl)
          n1234 = Multiply(x=w2189, y=w2190) -> (x*y=w2193:sgl)
        }
        "totalNumLayers" <- w2175
        n1235 = Divide(x=w2185, y=sgl 144.0) -> (x/y=w2183:sgl[])
        n1236 = Index Array(array=w2183) -> (element #1=→"fab1_totalWt":sgl, element #2=→"fab2_totalWt":sgl, element #3=→"fab3_totalWt":sgl, element #4=→"fab4_totalWt":sgl, element #5=→"fab5_totalWt":sgl, element #6=→"fab6_totalWt":sgl)  [unwired: 6 in]
        n1237 = Add Array Elements(numeric array=w2183) -> (sum=→"totalBAW":sgl)
      }
      event "clayCalArray": Value Change {
        n1238 = event-data() -> ()  [unwired: 2 out]
        n1239 = for {
          tunnel: "clayCalArray" -> [w2229] mode=indexing
          shift-right: [w2228] -> w2211
          shift-left: "" ("Empty String Constant") -> [w2226]
          shift-right: [w2223] -> w2207
          shift-left: i16[] [] -> [w2222]
          n1240 = Greater Than 0?(x=w2229) -> (x > 0?=w2230:bool)
          n1241 = case shown="False" w2230 {
            tunnel: w2229 -> [_ w2236]
            tunnel: ["##" ("clayCalib") w2238] -> w2227
            tunnel: w2226 -> [w2233 w2237]
            tunnel: [w2233 w2237] -> w2225
            tunnel: [w2231 w2235] -> w2223
            tunnel: w2222 -> [w2231 w2234]
            frame False {
            }
            frame True {
              n1242 = Format Into String(w2236) -> (resulting string=w2238:string)  [unwired: 3 in, 1 out]
              n1243 = Build Array (concatenate)(w2234, w2236) -> (w2235:i16[])
            }
          }
          n1244 = Concatenate Strings(w2225, w2227, "-" ("string")) -> (w2228:string)
        }
        n1245 = String Length(string=w2211) -> (length=w2212:i32)
        n1246 = Add Array Elements(numeric array=w2207) -> (sum=w2216:i16)
        n1247 = Array Size(array=w2207) -> (size(s)=w2217:i32)
        n1248 = Decrement(x=w2212) -> (x-1=w2209:i32)
        n1249 = To Single Precision Float(number=w2216) -> (single precision float=w2215:sgl)
        n1250 = To Single Precision Float(number=w2217) -> (single precision float=w2205:sgl)
        n1251 = String Subset(string=w2211, length (rest)=w2209) -> (substring=w2210:string)  [unwired: 1 out]
        n1252 = Equal To 0?(x=w2205) -> (x = 0?=w2204:bool)
        n1253 = local write "clayCalib"(w2210) -> ()
        n1254 = case shown="True" w2204 {
          tunnel: w2215 -> [w2220 w2221]
          tunnel: w2205 -> [w2219 _]
          tunnel: [w2218 w2221] -> w2214
          frame False {
            n1255 = Divide(x=w2220, y=w2219) -> (x/y=w2218:sgl)
          }
          frame True {
          }
        }
        "clayAverage" <- w2214
      }
      event "reportV50_History": Value Change {
        n1256 = event-data() -> ()  [unwired: 2 out]
        n1257 = local write "lookupRec"(TRUE ("lookupRec")) -> ()
      }
      event "Methods": Value Change {
        n1258 = event-data() -> ("CtlRef"=w2248:refnum<vi>)  [unwired: 1 out]
        n1259 = call "Dropdown Selection (SubVI).vi"("reference"=w2248) -> ("element"=w2247:string)
        n1260 = Equal?(x=w2247, y="V50") -> (x = y?=w2245:bool)
        n1261 = property on="minV50" class="DigNum (strict)"(error in=w2244, "Visible"=w2245) -> (error out=w2243:errorcluster)  [unwired: 1 in, 1 out]
      }
      event "rangeSetup": Value Change {
        n1262 = event-data() -> ("NewVal"=w2258:u16)  [unwired: 1 out]
        n1263 = case shown="2" w2258 {
          tunnel: ["0" ("section") "5.0" ("section") "7.5" ("section") "45.0" ("section")] -> w2264
          frame 0, Default {
          }
          frame 1 {
          }
          frame 2 {
          }
          frame 3 {
          }
        }
        n1264 = local read "configPath"() -> (w2266:path)
        n1265 = local read "GrainSize"() -> (w2257:u16)
        n1266 = Greater Than 0?(x=w2258) -> (x > 0?=w2261:bool)
        n1267 = Greater Than 0?(x=w2257) -> (x > 0?=w2259:bool)
        n1268 = call <vilib>:"Open Config Data (compatibility).vi"("error in (no error)"=w2254, "configuration file path"=w2266) -> ("error out"=w2274:errorcluster, "refnum"=w2276:T36)  [unwired: 7 in, 1 out]
        n1269 = And(x=w2261, y=w2259) -> (x .and. y?=w2260:bool)
        n1270 = call-poly <vilib>:"Write Key.vi"("write raw string? (F)"=TRUE, "section"="Ballistic Parameters", "error in (no error)"=w2274, "value"=w2264, "key"="MidPoint To Target Distance", "refnum"=w2276) -> ("error out"=w2273:errorcluster, "refnum out"=w2272:T36)  [unwired: 4 out]
        n1271 = call <vilib>:"Close Config Data.vi"("error in (no error)"=w2273, "refnum"=w2272) -> ("error out"=w2265:errorcluster)  [unwired: 1 in, 8 out]
        n1272 = Not(x=w2260) -> (.not. x?=w2270:bool)
        n1273 = Select(t=u8 0 ("y"), s=w2260, f=u8 2 ("y")) -> (s? t:f=w2256:u8)
        n1274 = Scan From String(input string=w2264, error in=w2265, default 1=sgl 0.0 ("default value 1")) -> (error out=w2253:errorcluster, output 1=w2263:sgl)  [unwired: 2 in, 2 out]
        n1275 = local write "mid_to_targ_dist"(w2263) -> ()
        n1276 = property on="ARM" class="Bool"(error in=w2253, "Disabled"=w2256) -> (error out=w2252:errorcluster)  [unwired: 1 in, 1 out]
        n1277 = property on="addShot" class="Bool"(error in=w2252, "Disabled"=w2256) -> (error out=w2251:errorcluster)  [unwired: 1 in, 1 out]
        n1278 = property on="instruct_addShot" class="Str"(error in=w2251, "Visible"=w2270) -> (error out=w2250:errorcluster)  [unwired: 1 in, 1 out]
        "instruct_addShot" <- "RANGE SETUP and THREAT must be selected before shots can be added." ("instruct_addShot")
      }
      event "Drag Corrected", "maxDev": Value Change {
        n1279 = event-data() -> ()  [unwired: 2 out]
        n1280 = local write "processShots"(TRUE ("ProcessShots")) -> ()
      }
      event "MC Listbox of Shots": Mouse Up {
        n1281 = event-data() -> ()  [unwired: 2 out]
        n1282 = flat-sequence {
          tunnel: w2289 -> [w2293]
          tunnel: [w2291] -> w2288
          tunnel: ["MC Listbox of Shots"] -> w2285
          tunnel: w2288 -> [w2297]
          tunnel: [w2296] -> w2287
          tunnel: w2285 -> [_]
          tunnel: w2287 -> [w2302]
          tunnel: [w2300] -> w2286
          frame #0 {
            n1283 = property on="Table of Shots" class="Tbl (strict)"(error in=w2293) -> (error out=w2292:errorcluster, "Value"=w2294:string[][])  [unwired: 1 in, 1 out]
            n1284 = local write "STOP (Shots MC LB)"(FALSE ("STOP (Shots MC LB)")) -> ()
            n1285 = property on="MC Listbox of Shots" class="MCListbox (strict)"(error in=w2292, "ItemNames"=w2294) -> (error out=w2291:errorcluster)  [unwired: 1 in, 1 out]
          }
          frame #1 {
            n1286 = control-ref of="MC Listbox of Shots"() -> (w2299:refnum<vi>)
            n1287 = control-ref of="STOP (Shots MC LB)"() -> (w2298:refnum<vi>)
            n1288 = call "multicolumn listbox sort.vi"("error IN"=w2297, "Bool Refnum"=w2298, "MCListbox Refnum"=w2299) -> ("error out"=w2296:errorcluster)  [unwired: 4 in]
          }
          frame #2 {
            n1289 = property on="MC Listbox of Shots" class="MCListbox (strict)"(error in=w2302) -> (error out=w2301:errorcluster, "ItemNames"=w2303:string[][])  [unwired: 1 in, 1 out]
            n1290 = property on="Table of Shots" class="Tbl (strict)"(error in=w2301, "Val(Sgnl)"=w2303) -> (error out=w2300:errorcluster)  [unwired: 1 in, 1 out]
          }
        }
      }
      event "PublishNewRecords": Value Change {
        w2309 = "\\" ("string")
        w2320 = TRUE  # overwrite (F)
        # "2. INSERT new records to Experiments and  \n      Shots tables in local Export.mdb file."
        # "1. SELECT new records from local MDB \n     by comparing against last record numbers \n     found in IMPORT table on BIMS server."
        # "Pushes latest ballistics performance data up to BIMS Server\n\n - Attempts connection with server (reports connection success in msgbox)\n - If successful:\n   - Exports all experiment/shot records since last table marker to [site].mdb file\n   - Sends export.mdb file to drop location on BIMS File Server\n   - Executes SSIS package to import records from export.mdb file\n - Otherwise provides option to try again or cancel"
        # "3. Copy Export.mdb file to [sitename].mdb in [sitename] \n      FileDrop folder on BIMS server."
        n1291 = event-data() -> ()  [unwired: 2 out]
        n1292 = property on="Loading" class="Ring (strict)"(error in=w2315, "Visible"=TRUE) -> (error out=w2314:errorcluster)  [unwired: 1 in, 1 out]
        n1293 = local read "Site"() -> (w2304:string)
        n1294 = call "Export New Records.vi"("error IN"=w2314, "Site"=w2304) -> ("error out"=w2322:errorcluster)  [unwired: 3 in, 6 out]
        n1295 = Concatenate Strings("\\\\" ("string"), "Server", w2309, "Folder", w2309, w2304, ".mdb" ("string")) -> (w2305:string)
        n1296 = String To Path(string=w2305) -> (path=w2318:path)
        n1297 = Copy(8:w2322, 9:w2320, 10:w2318, 11:path "C:/Ballistics/Export.mdb" ("source path")) -> (0:w2319:errorcluster)  [unwired: 3 out]
        n1298 = case shown="No Error" w2319 {
          selector: w2319 -> [w2324 w2326]
          tunnel: [w2324 w2325] -> w2313
          frame No Error {
            n1299 = One Button Dialog(message="New sample performance records submitted \nto BIMS Warehouse successfully.\n\nPublishing will occur in under five minutes.") -> ()  [unwired: 2 out]
          }
          frame Error {
            n1300 = call <vilib>:"General Error Handler.vi"("error in (no error)"=w2326) -> ("error out"=w2325:errorcluster)  [unwired: 2 in, 12 out]
          }
        }
        n1301 = property on="Loading" class="Ring (strict)"(error in=w2313, "Visible"=FALSE) -> (error out=w2312:errorcluster)  [unwired: 1 in, 1 out]
      }
      event "arrIDC": Mouse Up {
        n1302 = event-data() -> ()  [unwired: 2 out]
        "velProfile" <- cluster{dbl, dbl}[] [] ("velProfile")
        "arrIDC" <- dbl[] [] ("arrIDC")
        "relativeTime" <- cluster{"ts2":dbl, "ts3":dbl, "ts1":dbl} {"ts2"=0.0, "ts3"=0.0, "ts1"=0.0} ("relativeTime")
        "velMeasProf" <- T8 {"v2"=0.0, "vB"=0.0, "vOuter"=0.0, "v1"=0.0, "vA"=0.0, "vInner"=0.0} ("velMeasProf")
        "velCompProf" <- cluster{"vStrike":dbl, "vA":dbl} {"vStrike"=0.0, "vA"=0.0} ("velCompProf")
        "displacement" <- T9 {"ds_v2"=6.75, "ds2"=5.0833, "ds_vB"=4.9167, "ds3"=4.75, "ds_vAvg"=6.9167, "ds_v1"=7.0833, "ds1"=8.75, "ds_vA"=8.9167, "ds0"=9.0833} ("displacement")
      }
      event "SampleBackings": Value Change {
        # "Clay is the default sample backing material.\n\n  If another selection is made, then grey out and disable all controls relating to clay."
        n1303 = event-data() -> ()  [unwired: 2 out]
        n1304 = case shown="0, Default" "SampleBackings" {
          tunnel: [T15."Disabled and Grayed Out" ("Disabled") T15."Enabled" ("Disabled") T15."Disabled and Grayed Out" ("Disabled")] -> w2335
          frame 0, Default {
          }
          frame 1 {
          }
          frame 2.. {
          }
        }
        n1305 = property on="clayCalArray" class="Arr (strict)"("DisabledEnum"=w2335) -> ()  [unwired: 2 in, 2 out]
        n1306 = property on="clayAverage" class="DigNum (strict)"("DisabledEnum"=w2335) -> ()  [unwired: 2 in, 2 out]
        n1307 = property on="clayTemp" class="DigNum (strict)"("DisabledEnum"=w2335) -> ()  [unwired: 2 in, 2 out]
      }
      event "RefreshMetadata": Value Change {
        # "Pulls latest metadata down from BIMS Database Server\n - Attempts connection with server \n        (reports failure if connection is unsuccessful)\n - If successful:\n   - Updates local database records from server\n   - Updates dropdown listboxes from local database"
        n1308 = event-data() -> ()  [unwired: 2 out]
        n1309 = property on="Loading" class="Ring (strict)"(error in=w2365, "Visible"=TRUE) -> (error out=w2364:errorcluster)  [unwired: 1 in, 1 out]
        n1310 = control-ref of="LayerStitchTypes"() -> (w2349:refnum<vi>)
        n1311 = control-ref of="BackLayer"() -> (w2360:refnum<vi>)
        n1312 = control-ref of="FrontLayer"() -> (w2361:refnum<vi>)
        n1313 = control-ref of="ThreatGroups"() -> (w2362:refnum<vi>)
        n1314 = control-ref of="SampleClamping"() -> (w2370:refnum<vi>)
        n1315 = control-ref of="SampleTypes"() -> (w2387:refnum<vi>)
        n1316 = control-ref of="SampleDimensions"() -> (w2386:refnum<vi>)
        n1317 = control-ref of="ModelMfrs"() -> (w2385:refnum<vi>)
        n1318 = control-ref of="Assemblers"() -> (w2384:refnum<vi>)
        n1319 = control-ref of="Submitters"() -> (w2383:refnum<vi>)
        n1320 = control-ref of="PowderTypes"() -> (w2382:refnum<vi>)
        n1321 = control-ref of="Methods"() -> (w2379:refnum<vi>)
        n1322 = control-ref of="TestConditions"() -> (w2378:refnum<vi>)
        n1323 = control-ref of="SampleBackings"() -> (w2377:refnum<vi>)
        n1324 = control-ref of="Ballisticians"() -> (w2376:refnum<vi>)
        n1325 = control-ref of="Shooters"() -> (w2375:refnum<vi>)
        n1326 = control-ref of="Recorders"() -> (w2374:refnum<vi>)
        n1327 = Build Array(w2349, w2360, w2361, w2362, w2370, w2387, w2386, w2385, w2384, w2383, w2382, w2379, w2378, w2377, w2376, w2375, w2374) -> (w2381:refnum<vi>[])
        n1328 = call "Update Metadata using listbox names.vi"("error in"=w2364, "Site"="Site", "RefNumArrIn"=w2381) -> ("error out"=w2388:errorcluster, "RefNumArrOut"=w2380:refnum<vi>[])  [unwired: 1 in, 6 out]
        n1329 = call "Fill Lists from DB (1st Pass).vi"("error in"=w2388, "RefNumArray"=w2380) -> ("error out"=w2350:errorcluster)  [unwired: 1 in, 4 out]
        n1330 = call "Fill Stitch Lists.vi"("error IN"=w2350) -> ("error OUT"=w2345:errorcluster)  [unwired: 6 in]
        n1331 = control-ref of="ThreatSize_0"() -> (w2343:refnum<vi>)
        n1332 = control-ref of="Requestors_0"() -> (w2348:refnum<vi>)
        n1333 = Build Array(w2343, w2348) -> (w2347:refnum<vi>[])
        n1334 = call "Fill Lists from DB (2nd Pass).vi"("errorIN"=w2345, "colNames"=string[] ["GrainSize", "requestor"] ("lkupTableNames"), "lkupTableNames"=string[] ["ThreatDetails", "Submitters"], "RefNumArray"=w2347) -> ("error OUT"=w2344:errorcluster)  [unwired: 3 in]
        n1335 = flat-sequence {
          frame #0 {
            n1336 = local write "RefreshMetadata"(FALSE ("UpdateMetadata")) -> ()
            n1337 = local write "TimeNow"("Connecting to BIMS Server . . ." ("TimeNow")) -> ()
          }
        }
        n1338 = call "Create local tables from Server DB.vi"("error in"=w2344, "Site"="Site", "tableNames"=string[] ["Threats", "ThreatDetails", "ThreatCalibers", "Mfrs", "SampleStyles", "SampleSpecs", "FiberTypes"]) -> ("error out"=w2372:errorcluster)  [unwired: 1 in, 7 out]
        n1339 = call "Fill Lists From DB (3rd Pass).vi"("error IN"=w2372) -> ("error OUT"=w2352:errorcluster)  [unwired: 3 in, 3 out]
        n1340 = control-ref of="ModelMfrs"() -> (w2359:refnum<vi>)
        n1341 = property class="Ring (strict)"(reference=w2359, error in=w2352) -> (reference out=w2358:refnum<vi>, error out=w2357:errorcluster, "Strings []"=w2356:string[])
        n1342 = Delete From Array(array=w2356, length=1, index=0) -> (array with subset deleted=w2355:string[])  [unwired: 1 out]
        n1343 = property class="Ring (strict)"(reference=w2358, error in=w2357, "Strings []"=w2355) -> (error out=w2351:errorcluster)  [unwired: 1 out]
        n1344 = case shown="No Error" w2351 {
          selector: w2351 -> [w2389 w2392]
          tunnel: [w2389 w2392] -> w2368
          frame No Error {
            n1345 = local write "TimeNow"("Collector Metadata is READY!" ("TimeNow")) -> ()
            n1346 = Wait (ms)(milliseconds to wait=u32 2000) -> ()  [unwired: 1 out]
          }
          frame Error {
            n1347 = call <vilib>:"General Error Handler.vi"("error in (no error)"=w2392) -> ()  [unwired: 2 in, 13 out]
          }
        }
        n1348 = property on="Loading" class="Ring (strict)"(error in=w2368, "Visible"=FALSE) -> (error out=w2367:errorcluster)  [unwired: 1 in, 1 out]
      }
      event "loadingUnits": Value Change {
        n1349 = local read "Powder Loading"() -> (w2396:sgl)
        n1350 = event-data() -> ("NewVal"=w2395:enum32{"grams", "grains"})  [unwired: 6 out]
        n1351 = case shown="\"grams\", Default" w2395 {
          tunnel: w2396 -> [w2401 w2402]
          frame "grams", Default {
            n1352 = Multiply(x=w2401, y=sgl 0.06479891) -> (x*y=w2399:sgl)
            n1353 = local write "Powder Loading"(w2399) -> ()
          }
          frame "grains" {
            n1354 = Multiply(x=w2402, y=sgl 15.432359) -> (x*y=w2403:sgl)
            n1355 = local write "Powder Loading"(w2403) -> ()
          }
        }
      }
      event "clearErrors": Value Change {
        w2405 = errorcluster {"status"=FALSE, "code"=0, "source"=""} ("error in")
        n1356 = event-data() -> ()  [unwired: 7 out]
        n1357 = local write "SMErr"(w2405) -> ()
      }
    }
    "U/I EvErr" <- w1895
    "booleanDump" <- w1894
  }
